vi "RT_SynthFoc.vi"(0 "mode":T4=enum."Full 25 Ch", 2 "Pause?":bool, 3 "Motion Board ID":T6=1 min=1 max=32 step=1, 5 "Scan Axis":u16=3, 8 "Filter":T1, 9 "Qs and Notis":T3, 10 "BKPT Shift":i32, 11 "Raw Name":string="raw", 14 "Trans Geometry (mm)":T2={"Geo Focus"=12.0, "a (radius)"=3.0, "# of rings"=5, "kerf space "=0.1} {"kerf space" format="%.4f"; "a (radius)" format="%.2f"; "Geo Focus" format="%.2f"}) -> (16 "Bd ID Out":T5, 19 "error out":errorcluster)   [LabVIEW 2022 SP3]
uses:
  ScanningControl/Motion Controllers/-MotionRoutines/MotionGlobals.vi
  <vilib>/Motion/FlexMotion/FunctionsVIs/Trajectory.llb/Load Acceleration/Deceleration.flx
  <vilib>/Motion/FlexMotion/CustomControls/CustomControls.llb/Axis To Control.flx
  <vilib>/Motion/FlexMotion/CustomControls/CustomControls.llb/Program.flx
  <instrlib>/niScope/Acquire/Fetch/niScope Multi Fetch Binary 8.vi
  <vilib>/Platform/TimedLoop/XDataNode/XDataNode.xnode
  <vilib>/Platform/TimedLoop/XDataNode/nitl_modes.ctl
  <vilib>/Platform/TimedLoop/XDataNode/XDNodeRunTimeDep.lvlib
  <vilib>/Platform/TimedLoop/XDataNode/wakeup.ctl
  <vilib>/Platform/TimedLoop/XDataNode/timing_clust.ctl
  <vilib>/Motion/FlexMotion/FunctionsVIs/Trajectory.llb/Wait for Move Complete (8 axes).flx
  <vilib>/DAQmx/write.llb/DAQmx Write (Digital 1D Bool NChan 1Samp 1Line).vi
  <vilib>/Motion/FlexMotion/FunctionsVIs/OnboardProgramming.llb/Pause/Resume Program.flx
  RealTimeMode.ctl
  <vilib>/ptbypt/NI_PtbyPt.lvlib
  Annular Array/-SynthApperture/TimeShiftDataI8.vi
  <vilib>/Analysis/NI_AALBase.lvlib
  Annular Array/-SynthApperture/TimeShiftData.vi
  <vilib>/Analysis/baseanly.llb/Mean (DBL).vi
  <instrlib>/niScope/Acquire/niScope Get Scaling Coefficients.vi
  <vilib>/picture/picture.llb/imagedata.ctl
panel:
  out "SF Loop":i32
  out "Read Loop":i32
  out "SF queue":i32
  out "Record queue":i32
  in  "Round to ROC?":bool
  in  "One Way Receive":bool
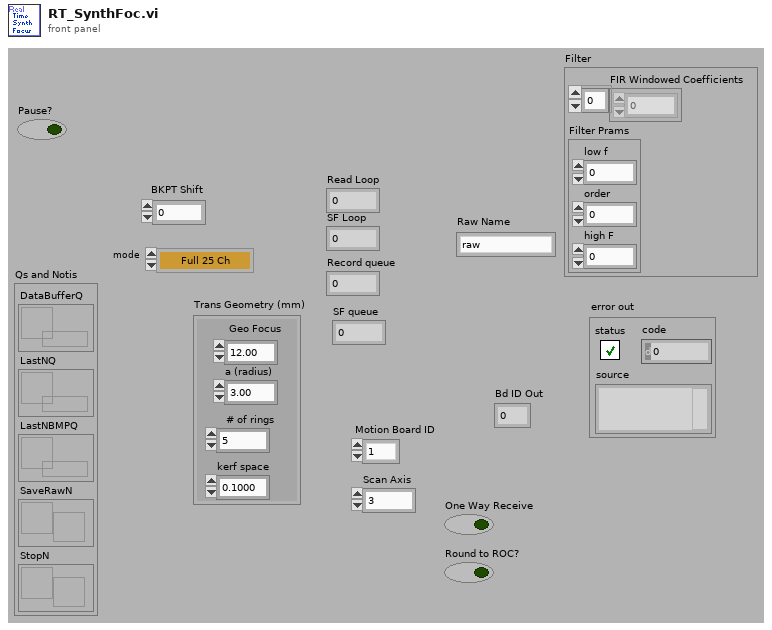
[diagram p1: front panel]
types:
  T1 = cluster{"FIR Windowed Coefficients":dbl[], "Filter Prams":cluster{"low f":i32, "order":i32, "high F":i32}}
  T2 = cluster{"Geo Focus":dbl, "a (radius)":dbl, "# of rings":i32, "kerf space ":dbl}
  T3 = cluster{"DataBufferQ":refnum<queue>, "LastNQ":refnum<queue>, "LastNBMPQ":refnum<queue>, "SaveRawN":refnum<notifier>, "StopN":refnum<notifier>}
  T4 = typedef "RealTimeMode.ctl" = enum16{"1T/5R", "1T/5R Deep Mem", "Full 25 Ch", "Drop Ch 5", "Drop Ch 5,4", "Drop Ch 5,4,3", "Drop Ch 5,4,3,2", "All 25 FIFO CH by CH", "Line by line 2 Ch", "Line by line All", "Deep Memory 2 CH", "Drop Ch 5 (3 Trig)", "test", "Drop Ch 5 XMIT", "Drop Ch 5,4 XMIT", "Drop Ch 5,4,3 XMIT"}
  T5 = typedef "Bd Id Out" = u8
  T6 = typedef "Board Id" = u8
  T7 = cluster{"offset":dbl, "gain":dbl, "reserved 1":dbl, "reserved 2":dbl}[]
  T8 = cluster{"offset":dbl, "gain":dbl, "reserved 1":dbl, "reserved 2":dbl}
  T9 = typedef "location.ctl" = enum16{"Automatic", "WCM Main", "Hawaii", "Columbia MM3000", "Columbia  NI System", "NYU", "RRI 2", "UHI Allen", "CUMC RT", "Chiba", "Stony Brook", "WCM Microscopy", "WCM Aeoretch", "WCM Optics Lab", "WCM Main 2Axis", "WCM Rotation", "WCM SAM SMAC", "SERI GP"}
  T10 = cluster{sgl, "Gain [dB]  ":sgl, "Atten (dB)":sgl}
  T11 = typedef "Program.flx" = u8
  T12 = cluster{"gain":dbl, "wfm":i8[][], bool, "max queue size (-1, unlimited)":i32}
  T13 = typedef "XDNodeRunTimeDep.lvlib/timing_clust.ctl" = cluster{"Expected End [f-1]":u64, "Actual End [f-1]":u64, "Finished Late? [f-1]":bool, "Expected End [i-1]":u64, "Actual End [i-1]":u64, "Finished Late? [i-1]":bool, "Expected Start [i]":u64, "Actual Start [i]":u64, "Expected Start [f]":u64, "Actual Start [f]":u64, "Source Name":string, "Structure Name":string, "Period":i64, "Deadline":i64, "Offset":i64, "Start":i64, "Priority":i32, "Timeout":i32, "Mode":T14, "Wakeup Reason":T15, "Error":errorcluster, "Source Type":string, "Secondary Source Type":string, "Global End Time":u64, "Global Start Time":u64, "Frame Duration":u64, "Iteration Duration":u64, "Assigned CPU":i32, "I/O Scan Engine Mode":u32}
  T14 = typedef "XDNodeRunTimeDep.lvlib/nitl_modes.ctl" = enum32{"No Change", "Process missed periods, maintain original phase", "Discard missed periods, maintain original phase", "Process missed periods, ignore original phase", "Discard missed periods, ignore original phase"}
  T15 = typedef "XDNodeRunTimeDep.lvlib/wakeup.ctl" = enum32{"Normal", "Aborted", "Asynchronous wakeup", "Timing source error", "Timed loop error", "Timeout"}
  T16 = typedef "Axis To Control.flx" = u16
  T17 = cluster{"ZoneStart":sgl[], "ZoneShift":sgl[], "ZoneLength":sgl[]}
  T18 = cluster{"[0]":string, "[1]":string, "[2]":string, "[3]":string, "[4]":string}
  T19 = cluster{"ZoneStart":sgl[], "ZoneShift":sgl[], "ZoneLength":sgl[]}[][]
  T20 = cluster{"ZoneStart":sgl[], "ZoneShift":sgl[], "ZoneLength":sgl[]}[]
  T21 = cluster{"gain":dbl, bool, i16[][], "Sat Pts":i32}
  T22 = cluster{"actualSamples":i32, "absoluteInitialX":dbl, "relativeInitialX":dbl, "xIncrement":dbl, "offset":dbl, "gain":dbl, "reserved1":dbl, "reserved2":dbl}[]
  T23 = cluster{"actualSamples":i32, "absoluteInitialX":dbl, "relativeInitialX":dbl, "xIncrement":dbl, "offset":dbl, "gain":dbl, "reserved1":dbl, "reserved2":dbl}
  T24 = cluster{"gain":dbl, "wfm":i8[][], "Reverse?":bool, i32}
  T25 = cluster{"dig gain":dbl, "Array":i8[][], "Reverse?":bool, i32}
  T26 = cluster{"dig gain":dbl, "Array":i8[][], "Reverse?":bool}
  T27 = typedef "Resource Out (Enum).flx" = u16
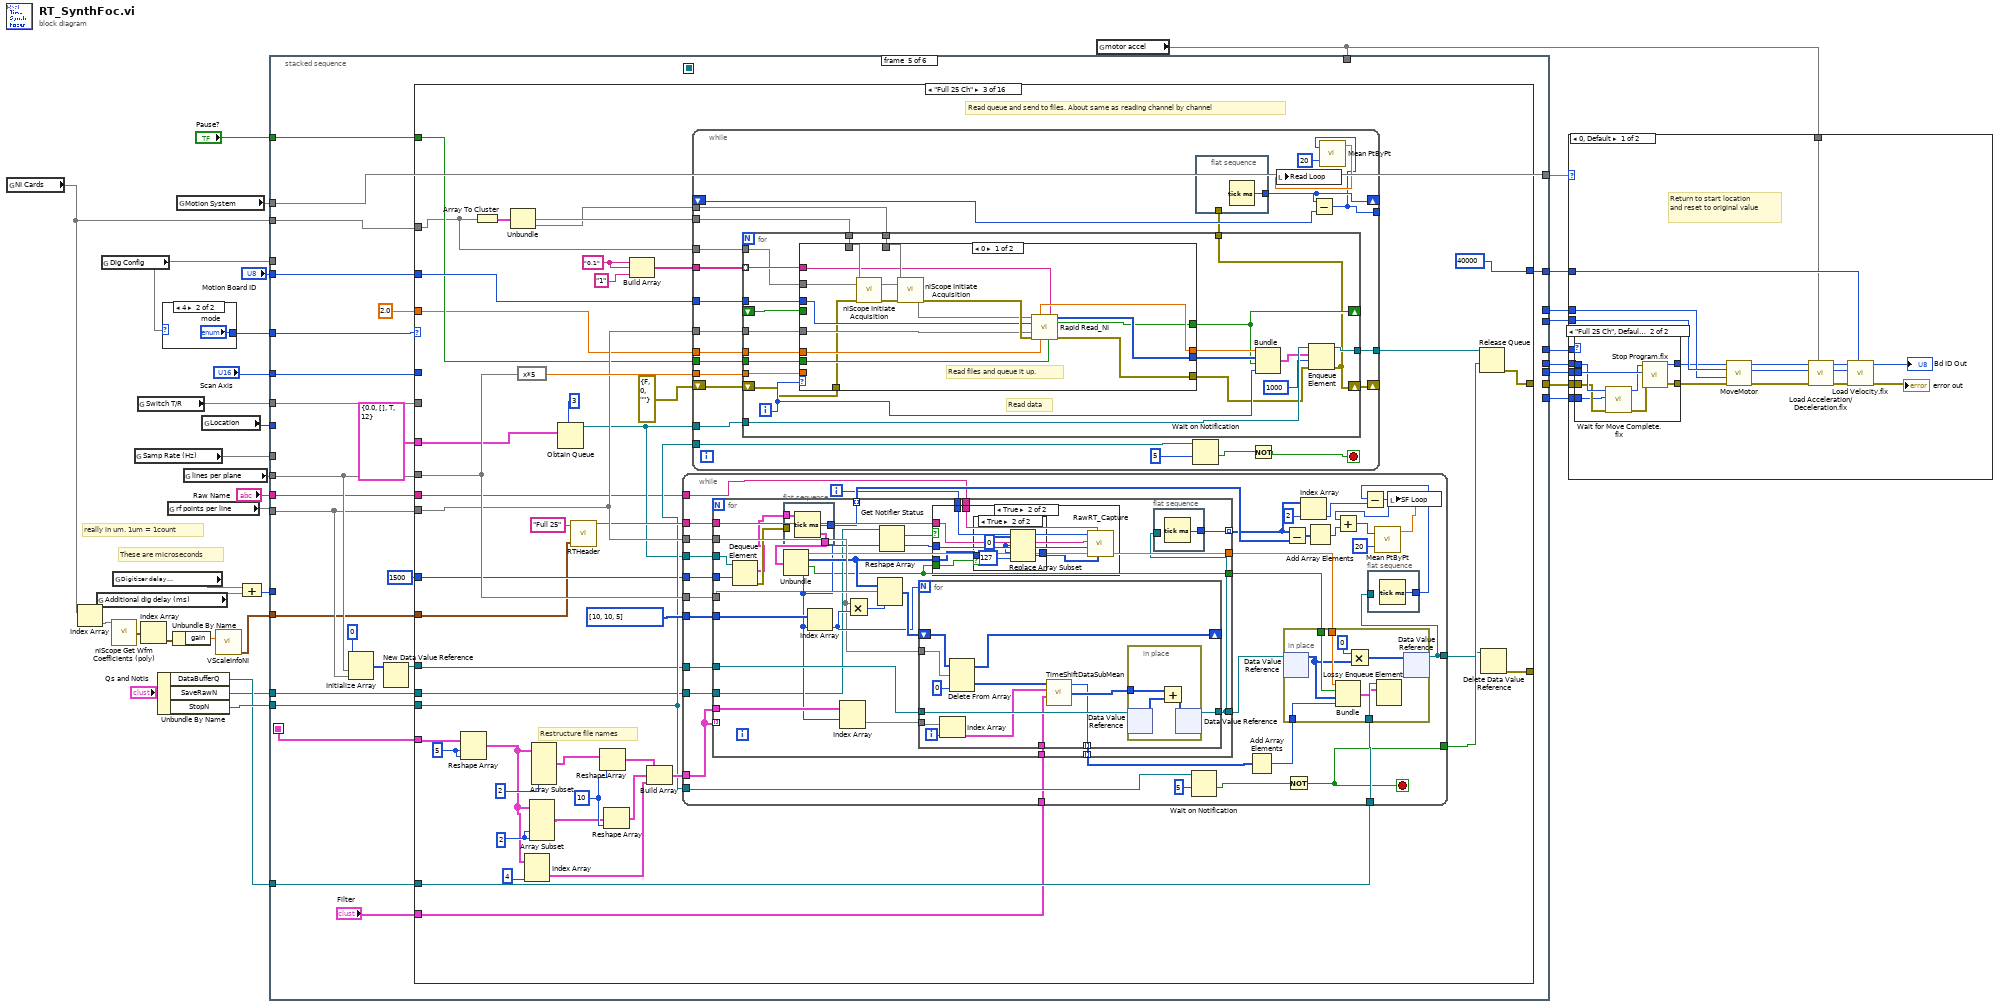
[diagram p0: block diagram]
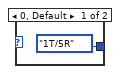
[diagram p4: hidden frame]
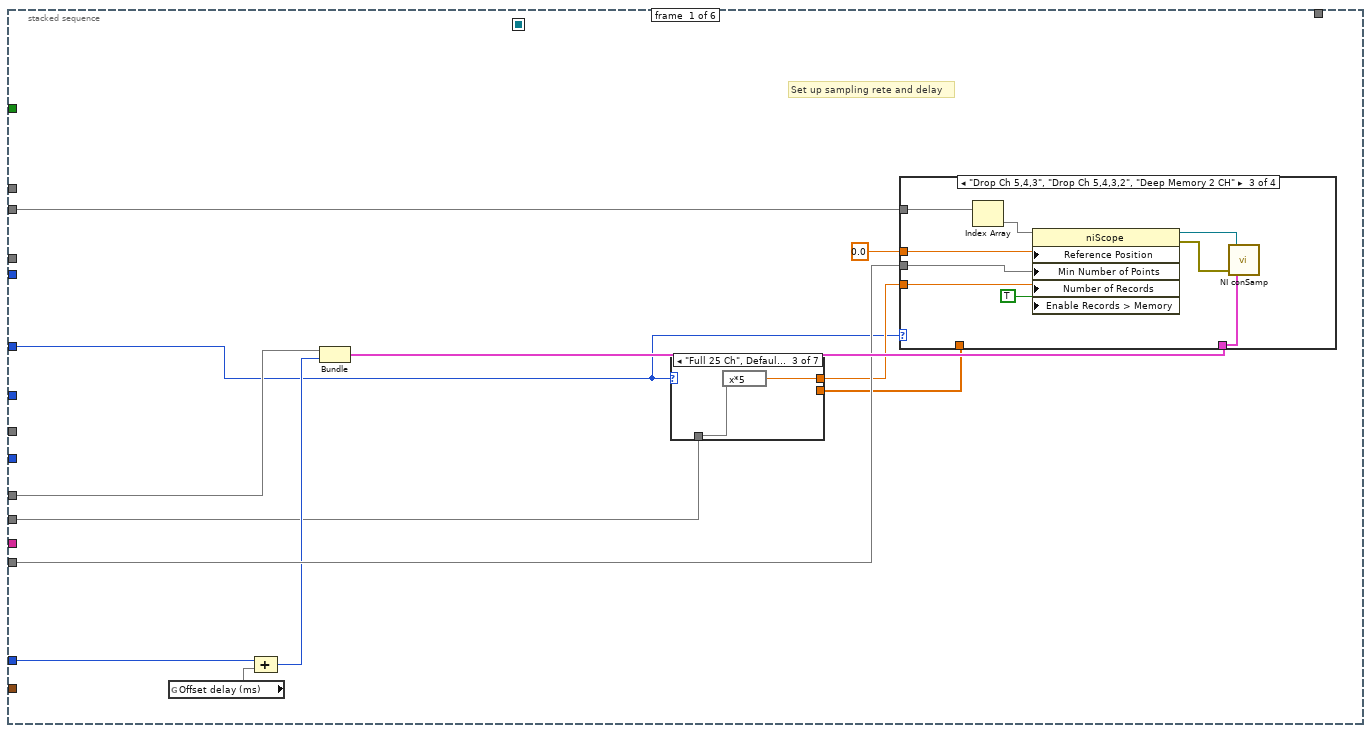
[diagram p5: hidden frame]
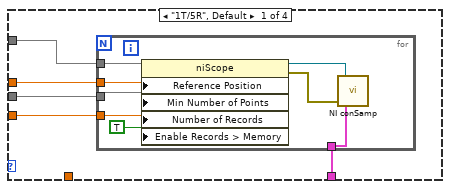
[diagram p6: hidden frame]
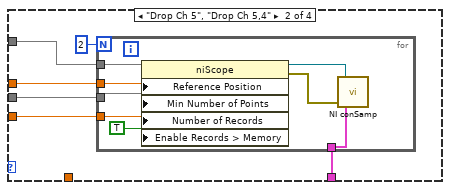
[diagram p7: hidden frame]
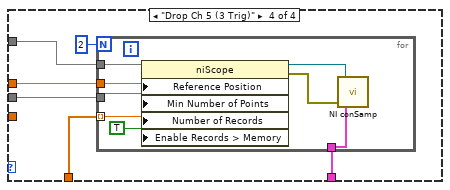
[diagram p8: hidden frame]
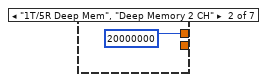
[diagram p10: hidden frame]
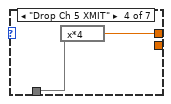
[diagram p11: hidden frame]
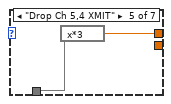
[diagram p12: hidden frame]
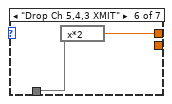
[diagram p13: hidden frame]
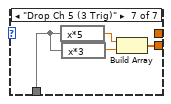
[diagram p14: hidden frame]
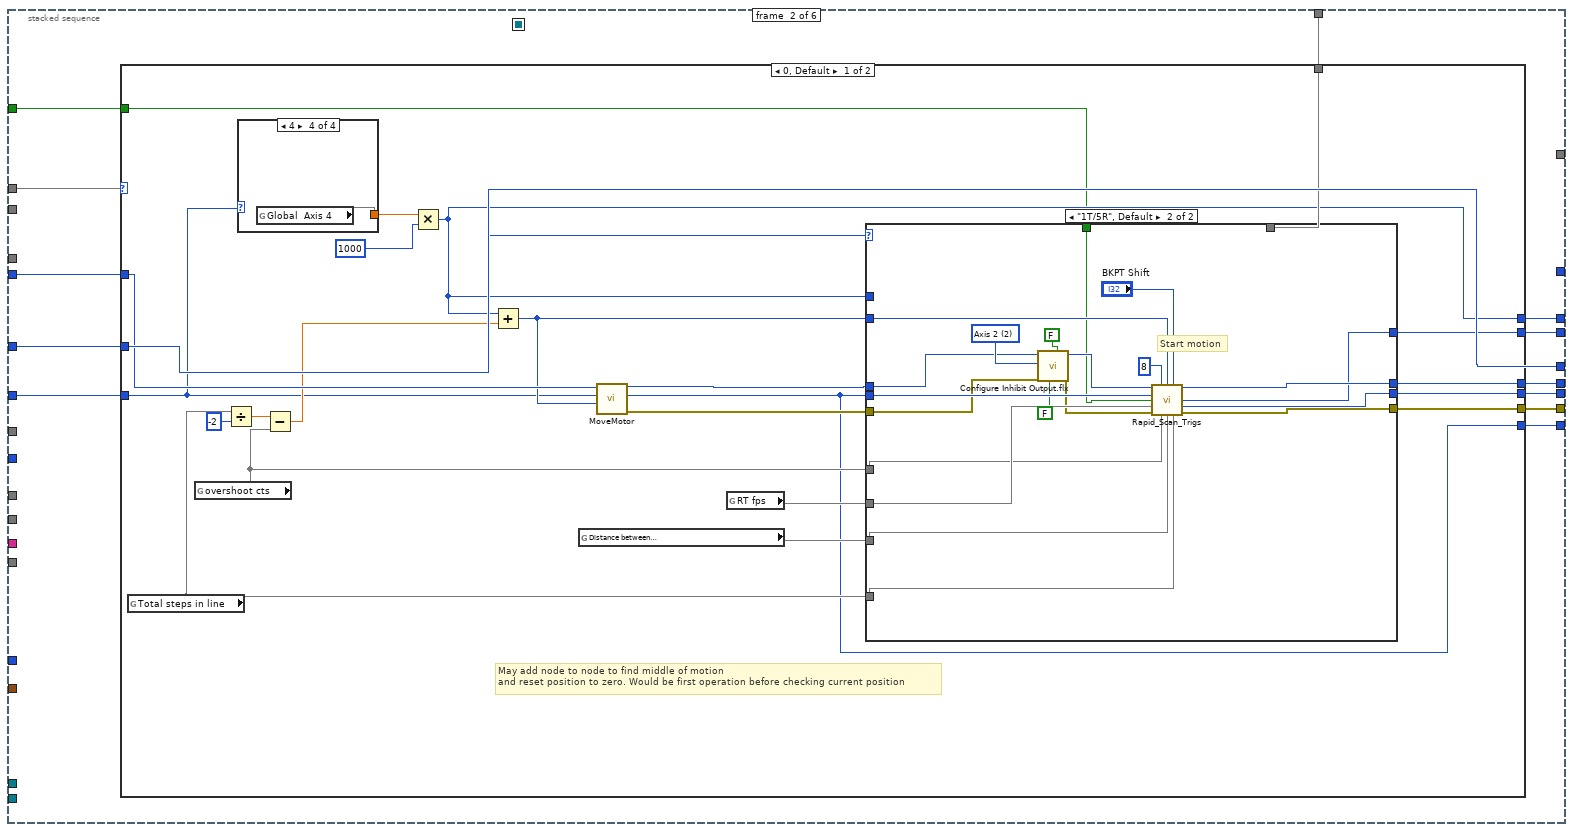
[diagram p15: hidden frame]
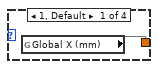
[diagram p16: hidden frame]
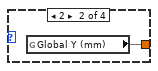
[diagram p17: hidden frame]
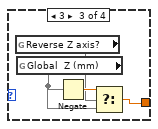
[diagram p18: hidden frame]
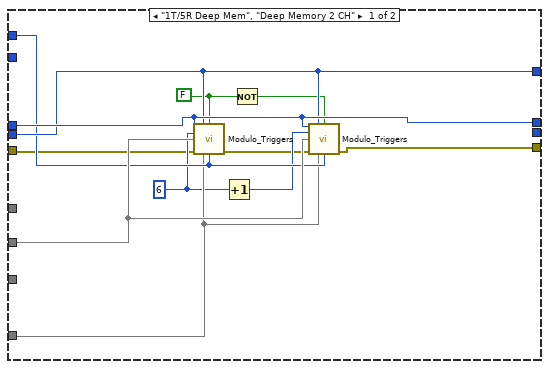
[diagram p19: hidden frame]
diagram:
  # "These are microseconds"
  # "really in um. 1um = 1count"
  n1 = global read "MotionGlobals.vi" "NI Cards"() -> (w1)
  n2 = Index Array(array=w1) -> (element=w4)  [unwired: 1 in]
  n3 = global read "MotionGlobals.vi" "Additional dig delay (ms)"() -> (w24)
  n4 = global read "MotionGlobals.vi" "Dig Config"() -> (w20)
  n5 = call-poly <instrlib>:"niScope Get Wfm Coefficients (poly).vi"("instrument handle"=w4) -> ("coefficient info"=w5:T7)  [unwired: 12 in, 2 out]
  n6 = global read "MotionGlobals.vi" "Digitizer delay\n (ms)"() -> (w25)
  n7 = global read "MotionGlobals.vi" "Samp Rate (Hz)"() -> (w22)
  n8 = global read "MotionGlobals.vi" "Switch T/R"() -> (w8)
  n9 = Index Array(array=w5) -> (element=w6:T8)  [unwired: 1 in]
  n10 = Unbundle By Name("Qs and Notis") -> ("DataBufferQ"=w13:refnum<queue>, "SaveRawN"=w12:refnum<notifier>, "StopN"=w14:refnum<notifier>)
  n11 = case shown="4" w20 {
    tunnel: [RealTimeMode."1T/5R" ("mode") "mode"] -> w21
    frame 0, Default {
    }
    frame 4 {
    }
  }
  n12 = global read "MotionGlobals.vi" "rf points per line"() -> (w34)
  n13 = Unbundle By Name(w6) -> ("gain"=w3:dbl)
  n14 = global read "MotionGlobals.vi" "Motion System"() -> (w19)
  n15 = global read "MotionGlobals.vi" "lines per plane"() -> (w35)
  n16 = global read "MotionGlobals.vi" "Location"() -> (w9:T9)
  n17 = call "VScaleInfoNI.vi"("gain"=w3) -> ("Voltage Scale"=w2:T10)  [unwired: 6 in, 3 out]
  n18 = Compound Arithmetic op=ADD(w25, w24) -> (w23:i32)
  n19 = global read "MotionGlobals.vi" "motor accel"() -> (w26)
  n20 = stacked-sequence {
    seq-local: [_ _ _ w214 _ _] -> [_ _ _ _ w298 _]
    seq-local: [_ _ _ w206 _ _] -> [_ _ _ _ _ w3133]
    tunnel: w35 -> [w41 _ _ _ w291 _]
    tunnel: [_ w125 _ _ _ _] -> w30
    tunnel: [_ w124 _ _ _ _] -> w32
    tunnel: w34 -> [w48 _ _ w219 w283 _]
    tunnel: [_ w123 _ _ _ _] -> w31
    tunnel: [_ w117 _ _ _ _] -> w29
    tunnel: [_ w122 _ _ _ _] -> w33
    tunnel: "Motion Board ID" -> [_ w121 w190 w205 w301 _]
    tunnel: [_ w119 _ _ _ _] -> w28
    tunnel: w21 -> [w40 w119 _ w208 w287 _]
    tunnel: "Scan Axis" -> [_ w118 _ w210 w296 _]
    tunnel: [_ _ _ _ w300 _] -> w27
    tunnel: w26 -> [_ w120 _ _ _ _]
    tunnel: w19 -> [_ w114 w189 w202 w299 _]
    tunnel: [_ _ _ _ w299 _] -> w7
    tunnel: w23 -> [w44 _ _ w217 _ _]
    tunnel: w22 -> [w47 _ _ w218 _ _]
    tunnel: w1 -> [w43 _ _ _ w297 _]
    tunnel: w20 -> [_ _ _ w203 _ w3130]
    tunnel: w14 -> [_ _ _ _ w295 w3131]
    tunnel: w13 -> [_ _ _ _ w294 _]
    tunnel: w9 -> [_ _ w191 _ _ w3132]
    tunnel: "Pause?" -> [_ w116 w188 w209 w289 _]
    tunnel: [_ w115 _ _ _ _] -> w15
    tunnel: w12 -> [_ _ _ _ w285 _]
    tunnel: "Raw Name" -> [_ _ _ _ w284 _]
    tunnel: w8 -> [_ _ _ w204 w282 _]
    tunnel: w2 -> [_ _ _ _ w280 _]
    frame #0 {
      # "Set up sampling rete and delay"
      n21 = global read "MotionGlobals.vi" "Offset delay (ms)"() -> (w46)
      n22 = Compound Arithmetic op=ADD(w44, w46) -> (w45:i32)
      n23 = Bundle("Samp Rate (Hz)"=w47, w45) -> (w49:cluster{"Samp Rate (Hz)":void, i32})  [unwired: 1 out]
      n24 = case shown="\"Full 25 Ch\", Default" w40 {
        tunnel: [w100 20000000 w102 w104 w106 w108 _] -> w42
        tunnel: w41 -> [w100 _ w103 w105 w107 w109 w113]
        tunnel: [_ _ _ _ _ _ w110] -> w39
        frame "1T/5R" {
        }
        frame "1T/5R Deep Mem", "Deep Memory 2 CH" {
        }
        frame "Full 25 Ch", Default {
          n25 = expression code="x*5"(w103) -> (w102:dbl)
        }
        frame "Drop Ch 5 XMIT" {
          n26 = expression code="x*4"(w105) -> (w104:dbl)
        }
        frame "Drop Ch 5,4 XMIT" {
          n27 = expression code="x*3"(w107) -> (w106:dbl)
        }
        frame "Drop Ch 5,4,3 XMIT" {
          n28 = expression code="x*2"(w109) -> (w108:dbl)
        }
        frame "Drop Ch 5 (3 Trig)" {
          n29 = expression code="x*5"(w113) -> (w112:dbl)
          n30 = expression code="x*3"(w113) -> (w111:dbl)
          n31 = Build Array(w112, w111) -> (w110:dbl[])
        }
      }
      n32 = case shown="\"Drop Ch 5,4,3\", \"Drop Ch 5,4,3,2\", \"Deep Memory 2 CH\"" w40 {
        tunnel: w42 -> [w54 w68 w85 _]
        tunnel: w48 -> [w53 w67 w84 w91]
        tunnel: w49 -> [w52 w66 w83 w90]
        tunnel: w43 -> [w51 w65 w81 w89]
        tunnel: 0.0 -> [w50 w64 w82 w88]
        tunnel: w39 -> [_ _ _ w86]
        frame "1T/5R", Default {
          n33 = for {
            tunnel: w54 -> [w57]
            tunnel: w53 -> [w62]
            tunnel: w51 -> [w59]
            tunnel: w52 -> [w58]
            tunnel: w50 -> [w56]
            n34 = property class="niScope"(reference=w59, "Reference Position"=w56, "Min Number of Points"=w62, "Number of Records"=w57, "Enable Records > Memory"=TRUE) -> (reference out=w61:refnum<k15>, error out=w60:errorcluster)  [unwired: 1 in]
            n35 = call "NI conSamp.vi"("error in"=w60, "Sampling"=w58, "InstrumentID"=w61) -> ()  [unwired: 2 out]
          }
        }
        frame "Drop Ch 5", "Drop Ch 5,4" {
          n36 = for {
            N: 2 -> [_]
            tunnel: w68 -> [w71]
            tunnel: w67 -> [w76]
            tunnel: w65 -> [w73]
            tunnel: w66 -> [w72]
            tunnel: w64 -> [w70]
            n37 = property class="niScope"(reference=w73, "Reference Position"=w70, "Min Number of Points"=w76, "Number of Records"=w71, "Enable Records > Memory"=TRUE) -> (reference out=w75:refnum<k15>, error out=w74:errorcluster)  [unwired: 1 in]
            n38 = call "NI conSamp.vi"("error in"=w74, "Sampling"=w72, "InstrumentID"=w75) -> ()  [unwired: 2 out]
          }
        }
        frame "Drop Ch 5,4,3", "Drop Ch 5,4,3,2", "Deep Memory 2 CH" {
          n39 = Index Array(array=w81) -> (element=w77)  [unwired: 1 in]
          n40 = property class="niScope"(reference=w77, "Reference Position"=w82, "Min Number of Points"=w84, "Number of Records"=w85, "Enable Records > Memory"=TRUE) -> (reference out=w80:refnum<k15>, error out=w79:errorcluster)  [unwired: 1 in]
          n41 = call "NI conSamp.vi"("error in"=w79, "Sampling"=w83, "InstrumentID"=w80) -> ()  [unwired: 2 out]
        }
        frame "Drop Ch 5 (3 Trig)" {
          n42 = for {
            N: 2 -> [_]
            tunnel: w86 -> [w94] mode=indexing
            tunnel: w91 -> [w99]
            tunnel: w89 -> [w96]
            tunnel: w90 -> [w95]
            tunnel: w88 -> [w93]
            n43 = property class="niScope"(reference=w96, "Reference Position"=w93, "Min Number of Points"=w99, "Number of Records"=w94, "Enable Records > Memory"=TRUE) -> (reference out=w98:refnum<k15>, error out=w97:errorcluster)  [unwired: 1 in]
            n44 = call "NI conSamp.vi"("error in"=w97, "Sampling"=w95, "InstrumentID"=w98) -> ()  [unwired: 2 out]
          }
        }
      }
    }
    frame #1 {
      n45 = case shown="0, Default" w114 {
        tunnel: [w148 _] -> w125
        tunnel: [w147 _] -> w124
        tunnel: [w145 _] -> w123
        tunnel: [w144 _] -> w122
        tunnel: w121 -> [w141 _]
        tunnel: w120 -> [w139 _]
        tunnel: w119 -> [w137 _]
        tunnel: w118 -> [w136 _]
        tunnel: [w134 _] -> w117
        tunnel: w116 -> [w127 _]
        tunnel: [w126 _] -> w115
        frame 0, Default {
          # "May add node to node to find middle of motion\nand reset position to zero. Would be first operation before checking current position"
          n46 = global read "MotionGlobals.vi" "Total steps in line"() -> (w143)
          n47 = global read "MotionGlobals.vi" "overshoot cts"() -> (w131)
          n48 = Divide(x=w143, y=-2) -> (x/y=w142:dbl)
          n49 = case shown="4" w136 {
            tunnel: [w149 w150 w151 w155] -> w135
            frame 1, Default {
              n50 = global read "MotionGlobals.vi" "Global X (mm)"() -> (w149)
            }
            frame 2 {
              n51 = global read "MotionGlobals.vi" "Global Y (mm)"() -> (w150)
            }
            frame 3 {
              n52 = global read "MotionGlobals.vi" "Reverse Z axis?"() -> (w152)
              n53 = global read "MotionGlobals.vi" "Global  Z (mm)"() -> (w153)
              n54 = Negate(x=w153) -> (-x=w154:dbl)
              n55 = Select(t=w154, s=w152, f=w153) -> (s? t:f=w151:dbl)
            }
            frame 4 {
              n56 = global read "MotionGlobals.vi" "Global  Axis 4"() -> (w155)
            }
          }
          n57 = Subtract(x=w142, y=w131) -> (x-y=w140:dbl)
          n58 = Multiply(x=w135, y=1000) -> (x*y=w134:i32)
          n59 = Add(x=w134, y=w140) -> (x+y=w138:i32)
          n60 = global read "MotionGlobals.vi" "Distance between\nscan lines (mm)"() -> (w129)
          n61 = call "MoveMotor.vi"("Target Position (0)"=w138, "Axis or Vector Space"=w136, "Motion Bd ID"=w141) -> ("error out"=w133:errorcluster, "Resource Output"=w126:u16, "Bd ID Out"=w132:u8)  [unwired: 2 in, 4 out]
          n62 = global read "MotionGlobals.vi" "RT fps"() -> (w128)
          n63 = case shown="\"1T/5R\", Default" w137 {
            tunnel: w128 -> [w165 w187]
            tunnel: [w156 w186] -> w148
            tunnel: [w167 w185] -> w147
            tunnel: [_ w184] -> w145
            tunnel: [w166 w183] -> w144
            tunnel: w143 -> [w163 w182]
            tunnel: w129 -> [_ w169]
            tunnel: w131 -> [_ w181]
            tunnel: w132 -> [w167 w172]
            tunnel: w126 -> [w166 w180]
            tunnel: w133 -> [w157 w171]
            tunnel: w138 -> [_ w179]
            tunnel: w134 -> [w164 _]
            tunnel: w139 -> [_ _]
            tunnel: w127 -> [_ w170]
            frame "1T/5R Deep Mem", "Deep Memory 2 CH" {
              w159 = T11 6 ("Program (1)")
              w162 = FALSE
              n64 = call "Modulo_Triggers.vi"("Motion Settings In"=w167, "Axis"=w166, "Reverse ?"=w162, "Program (1)"=w159, 7:w165, "error in (no error)"=w157, 12:w163, "Offset"=w164) -> ("error out"=w158:errorcluster)  [unwired: 1 in, 6 out]
              n65 = Increment(x=w159) -> (x+1=w160:T11)
              n66 = Not(x=w162) -> (.not. x?=w161:bool)
              n67 = call "Modulo_Triggers.vi"("Motion Settings In"=w167, "Axis"=w166, "Reverse ?"=w161, "Program (1)"=w160, 7:w165, "error in (no error)"=w158, 12:w163, "Offset"=w164) -> ("error out"=w156:errorcluster)  [unwired: 1 in, 6 out]
            }
            frame "1T/5R", Default {
              w174 = T16 2 items=["Axis 1"=1, "Axis 2"=2, "Axis 3"=3, "Axis 4"=4, "Axis 5"=5, "Axis 6"=6, "Axis 7"=7, "Axis 8"=8] ("Axis")
              # "Start motion"
              n68 = call <vilib>:"Configure Inhibit Output.flx"("Enable"=FALSE, "Polarity (Active Low)"=FALSE, "error in (no error)"=w171, "Axis"=w174, "Board ID"=w172) -> ("error out"=w177:errorcluster, "Bd ID Out"=w178:T5)  [unwired: 1 in, 4 out]
              n69 = call "Rapid_Scan_Trigs.vi"("Board ID"=w178, "Program (1)"=T11 8, "Start Position"=w179, "BKPT Shift"="BKPT Shift", "Scan Axis"=w180, "Pause?"=w170, "# frames/ s"=w187, "error in (no error)"=w177, "overshoot"=w181, "step interval"=w169, "Total Steps (one way)"=w182) -> ("Bd ID Out"=w185:u8, "Axis Resource out"=w183:u16, "Program ID"=w184:u8, "error out"=w186:errorcluster)  [unwired: 1 out]
            }
          }
        }
        frame 8 {
        }
      }
    }
    frame #2 {
      n70 = case shown="0, Default" w189 {
        tunnel: w190 -> [w197 _]
        frame 0, Default {
          n71 = call "CheckLimStat.vi"("Motion Board ID"=w197) -> ()
        }
        frame 1, 7, 8 {
        }
      }
      n72 = case shown="\"Hawaii\", Default" w191 {
        tunnel: w188 -> [_ w192]
        frame "UHI Allen", "CUMC RT" {
        }
        frame "Hawaii", Default {
          n73 = case shown="False" w192 {
            tunnel: [bool[] [FALSE, TRUE] ("data") bool[] [TRUE, FALSE] ("data")] -> w193
            frame False {
              # "turn on gated RT trig"
            }
            frame True {
              # "turn on motion trig"
            }
          }
          n74 = call-poly <vilib>:"DAQmx Write.vi"("task/channels in"=refnum<k21> "DIO-L2 L3", "data"=w193) -> ()  [unwired: 11 in, 3 out]
        }
      }
    }
    frame #3 {
      n75 = case shown="True" w209 {
        tunnel: w205 -> [_ w251]
        frame False {
        }
        frame True {
          w252 = T11 11 ("Program (1)")
          n76 = call <vilib>:"Begin Program Storage.flx"("Program (1)"=w252, "Board ID"=w251) -> ("error out"=w256:errorcluster, "Bd ID Out"=w257:T5)  [unwired: 4 in, 1 out]
          n77 = call "Pause/Resume Program.flx"("error in (no error)"=w256, "Program (1)"=T11 8, "Board ID"=w257) -> ("error out"=w254:errorcluster, "Bd ID Out"=w255:T5)  [unwired: 3 in, 1 out]
          n78 = call <vilib>:"End Program Storage.flx"("error in (no error)"=w254, "Program (1)"=w252, "Board ID"=w255) -> ()  [unwired: 3 in, 3 out]
        }
      }
      n79 = Decrement(x=w204) -> (x-1=w207:dbl)
      n80 = case shown="4" w203 {
        tunnel: w210 -> [_ w228]
        tunnel: w208 -> [_ w227]
        tunnel: w207 -> [_ w226]
        tunnel: [_ w225] -> w206
        tunnel: w205 -> [_ w221]
        tunnel: w202 -> [_ w220]
        frame 0, Default {
        }
        frame 4 {
          # "Arm all counters"
          n81 = call "5ChPulserTrigsNew.vi"("Motion Settings"=w221, 4:w226, "Digitizer Settings"=w227, "Axis"=w228) -> ("5CH Pulser Tasks"=w225:refnum<k21>[])  [unwired: 5 in, 1 out]
          n82 = for {
            tunnel: w225 -> [w235] mode=indexing
            tunnel: [w234] -> w223
            n83 = call <vilib>:"DAQmx Start Task.vi"("task/channels in"=w235) -> ("error out"=w234:errorcluster)  [unwired: 1 in, 13 out]
          }
          n84 = for {
            tunnel: bool[][] [[TRUE], [FALSE]] ("data") -> [w237] mode=indexing
            tunnel: w223 -> [_]
            tunnel: [w236] -> w222
            n85 = flat-sequence {
              tunnel: w237 -> [w240]
              tunnel: [w240] -> w238
              tunnel: w238 -> [w242]
              tunnel: [w241] -> w236
              frame #0 {
                n86 = Wait (ms)(milliseconds to wait=u32 25) -> ()  [unwired: 1 out]
              }
              frame #1 {
                n87 = call "DAQ Assistant"("data"=w242) -> ("error out"=w241:errorcluster)  [unwired: 17 in, 1 out]
              }
            }
          }
          n88 = case shown="0, Default" w220 {
            tunnel: w222 -> [w230 _]
            tunnel: w221 -> [w229 _]
            frame 0, Default {
              # "Prep Counters"
              n89 = for {
                N: 4 -> [_]
                tunnel: w229 -> [w233]
                tunnel: w230 -> [w232]
                n90 = call "ForceBreakPt.vi"("error in"=w232, "Bd ID in"=w233) -> ()  [unwired: 2 out]
              }
            }
            frame 8 {
            }
          }
        }
      }
      n91 = case shown="\"Full 25 Ch\", Default" w208 {
        tunnel: [w245 25] -> w213
        tunnel: [w244 u32 0] -> w212
        tunnel: w207 -> [w243 _]
        frame "1T/5R", "1T/5R Deep Mem" {
          w245 = 5
          n92 = In Range and Coerce(upper limit=u32 0, x=w243, lower limit=u32 4) -> (coerced(x)=w248:u32)  [unwired: 1 out]
          n93 = Multiply(x=w248, y=w245) -> (x*y=w244:i32)
        }
        frame "Full 25 Ch", Default {
        }
      }
      n94 = global read "MotionGlobals.vi" "c mm/mics"() -> (w211:sgl)
      n95 = global read "MotionGlobals.vi" "Tansducer"() -> (w199)
      n96 = call "F-Zones.vi"(7:"Trans Geometry (mm)", 11:w199) -> ("ROC (m)"=w200:dbl, "annuli rad (m)"=w201:dbl[])  [unwired: 6 in, 2 out]
      n97 = for {
        N: w213 -> [_]
        tunnel: w219 -> [w274]
        tunnel: w211 -> [w267]
        tunnel: w218 -> [w262]
        tunnel: w217 -> [w273]
        tunnel: "One Way Receive" -> [w272]
        tunnel: "Round to ROC?" -> [w271]
        tunnel: [w269] -> w214 mode=indexing
        tunnel: w212 -> [w264]
        tunnel: w201 -> [w259]
        tunnel: w200 -> [w258]
        i -> [w263]
        # "Added delay when Ch1 triggered from different hardware card."
        n98 = Multiply(x=w267, y=1000) -> (x*y=w268:sgl)
        n99 = Add(x=w263, y=w264) -> (x+y=w265:u32)
        n100 = Divide(x=w267, y=2) -> (x/y=w277:sgl)
        n101 = Multiply(x=w273, y=w277) -> (x*y=w266:sgl)
        n102 = global read "MotionGlobals.vi" "F Zones"() -> (w276)
        n103 = call "CalcFZones.vi"("F- zones"=w276, "delay (mm)"=w266, "Round to ROC?"=w271, "One Way Receive"=w272, "# rf points per line"=w274, "Radii (m)"=w259, "ROC (m)"=w258, "Sampling Rate"=w262, "c (m/s)"=w268, "File index number"=w265) -> ("ZoneStart"=w261:sgl[], "ZoneShift"=w260:sgl[], "ZoneLength"=w270:sgl[])  [unwired: 3 out]
        n104 = Bundle("ZoneStart"=w261, "ZoneShift"=w260, "ZoneLength"=w270) -> (w269:T17)  [unwired: 1 in]
      }
    }
    frame #4 {
      n105 = Initialize Array(i16 0, w291, w283) -> (w292:i16[][])
      n106 = New Data Value Reference(data value=w292) -> (data value reference=w290:refnum<data-value>)  [unwired: 1 in, 1 out]
      n107 = case shown="\"Full 25 Ch\"" w287 {
        tunnel: [40000 40000 40000 40000 40000 40000 40000 40000 40000 40000 40000 40000 40000 40000 40000 40000] -> w300
        tunnel: w301 -> [w346 w537 w691 w918 w1139 w1359 w1575 w1789 w2004 w2211 w2352 w2477 w2644 w2720 w2814 w2990]
        tunnel: w291 -> [w320 w533 w716 w942 w1163 w1383 w1599 w1774 w1989 w2209 w2350 w2478 w2645 w2721 w2793 w2971]
        tunnel: w283 -> [w345 w534 w701 w929 w1150 w1370 w1586 w1776 w1991 w2200 w2342 w2475 w2633 w2713 w2795 w2977]
        tunnel: w298 -> [w340 w528 w721 w947 w1168 w1388 w1604 w1792 w2008 w2214 w2355 w2482 w2636 w2722 w2799 w2994]
        tunnel: w297 -> [w333 w503 w680 w919 w1140 w1360 w1576 w1765 w1979 w2194 w2336 w2466 w2626 w2711 w2779 w2965]
        tunnel: w296 -> [_ w515 _ _ _ _ _ _ _ w2190 w2332 _ _ _ w2808 _]
        tunnel: w295 -> [w328 w505 w697 w925 w1146 w1366 w1582 w1769 w1982 w2192 w2335 w2471 w2630 w2715 w2785 w2968]
        tunnel: w294 -> [w329 w507 w696 w924 w1145 w1365 w1581 w1770 w1983 w2198 w2340 w2472 w2631 w2716 w2786 w2969]
        tunnel: w290 -> [_ _ w695 w923 w1144 w1364 w1580 w1767 w1981 w2196 w2338 w2468 w2628 w2712 w2781 w2967]
        tunnel: w289 -> [w319 _ w686 w913 w1134 w1354 w1570 w1761 w1975 w2188 w2333 w2460 w2624 w2710 _ w2960]
        tunnel: [_ _ w689 w916 w1137 w1357 w1573 _ _ _ _ _ _ _ _ _] -> _
        tunnel: [_ _ w688 w915 w1136 w1356 w1572 _ _ _ _ _ _ _ _ _] -> _
        tunnel: 1500 -> [w304 w504 w687 w914 w1135 w1355 w1571 w1760 w1976 w2189 w2331 w2461 _ _ w2777 w2961]
        tunnel: 2.0 ("timeout") -> [w318 w501 w685 w912 w1133 w1353 w1568 w1759 w1967 w2187 w2323 w2459 _ _ _ _]
        tunnel: w285 -> [w317 _ w684 w911 w1132 w1352 w1566 w1758 w1966 w2185 w2322 _ _ _ _ _]
        tunnel: w284 -> [w314 _ w683 w910 w1131 w1351 w1567 w1757 w1965 w2183 w2321 _ _ _ _ _]
        tunnel: w282 -> [w313 _ _ _ _ _ _ _ _ _ _ _ _ _ _ _]
        tunnel: T12 {"gain"=0.0, "wfm"=[], TRUE, "max queue size (-1, unlimited)"=12} -> [_ _ w682 w904 w1125 w1345 w1565 w1754 w1962 _ _ _ _ _ _ w2959]
        tunnel: w280 -> [w303 _ w679 w903 w1124 w1344 w1564 w1753 w1961 w2182 w2318 _ _ _ _ _]
        tunnel: "Filter" -> [w302 _ w678 w902 w1123 w1343 w1563 w1752 w1960 w2181 w2317 w2458 w2623 _ _ w2958]
        frame "1T/5R", Default {
          # "1T/5R flip flop version"
          n108 = Array To Cluster(array=w333) -> (cluster=w332:cluster{"[0]":void, "[1]":void, "[2]":void})
          n109 = Unbundle(w332) -> ("[0]"=w330, "[1]"=w326, "[2]"=w323)
          n110 = for {
            N: 5 -> [_]
            tunnel: w313 -> [w359]
            tunnel: [w356] -> w311 mode=indexing
            i -> [w358]
            n111 = Increment(x=w358) -> (x+1=w357:i32)
            n112 = Format Into String(initial string="_%d to %d", w359, w357) -> (resulting string=w356:string)  [unwired: 2 in, 1 out]
          }
          n113 = Obtain Queue(max queue size (-1, unlimited)=2, element data type=cluster{"gain":dbl, bool} {"gain"=0.0, TRUE}) -> (queue out=w353:refnum<queue>)  [unwired: 2 in, 3 out]
          n114 = Index Array(array=w340) -> (element=w337:T17)  [unwired: 1 in]
          n115 = Index Array(array=w340, index=1) -> (element=w336:T17)
          n116 = Index Array(array=w340, index=2) -> (element=w335:T17)
          n117 = Index Array(array=w340, index=3) -> (element=w338:T17)
          n118 = Index Array(array=w340, index=4) -> (element=w339:T17)
          n119 = Obtain Queue(max queue size (-1, unlimited)=5, element data type=i8[][] [] ("Array")) -> (queue out=w347:refnum<queue>)  [unwired: 2 in, 3 out]
          n120 = Array To Cluster(array=w311) -> (cluster=w310:T18)
          n121 = property class="niScope"(reference=w326, "Fetch Record Number"=0, "Fetch Number of Records"=w320) -> (reference out=w325:refnum<k15>)  [unwired: 1 in, 1 out]
          n122 = call "RTHeader.vi"("Comment"="1T, 5RCV", "Votage scaling"=w303) -> ("Header String Out"=w315:string)  [unwired: 4 in, 1 out]
          n123 = Unbundle(w310) -> ("[0]"=w309:string, "[1]"=w308:string, "[2]"=w307:string, "[3]"=w306:string, "[4]"=w305:string)
          n124 = while {
            tunnel: w353 -> [w411]
            tunnel: [w401] -> w352
            tunnel: [w417] -> w351
            tunnel: w347 -> [w412]
            tunnel: w339 -> [w424]
            tunnel: w338 -> [w423]
            tunnel: w337 -> [w422]
            tunnel: w336 -> [w421]
            tunnel: w335 -> [w420]
            tunnel: [w408] -> w334
            tunnel: w329 -> [w419]
            tunnel: w328 -> [w400]
            tunnel: w304 -> [w398]
            tunnel: w317 -> [w382]
            tunnel: w315 -> [w374]
            tunnel: w314 -> [w373]
            tunnel: w309 -> [w366]
            tunnel: w308 -> [w365]
            tunnel: w307 -> [w364]
            tunnel: w306 -> [w363]
            tunnel: w305 -> [w362]
            tunnel: w302 -> [w361]
            i -> [w375]
            stop <- w401 stop-if-true
            # "Dequeue data and synth focus"
            n125 = Get Notifier Status(notifier=w382) -> (current notification=w381:bool)  [unwired: 1 in, 4 out]
            n126 = Dequeue Element(queue=w411, timeout in ms (-1)=w398) -> (queue out=w417:refnum<queue>, element=w428:cluster{"gain":dbl, bool}, error out=w385:errorcluster)  [unwired: 1 in, 1 out]
            n127 = Dequeue Element(queue=w412, timeout in ms (-1)=w398, error in (no error)=w384) -> (queue out=w390:refnum<queue>, element=w380:i8[][], error out=w416:errorcluster)  [unwired: 1 out]
            n128 = flat-sequence {
              tunnel: [w443] -> w389
              tunnel: w385 -> [w442]
              tunnel: [w442] -> w384
              frame #0 {
                n129 = Tick Count (ms)() -> (millisecond timer value=w443:u32)
              }
            }
            n130 = call "TimeShiftDataSubMean.vi"("Filter"=w361, "output cluster"=w422, "Array In"=w380) -> ("Array Out"=w406:i16[][], "Sat Pts"=w372:i32)  [unwired: 2 in]
            n131 = Dequeue Element(queue=w390, timeout in ms (-1)=w398, error in (no error)=w416) -> (queue out=w427:refnum<queue>, element=w379:i8[][], error out=w415:errorcluster)  [unwired: 1 out]
            n132 = call "TimeShiftDataSubMean.vi"("Filter"=w361, "output cluster"=w421, "Array In"=w379) -> ("Array Out"=w383:i16[][], "Sat Pts"=w371:i32)  [unwired: 2 in]
            n133 = Dequeue Element(queue=w427, timeout in ms (-1)=w398, error in (no error)=w415) -> (queue out=w426:refnum<queue>, element=w378:i8[][], error out=w414:errorcluster)  [unwired: 1 out]
            n134 = call "TimeShiftDataSubMean.vi"("Filter"=w361, "output cluster"=w420, "Array In"=w378) -> ("Array Out"=w394:i16[][], "Sat Pts"=w370:i32)  [unwired: 2 in]
            n135 = Dequeue Element(queue=w426, timeout in ms (-1)=w398, error in (no error)=w414) -> (queue out=w425:refnum<queue>, element=w377:i8[][], error out=w413:errorcluster)  [unwired: 1 out]
            n136 = call "TimeShiftDataSubMean.vi"("Filter"=w361, "output cluster"=w423, "Array In"=w377) -> ("Array Out"=w393:i16[][], "Sat Pts"=w369:i32)  [unwired: 2 in]
            n137 = Dequeue Element(queue=w425, timeout in ms (-1)=w398, error in (no error)=w413) -> (queue out=w409:refnum<queue>, element=w376:i8[][], error out=w410:errorcluster)  [unwired: 1 out]
            n138 = case shown="True" w381 {
              tunnel: w380 -> [_ w441]
              tunnel: w379 -> [_ w440]
              tunnel: w378 -> [_ w439]
              tunnel: w377 -> [_ w438]
              tunnel: w376 -> [_ w437]
              tunnel: w375 -> [_ w435]
              tunnel: w374 -> [_ w436]
              tunnel: w373 -> [_ w434]
              tunnel: w366 -> [_ w433]
              tunnel: w365 -> [_ w432]
              tunnel: w364 -> [_ w431]
              tunnel: w363 -> [_ w430]
              tunnel: w362 -> [_ w429]
              frame False {
              }
              frame True {
                n139 = call "RawRT_Capture.vi"("Raw data"=w441, "File Name In"=w434, "Add Text"=w433, "header"=w436, "Iter"=w435) -> ()  [unwired: 7 in]
                n140 = call "RawRT_Capture.vi"("Raw data"=w440, "File Name In"=w434, "Add Text"=w432, "header"=w436, "Iter"=w435) -> ()  [unwired: 7 in]
                n141 = call "RawRT_Capture.vi"("Raw data"=w439, "File Name In"=w434, "Add Text"=w431, "header"=w436, "Iter"=w435) -> ()  [unwired: 7 in]
                n142 = call "RawRT_Capture.vi"("Raw data"=w438, "File Name In"=w434, "Add Text"=w430, "header"=w436, "Iter"=w435) -> ()  [unwired: 7 in]
                n143 = call "RawRT_Capture.vi"("Raw data"=w437, "File Name In"=w434, "Add Text"=w429, "header"=w436, "Iter"=w435) -> ()  [unwired: 7 in]
              }
            }
            n144 = Unbundle(w428) -> ("gain"=w404:dbl, w418:bool)
            n145 = call "TimeShiftDataSubMean.vi"("Filter"=w361, "output cluster"=w424, "Array In"=w376) -> ("Array Out"=w392:i16[][], "Sat Pts"=w368:i32)  [unwired: 2 in]
            n146 = Compound Arithmetic op=ADD(w383, w394, w393, w392) -> (w391:i16[][])
            n147 = Get Queue Status(queue=w409, error in (no error)=w410) -> (queue out=w408:refnum<queue>, # elements in queue=w407:i32)  [unwired: 1 in, 6 out]
            n148 = local write "SF queue"(w407) -> ()
            n149 = expression code="x*2"(w391) -> (w405:i16[][])
            n150 = Compound Arithmetic op=ADD(w368, w372, w371, w370, w369) -> (w367:i32)
            n151 = Add(x=w406, y=w405) -> (x+y=w395:i16[][])
            n152 = Wait on Notification(notifier=w400, timeout in ms (-1)=5) -> (timed out?=w399:bool)  [unwired: 2 in, 3 out]
            n153 = Not(x=w399) -> (.not. x?=w401:bool)
            n154 = Bundle("gain"=w404, w418, w395, w367) -> (w403:cluster{"gain":dbl, bool, i16[][], i32})  [unwired: 1 in]
            n155 = Lossy Enqueue Element(queue=w419, element=w403) -> (error out=w397:errorcluster)  [unwired: 1 in, 3 out]
            n156 = stacked-sequence {
              tunnel: [w444] -> w396
              tunnel: w397 -> [_]
              frame #0 {
                n157 = Tick Count (ms)() -> (millisecond timer value=w444:u32)
              }
            }
            n158 = Subtract(x=w396, y=w389) -> (x-y=w387:u32)
            n159 = call <vilib>:"Mean PtByPt.vi"("x"=w387, "sample length"=20) -> ("mean"=w386:dbl)  [unwired: 2 in, 1 out]
            n160 = local write "SF Loop"(w386) -> ()
          }
          n161 = property class="niScope"(reference=w323, "Fetch Record Number"=0, "Fetch Number of Records"=w320) -> (reference out=w322:refnum<k15>)  [unwired: 1 in, 1 out]
          n162 = while {
            tunnel: w345 -> [w482]
            tunnel: w346 -> [w455]
            tunnel: w353 -> [w488]
            tunnel: w330 -> [w461]
            tunnel: w347 -> [w470]
            tunnel: w328 -> [w459]
            tunnel: w325 -> [w457]
            tunnel: w322 -> [w456]
            tunnel: [w454] -> w321
            tunnel: w319 -> [w453]
            shift-right: [w450] -> _
            shift-left: _ -> [w451]
            tunnel: w318 -> [w446]
            tunnel: w304 -> [w445]
            stop <- w454 stop-if-true
            # "Get next available frame and queue data"
            n163 = call <instrlib>:"niScope Initiate Acquisition.vi"("instrument handle"=w457) -> ("instrument handle out"=w473:refnum<k15>, "error out"=w474:errorcluster)  [unwired: 2 in, 11 out]
            n164 = call <instrlib>:"niScope Initiate Acquisition.vi"("instrument handle"=w456, "error in"=w474) -> ("instrument handle out"=w472:refnum<k15>, "error out"=w483:errorcluster)  [unwired: 1 in, 11 out]
            n165 = call "Rapid Read_NI.vi"("NI Card"=w461, "Channel"="0", "Motion Board ID"=w455, "rf points per line"=w482, "error in"=w483, "timeout"=w446, "Pause?"=w453) -> ("dig gain"=w485:dbl, "Array"=w468:i8[][], "Reverse?"=w487:bool, "error out"=w463:errorcluster)  [unwired: 5 in]
            n166 = Bundle("dig gain"=w485, "Reverse?"=w487) -> (w486:cluster{"dig gain":dbl, "Reverse?":bool})  [unwired: 1 out]
            n167 = Enqueue Element(queue=w470, element=w468, timeout in ms (-1)=w445) -> (queue out=w469:refnum<queue>, error out=w467:errorcluster)  [unwired: 1 in, 1 out]
            n168 = Lossy Enqueue Element(queue=w488, element=w486, error in (no error)=w463) -> (error out=w462:errorcluster)  [unwired: 3 out]
            n169 = flat-sequence {
              tunnel: w482 -> [w500]
              tunnel: [w499] -> w478
              tunnel: [w498] -> w477
              tunnel: [w497] -> w476
              tunnel: [w496] -> w475
              tunnel: w473 -> [w491]
              tunnel: w472 -> [w495]
              tunnel: 0.1 -> [w494]
              tunnel: w462 -> [_]
              tunnel: w461 -> [w493]
              frame #0 {
                w490 = "1" ("Channel")
                n170 = call-poly <instrlib>:"niScope Fetch (poly).vi"("timeout"=w494, "numSamples"=w500, "channels"="1" ("Channel"), "instrument handle"=w493) -> ("wfm"=w499:i8[][])  [unwired: 1 in, 6 out]
                n171 = call-poly <instrlib>:"niScope Fetch (poly).vi"("timeout"=w494, "numSamples"=w500, "instrument handle"=w491) -> ("wfm"=w498:i8[][])  [unwired: 2 in, 6 out]
                n172 = call-poly <instrlib>:"niScope Fetch (poly).vi"("timeout"=w494, "numSamples"=w500, "channels"=w490, "instrument handle"=w491) -> ("wfm"=w497:i8[][])  [unwired: 1 in, 6 out]
                n173 = call-poly <instrlib>:"niScope Fetch (poly).vi"("timeout"=w494, "numSamples"=w500, "channels"=w490, "instrument handle"=w495) -> ("wfm"=w496:i8[][])  [unwired: 1 in, 6 out]
              }
            }
            n174 = Enqueue Element(queue=w469, element=w478, timeout in ms (-1)=w445, error in (no error)=w467) -> (queue out=w481:refnum<queue>, error out=w466:errorcluster)  [unwired: 1 out]
            n175 = Wait on Notification(notifier=w459, timeout in ms (-1)=5) -> (timed out?=w458:bool)  [unwired: 2 in, 3 out]
            n176 = Enqueue Element(queue=w481, element=w477, timeout in ms (-1)=w445, error in (no error)=w466) -> (queue out=w480:refnum<queue>, error out=w465:errorcluster)  [unwired: 1 out]
            n177 = Not(x=w458) -> (.not. x?=w454:bool)
            n178 = Enqueue Element(queue=w480, element=w476, timeout in ms (-1)=w445, error in (no error)=w465) -> (queue out=w479:refnum<queue>, error out=w464:errorcluster)  [unwired: 1 out]
            n179 = Enqueue Element(queue=w479, element=w475, timeout in ms (-1)=w445, error in (no error)=w464) -> (error out=w452:errorcluster)  [unwired: 2 out]
            n180 = stacked-sequence {
              tunnel: w452 -> [_]
              tunnel: [w489] -> w450
              frame #0 {
                n181 = Tick Count (ms)() -> (millisecond timer value=w489:u32)
              }
            }
            n182 = Subtract(x=w450, y=w451) -> (x-y=w448:u32)
            n183 = call <vilib>:"Mean PtByPt.vi"("x"=w448, "sample length"=20) -> ("mean"=w447:dbl)  [unwired: 2 in, 1 out]
            n184 = local write "Read Loop"(w447) -> ()
          }
          n185 = And(x=w321, y=w352) -> (x .and. y?=w331:bool)
          n186 = Release Queue(queue=w351, force destroy? (F)=w331) -> ()  [unwired: 1 in, 3 out]
          n187 = Release Queue(queue=w334, force destroy? (F)=w331) -> ()  [unwired: 1 in, 3 out]
        }
        frame "1T/5R Deep Mem" {
          # "1T/5R test case/ This works but was a bit slower than case using flip flop gate. Also cam suffer memory overflow if Byte depth too small"
          # "Arm digitizer"
          n188 = Reverse 1D Array(array=w503) -> (reversed array=w513:void[])
          n189 = for {
            tunnel: [w580] -> w514
            tunnel: w513 -> [w579] mode=indexing
            n190 = call <instrlib>:"niScope Initiate Acquisition.vi"("instrument handle"=w579) -> ("error out"=w580:errorcluster)  [unwired: 2 in, 12 out]
          }
          n191 = Index Array(array=w503) -> (element=w502)  [unwired: 1 in]
          n192 = Index Array(array=w528) -> (element=w527:T17)  [unwired: 1 in]
          n193 = Obtain Queue(max queue size (-1, unlimited)=5, element data type=i8[][] [] ("Array")) -> (queue out=w522:refnum<queue>)  [unwired: 2 in, 3 out]
          n194 = Index Array(array=w528, index=1) -> (element=w523:T17)
          n195 = Index Array(array=w528, index=2) -> (element=w524:T17)
          n196 = Index Array(array=w528, index=3) -> (element=w525:T17)
          n197 = Index Array(array=w528, index=4) -> (element=w526:T17)
          n198 = Obtain Queue(max queue size (-1, unlimited)=2, element data type=cluster{"Fetch:Records Done":i32, bool} {"Fetch:Records Done"=0, TRUE}) -> (queue out=w520:refnum<queue>)  [unwired: 2 in, 3 out]
          n199 = node-c288() -> (w511:T13)  [unwired: 4 in]
          n200 = while {
            tunnel: w522 -> [w621]
            tunnel: [w603] -> w521
            tunnel: w526 -> [w585]
            tunnel: w525 -> [w588]
            tunnel: w527 -> [w596]
            tunnel: w523 -> [w594]
            tunnel: w524 -> [w592]
            shift-right: [w609] -> _
            shift-left: TRUE -> [w607]
            tunnel: w507 -> [w605]
            tunnel: w505 -> [w602]
            stop <- w603 stop-if-true
            w598 = 1000 ("timeout in ms (-1)")
            # "This loop does beam forming after data is read."
            n201 = Dequeue Element(queue=w621, timeout in ms (-1)=w598) -> (queue out=w616:refnum<queue>, element=w597:i8[][], error out=w617:errorcluster)  [unwired: 1 in, 1 out]
            n202 = call-poly "TimeShiftDataPoly.vi"("output cluster"=w596, "Array In"=w597) -> ("Array Out"=w583:i8[][])  [unwired: 1 in, 1 out]
            n203 = Dequeue Element(queue=w616, timeout in ms (-1)=w598, error in (no error)=w617) -> (queue out=w620:refnum<queue>, element=w595:i8[][], error out=w615:errorcluster)  [unwired: 1 out]
            n204 = call-poly "TimeShiftDataPoly.vi"("output cluster"=w594, "Array In"=w595) -> ("Array Out"=w591:i8[][])  [unwired: 1 in, 1 out]
            n205 = Dequeue Element(queue=w620, timeout in ms (-1)=w598, error in (no error)=w615) -> (queue out=w619:refnum<queue>, element=w593:i8[][], error out=w614:errorcluster)  [unwired: 1 out]
            n206 = To Word Integer(number=w591) -> (16bit integer=w582:i16[][])
            n207 = call-poly "TimeShiftDataPoly.vi"("output cluster"=w592, "Array In"=w593) -> ("Array Out"=w590:i8[][])  [unwired: 1 in, 1 out]
            n208 = Dequeue Element(queue=w619, timeout in ms (-1)=w598, error in (no error)=w614) -> (queue out=w618:refnum<queue>, element=w589:i8[][], error out=w613:errorcluster)  [unwired: 1 out]
            n209 = call-poly "TimeShiftDataPoly.vi"("output cluster"=w588, "Array In"=w589) -> ("Array Out"=w587:i8[][])  [unwired: 1 in, 1 out]
            n210 = Dequeue Element(queue=w618, timeout in ms (-1)=w598, error in (no error)=w613) -> (queue out=w612:refnum<queue>, element=w586:i8[][], error out=w611:errorcluster)  [unwired: 1 out]
            n211 = call-poly "TimeShiftDataPoly.vi"("output cluster"=w585, "Array In"=w586) -> ("Array Out"=w584:i8[][])  [unwired: 1 in, 1 out]
            n212 = Get Queue Status(queue=w612, error in (no error)=w611) -> (# elements in queue=→"SF queue":i32)  [unwired: 1 in, 7 out]
            n213 = Compound Arithmetic op=ADD(w582, w590, w587, w584) -> (w600:i16[][])
            n214 = expression code="x*2"(w600) -> ()  [unwired: 1 out]
            n215 = Wait on Notification(notifier=w602, timeout in ms (-1)=5) -> (timed out?=w601:bool)  [unwired: 2 in, 3 out]
            n216 = Compound Arithmetic op=ADD(w583, w600) -> (w599:i16[][])
            n217 = Not(x=w601) -> (.not. x?=w603:bool)
            n218 = Not(x=w607) -> (.not. x?=w609:bool)
            n219 = Bundle(0.0, w607, w599, 0) -> (w608:cluster{dbl, bool, i16[][], i32})  [unwired: 1 in]
            n220 = Lossy Enqueue Element(queue=w605, element=w608) -> ()  [unwired: 1 in, 4 out]
          }
          n221 = while {
            tunnel: w520 -> [w655]
            tunnel: [w633] -> w519
            tunnel: w522 -> [w653]
            tunnel: w534 -> [w636]
            tunnel: w533 -> [w652]
            tunnel: [w638] -> w517
            tunnel: [w644] -> w508
            tunnel: w505 -> [w634]
            tunnel: w504 -> [w631]
            tunnel: w503 -> [w629]
            tunnel: w501 -> [w622]
            stop <- w633 stop-if-true
            w630 = 483 items=["Start"=482, "Trigger"=483, "Pretrigger"=477, "Now"=481, "Read Pointer"=388] ("Fetch:Fetch Relative To")
            # "This loop reads the data once it is in the queue"
            # "Get and display data"
            n222 = Dequeue Element(queue=w655, timeout in ms (-1)=w631) -> (element=w654:cluster{"Fetch:Records Done":i32, bool}, error out=w646:errorcluster)  [unwired: 1 in, 2 out]
            n223 = Unbundle(w654) -> ("Fetch:Records Done"=w648:i32)  [unwired: 1 out]
            n224 = for {
              tunnel: w652 -> [w661]
              tunnel: w648 -> [w667]
              tunnel: [w666] -> w647
              tunnel: w646 -> [w665]
              tunnel: [w664] -> w626 mode=indexing
              tunnel: w630 -> [w663]
              tunnel: w629 -> [w662]
              n225 = property class="niScope"(reference=w662, error in=w665, "Fetch Relative To"=w663, "Fetch Record Number"=w667, "Fetch Number of Records"=w661) -> (reference out=w664:refnum<k15>, error out=w666:errorcluster)
            }
            n226 = Index Array(array=w626) -> (element=w623:refnum<k15>)  [unwired: 1 in]
            n227 = call-poly <instrlib>:"niScope Fetch (poly).vi"("timeout"=w622, "error in"=w647, "numSamples"=w636, "instrument handle"=w623) -> ("error out"=w645:errorcluster, "wfm"=w649:i8[][])  [unwired: 1 in, 5 out]
            n228 = Enqueue Element(queue=w653, element=w649, error in (no error)=w645) -> (queue out=w642:refnum<queue>, error out=w643:errorcluster)  [unwired: 1 in, 1 out]
            n229 = call-poly <instrlib>:"niScope Fetch (poly).vi"("timeout"=w622, "numSamples"=w636, "channels"="1", "instrument handle"=w623) -> ("wfm"=w639:i8[][])  [unwired: 1 in, 6 out]
            n230 = Index Array(array=w626, index=2) -> (element=w625:refnum<k15>)
            n231 = Index Array(array=w626, index=1) -> (element=w624:refnum<k15>)
            n232 = Enqueue Element(queue=w642, element=w639, error in (no error)=w643) -> (queue out=w640:refnum<queue>, error out=w641:errorcluster)  [unwired: 1 in, 1 out]
            n233 = stacked-sequence {
              tunnel: [w677] -> w658
              tunnel: [w676] -> w657
              tunnel: [w675] -> w656
              tunnel: w636 -> [w674]
              tunnel: w622 -> [w673]
              tunnel: w625 -> [w672]
              tunnel: w624 -> [w671]
              tunnel: [w668] -> w644
              frame #0 {
                n234 = call-poly <instrlib>:"niScope Fetch (poly).vi"("timeout"=w673, "numSamples"=w674, "instrument handle"=w671) -> ("wfm"=w677:i8[][])  [unwired: 2 in, 6 out]
                n235 = call-poly <instrlib>:"niScope Fetch (poly).vi"("timeout"=w673, "numSamples"=w674, "channels"="1" ("Channel"), "instrument handle"=w671) -> ("wfm"=w676:i8[][])  [unwired: 1 in, 6 out]
                n236 = call-poly <instrlib>:"niScope Fetch (poly).vi"("timeout"=w673, "numSamples"=w674, "channels"="1" ("Channel"), "instrument handle"=w672) -> ("error out"=w668:errorcluster, "wfm"=w675:i8[][])  [unwired: 1 in, 5 out]
              }
            }
            n237 = Enqueue Element(queue=w640, element=w658, error in (no error)=w641) -> (queue out=w660:refnum<queue>, error out=w651:errorcluster)  [unwired: 1 in, 1 out]
            n238 = Wait on Notification(notifier=w634, timeout in ms (-1)=5) -> (timed out?=w632:bool)  [unwired: 2 in, 3 out]
            n239 = Enqueue Element(queue=w660, element=w657, error in (no error)=w651) -> (queue out=w659:refnum<queue>, error out=w650:errorcluster)  [unwired: 1 in, 1 out]
            n240 = Not(x=w632) -> (.not. x?=w633:bool)
            n241 = Enqueue Element(queue=w659, element=w656, error in (no error)=w650) -> (queue out=w638:refnum<queue>)  [unwired: 1 in, 2 out]
          }
          n242 = timed-loop {
            shift-right: [w554] -> _
            shift-left: 0 -> [w561]
            shift-right: [w568] -> _
            shift-left: TRUE -> [w562]
            tunnel: w537 -> [w566]
            tunnel: w520 -> [w558]
            tunnel: [w548] -> w518
            tunnel: w502 -> [w560]
            tunnel: w515 -> [w555]
            tunnel: w514 -> [w564]
            timing: w511 -> [_]
            timing-out: [_] -> w510
            tunnel: [w544] -> w506
            tunnel: w505 -> [w543]
            stop <- w544 stop-if-true
            # "This loop performs back and forth scan and records record # at end of run"
            n243 = Bundle(w561, w562) -> (w559:cluster{i32, bool})  [unwired: 1 in]
            n244 = Select(t=T11 6 ("Program (1)"), s=w562, f=T11 7 ("Program (1)")) -> (s? t:f=w565:T11)
            n245 = call <vilib>:"Run Program.flx"("error in (no error)"=w564, "Program (1)"=w565, "Board ID"=w566) -> ("error out"=w557:errorcluster, "Bd ID Out"=w552:T5)  [unwired: 4 out]
            n246 = stacked-sequence {
              tunnel: w557 -> [w572]
              tunnel: [w572] -> w556
              tunnel: [w570] -> w553
              tunnel: w552 -> [w570]
              frame #0 {
                n247 = Wait (ms)(milliseconds to wait=35) -> ()  [unwired: 1 out]
              }
            }
            n248 = call-poly <vilib>:"Wait for Move Complete.flx"("Poll Interval (20 ms)"=5, "error in (no error)"=w556, "Axis or Vector Space"=w555, "Board ID"=w553) -> ("error out"=w563:errorcluster)  [unwired: 4 in, 3 out]
            n249 = property class="niScope"(reference=w560, error in=w563) -> (error out=w551:errorcluster, "Records Done"=w554:i32)  [unwired: 1 out]
            n250 = Wait on Notification(notifier=w543, timeout in ms (-1)=5) -> (timed out?=w542:bool)  [unwired: 2 in, 3 out]
            n251 = Lossy Enqueue Element(queue=w558, element=w559, error in (no error)=w551) -> (queue out=w549:refnum<queue>, error out=w547:errorcluster)  [unwired: 2 out]
            n252 = Not(x=w542) -> (.not. x?=w544:bool)
            n253 = Not(x=w562) -> (.not. x?=w568:bool)
            n254 = Get Queue Status(queue=w549, error in (no error)=w547) -> (queue out=w548:refnum<queue>, # elements in queue=→"Record queue":i32)  [unwired: 1 in, 6 out]
          }
          n255 = node-c288(w510) -> ()
          n256 = Compound Arithmetic op=AND(w506, w519, w521) -> (w512:bool)
          n257 = Release Queue(queue=w518, force destroy? (F)=w512) -> ()  [unwired: 1 in, 3 out]
          n258 = for {
            tunnel: w503 -> [w578]
            tunnel: w508 -> [w577]
            n259 = call <instrlib>:"niScope Abort.vi"("instrument handle"=w578, "error in"=w577) -> ()  [unwired: 12 in, 2 out]
          }
          n260 = Release Queue(queue=w517, force destroy? (F)=w512) -> ()  [unwired: 1 in, 3 out]
        }
        frame "Full 25 Ch" {
          w709 = 10
          w704 = 2 ("index")
          w720 = 5
          w711 = "0,1"
          # "Restructure file names"
          # "Read queue and send to files. About same as reading channel by channel"
          n261 = Reshape Array(w721, w720, w720) -> (w702:T19)
          n262 = Array To Cluster(array=w680) -> (cluster=w694:cluster{"[0]":void, "[1]":void, "[2]":void})
          n263 = Unbundle(w694) -> ("[1]"=w693, "[2]"=w692)  [unwired: 1 out]
          n264 = expression code="x*5"(w716) -> (w722:dbl)
          n265 = Index Array(array=w702, index (col)=4 ("index")) -> (element=w708:T20)  [unwired: 1 in]
          n266 = Array Subset(array=w702, index (col)=w704, length (col)=w704) -> (w707:T19)  [unwired: 2 in]
          n267 = Array Subset(array=w702, length (col)=2 ("index")) -> (w706:T19)  [unwired: 3 in]
          n268 = Obtain Queue(max queue size (-1, unlimited)=3, element data type=w682) -> (queue out=w690:refnum<queue>)  [unwired: 3 in, 2 out]
          n269 = call "RTHeader.vi"("Comment"="Full 25", "Votage scaling"=w679) -> ("Header String Out"=w698:string)  [unwired: 4 in, 1 out]
          n270 = Reshape Array(w706, w709) -> (w710:T20)
          n271 = Reshape Array(w707, w709) -> (w715:T20)
          n272 = Build Array(w711, w711, "1") -> (w724:string[])
          n273 = Build Array(w710, w715, w708) -> (w714:T19)
          n274 = while {
            tunnel: w690 -> [w758]
            tunnel: w701 -> [w757]
            tunnel: [w746] -> w717
            tunnel: w716 -> [w756]
            tunnel: w695 -> [w753]
            tunnel: w696 -> [w755]
            tunnel: w714 -> [w751]
            tunnel: i32[] [10, 10, 5] -> [w752]
            tunnel: w687 -> [w749]
            tunnel: [w743] -> w700
            tunnel: w698 -> [w748]
            tunnel: w697 -> [w744]
            tunnel: w684 -> [w731]
            tunnel: w683 -> [w730]
            tunnel: w678 -> [w725]
            i -> [w729]
            stop <- w746 stop-if-true
            n275 = for {
              tunnel: w757 -> [w785]
              tunnel: w756 -> [w793]
              tunnel: w758 -> [w795]
              tunnel: [w769] -> w726
              tunnel: [w784] -> w754
              tunnel: [w779] -> w750
              tunnel: w753 -> [w792]
              tunnel: w751 -> [_] mode=indexing
              tunnel: w752 -> [w788]
              tunnel: w751 -> [w790]
              tunnel: w749 -> [w787]
              tunnel: w748 -> [w782]
              tunnel: [w780] -> w741 mode=indexing
              tunnel: [w778] -> w739 mode=indexing
              tunnel: w731 -> [w773]
              tunnel: w730 -> [w772]
              tunnel: w729 -> [w771]
              tunnel: [w770] -> w728 mode=indexing
              tunnel: w725 -> [w768]
              n276 = Dequeue Element(queue=w795, timeout in ms (-1)=w787) -> (element=w776:T12, error out=w777:errorcluster)  [unwired: 1 in, 2 out]
              n277 = flat-sequence {
                tunnel: [w798] -> w780
                tunnel: w777 -> [_]
                tunnel: w776 -> [w797]
                tunnel: [w797] -> w775
                frame #0 {
                  n278 = Tick Count (ms)() -> (millisecond timer value=w798:u32)
                }
              }
              n279 = Unbundle(w775) -> ("gain"=w784:dbl, "wfm"=w783:i8[][], w769:bool, "max queue size (-1, unlimited)"=w781:i32)
              n280 = Index Array(array=w788, index=w781) -> (element=w786:i32)
              n281 = Index Array(array=w790, index (row)=w781) -> (element=w789:T20)  [unwired: 1 in]
              n282 = Multiply(x=w785, y=w786) -> (x*y=w791:i32)
              n283 = Reshape Array(w783, w793, w791) -> (w794:i8[][])
              n284 = Get Notifier Status(notifier=w773) -> (current notification=w774:bool)  [unwired: 1 in, 4 out]
              n285 = for {
                N: w786 -> [_]
                tunnel: w789 -> [w819]
                tunnel: [w822] -> w779
                tunnel: w792 -> [w821]
                shift-right: [w814] -> _
                shift-left: w794 -> [w823]
                tunnel: w785 -> [w817]
                tunnel: [w812] -> w770 mode=indexing
                tunnel: w768 -> [w811]
                i -> [w820]
                n286 = Index Array(array=w819, index=w820) -> (element=w815:T17)
                n287 = Delete From Array(array=w823, length=w817, index (col)=0 ("disabled index (col)")) -> (deleted portion=w816:i8[], array with subset deleted=w814:i8[][])  [unwired: 1 in]
                n288 = call "TimeShiftDataSubMean.vi"("Filter"=w811, "output cluster"=w815, "Array In"=w816) -> ("Array Out"=w813:i16[][], "Sat Pts"=w812:i32)  [unwired: 2 in]
                n289 = in-place {
                  in-place-border: w813 -> [w826]
                  n290 = in-place-dvr #1(w821) -> (w824:i16[][])  [unwired: 1 out]
                  n291 = Add(x=w826, y=w824) -> (x+y=w825:i16[][])
                  n292 = in-place-dvr #1(w825) -> (w822:refnum<data-value>)  [unwired: 1 out]
                }
              }
              n293 = case shown="True" w774 {
                tunnel: w781 -> [_ w804]
                tunnel: w783 -> [_ w801]
                tunnel: w782 -> [_ w805]
                tunnel: w772 -> [_ w803]
                tunnel: w771 -> [_ w802]
                tunnel: w769 -> [_ w799]
                frame False {
                }
                frame True {
                  n294 = case shown="True" w799 {
                    tunnel: w801 -> [w806 w810]
                    tunnel: [w806 w809] -> w800
                    frame False {
                    }
                    frame True {
                      w808 = 0 ("index (row)")
                      n295 = Replace Array Subset(array=w810, new element=127 ("index (row)"), index (row)=w808, index (col)=w808) -> (w809:i8[][])
                    }
                  }
                  n296 = call "RawRT_Capture.vi"("Raw data"=w800, "File Name In"=w803, "DigCard"=w804, "header"=w805, "Iter"=w802) -> ()  [unwired: 7 in]
                }
              }
              n297 = flat-sequence {
                tunnel: [w796] -> w778
                tunnel: w779 -> [_]
                frame #0 {
                  n298 = Tick Count (ms)() -> (millisecond timer value=w796:u32)
                }
              }
            }
            n299 = Wait on Notification(notifier=w744, timeout in ms (-1)=5) -> (timed out?=w747:bool)  [unwired: 2 in, 3 out]
            n300 = Add Array Elements(numeric array=w728) -> (sum=w727:i32)
            n301 = in-place {
              in-place-border: w755 -> [w767]
              in-place-border: w726 -> [w766]
              in-place-border: w754 -> [w765]
              in-place-border: w727 -> [w760]
              n302 = in-place-dvr #2(w750) -> (w761:i16[][])  [unwired: 1 out]
              n303 = Bundle("gain"=w765, w766, w761, "Sat Pts"=w760) -> (w764:T21)  [unwired: 1 in]
              n304 = Multiply(x=i16 0, y=w761) -> (x*y=w763:i16[][])
              n305 = Lossy Enqueue Element(queue=w767, element=w764) -> ()  [unwired: 1 in, 4 out]
              n306 = in-place-dvr #2(w763) -> (w743:refnum<data-value>)  [unwired: 1 out]
            }
            n307 = Subtract(x=w739, y=w741) -> (x-y=w740:u32[])
            n308 = Not(x=w747) -> (.not. x?=w746:bool)
            n309 = Index Array(array=w739, index=2) -> (element=w737:u32)
            n310 = Add Array Elements(numeric array=w740) -> (sum=w736:u32)
            n311 = Subtract(x=w742, y=w737) -> (x-y=w735:u32)
            n312 = Add(x=w735, y=w736) -> (x+y=w734:u32)
            n313 = flat-sequence {
              tunnel: [w759] -> w742
              tunnel: w743 -> [_]
              frame #0 {
                n314 = Tick Count (ms)() -> (millisecond timer value=w759:u32)
              }
            }
            n315 = call <vilib>:"Mean PtByPt.vi"("x"=w734, "sample length"=20) -> ("mean"=w732:dbl)  [unwired: 2 in, 1 out]
            n316 = local write "SF Loop"(w732) -> ()
          }
          n317 = while {
            tunnel: w724 -> [w849]
            tunnel: w690 -> [w848]
            tunnel: w693 -> [w847]
            tunnel: w692 -> [w846]
            tunnel: w722 -> [w845]
            tunnel: w701 -> [w844]
            tunnel: [w843] -> w718
            tunnel: w691 -> [w836]
            shift-right: [w832] -> _
            shift-left: _ -> [w842]
            tunnel: [w830] -> _
            tunnel: w697 -> [w838]
            tunnel: w680 -> [w837]
            tunnel: w686 -> [w835]
            tunnel: w685 -> [w829]
            shift-right: [w827] -> _
            shift-left: errorcluster {"status"=FALSE, "code"=0, "source"=""} ("error out") -> [w828]
            stop <- w839 stop-if-true
            n318 = for {
              tunnel: w844 -> [w869]
              tunnel: w845 -> [w871]
              tunnel: w849 -> [w870] mode=indexing
              tunnel: w848 -> [w861]
              tunnel: w847 -> [w866]
              tunnel: w846 -> [w865]
              tunnel: [w864] -> w843
              tunnel: w836 -> [w862]
              tunnel: w837 -> [w863]
              tunnel: w835 -> [w860]
              tunnel: [w852] -> w834
              tunnel: w829 -> [w857]
              shift-right: [w855] -> _
              shift-left: _ -> [w854]
              shift-right: [w852] -> w827
              shift-left: w828 -> [w851]
              i -> [w859]
              # "Read data"
              n319 = case shown="0" w859 {
                tunnel: w871 -> [_ w898]
                tunnel: w863 -> [w879 w897]
                tunnel: w870 -> [w877 w895]
                tunnel: w869 -> [w880 w894]
                tunnel: [w881 w893] -> w868
                tunnel: [w882 w892] -> w867
                tunnel: w866 -> [w886 _]
                tunnel: w865 -> [w885 _]
                tunnel: [w878 w889] -> w855
                tunnel: w862 -> [w876 _]
                tunnel: w860 -> [w875 _]
                tunnel: w857 -> [w874 w890]
                tunnel: w854 -> [_ w889]
                tunnel: [w873 w888] -> w853
                tunnel: w851 -> [w872 w887]
                frame 0 {
                  # "Read files and queue it up."
                  n320 = call <instrlib>:"niScope Initiate Acquisition.vi"("instrument handle"=w886, "error in"=w872) -> ("error out"=w884:errorcluster)  [unwired: 1 in, 12 out]
                  n321 = call <instrlib>:"niScope Initiate Acquisition.vi"("instrument handle"=w885, "error in"=w884) -> ("error out"=w883:errorcluster)  [unwired: 1 in, 12 out]
                  n322 = call "Rapid Read_NI.vi"("NI Card"=w879, "Channel"=w877, "Motion Board ID"=w876, "rf points per line"=w880, "error in"=w883, "timeout"=w874, "Pause?"=w875) -> ("dig gain"=w881:dbl, "Array"=w882:i8[][], "Reverse?"=w878:bool, "error out"=w873:errorcluster)  [unwired: 5 in]
                }
                frame 1, Default {
                  n323 = property class="niScope"(reference=w897, error in=w887, "Fetch Record Number"=0, "Fetch Number of Records"=w898) -> (reference out=w896:refnum<k15>, error out=w891:errorcluster)
                  n324 = call-poly <instrlib>:"niScope Fetch (poly).vi"("timeout"=w890, "error in"=w891, "numSamples"=w894, "channels"=w895, "instrument handle"=w896) -> ("error out"=w888:errorcluster, "wfm"=w892:i8[][], "wfm info"=w901:T22)  [unwired: 4 out]
                  n325 = Index Array(array=w901) -> (element=w900:T23)  [unwired: 1 in]
                  n326 = Unbundle By Name(w900) -> ("gain"=w893:dbl)
                }
              }
              n327 = Bundle("gain"=w868, "wfm"=w867, "Reverse?"=w855, w859) -> (w858:T24)  [unwired: 1 in]
              n328 = Enqueue Element(queue=w861, element=w858, timeout in ms (-1)=1000, error in (no error)=w853) -> (queue out=w864:refnum<queue>, error out=w852:errorcluster)  [unwired: 1 out]
            }
            n329 = Wait on Notification(notifier=w838, timeout in ms (-1)=5) -> (timed out?=w841:bool)  [unwired: 2 in, 3 out]
            n330 = flat-sequence {
              tunnel: [w850] -> w832
              tunnel: w834 -> [_]
              frame #0 {
                n331 = Tick Count (ms)() -> (millisecond timer value=w850:u32)
              }
            }
            n332 = Not(x=w841) -> (.not. x?=w839:bool)
            n333 = Subtract(x=w832, y=w842) -> (x-y=w830:u32)
            n334 = call <vilib>:"Mean PtByPt.vi"("x"=w830, "sample length"=20) -> ("mean"=w831:dbl)  [unwired: 2 in, 1 out]
            n335 = local write "Read Loop"(w831) -> ()
          }
          n336 = Release Queue(queue=w718, force destroy? (F)=w717) -> (error out=w688:errorcluster)  [unwired: 1 in, 2 out]
          n337 = Delete Data Value Reference(data value reference=w700) -> (error out=w689:errorcluster)  [unwired: 1 in, 1 out]
        }
        frame "Drop Ch 5 XMIT" {
          w905 = 4 ("index")
          w935 = 8
          w931 = 2 ("index")
          w946 = 5
          w937 = "0,1"
          # "Restructure file names"
          # "Read queue and send to files. About same as reading channel by channel"
          n338 = Reshape Array(w947, w946, w946) -> (w930:T19)
          n339 = Array To Cluster(array=w919) -> (cluster=w922:cluster{"[0]":void, "[1]":void, "[2]":void})
          n340 = Unbundle(w922) -> ("[1]"=w921, "[2]"=w920)  [unwired: 1 out]
          n341 = expression code="x*4"(w942) -> (w948:dbl)
          n342 = Index Array(array=w930, index (col)=4 ("index")) -> (element=w909:T20)  [unwired: 1 in]
          n343 = Array Subset(array=w930, length (row)=w905, index (col)=w931, length (col)=w931) -> (w934:T19)  [unwired: 1 in]
          n344 = Array Subset(array=w930, length (row)=w905, length (col)=2 ("index")) -> (w933:T19)  [unwired: 2 in]
          n345 = call "RTHeader.vi"("Comment"="Drop 5 Xmit", "Votage scaling"=w903) -> ("Header String Out"=w926:string)  [unwired: 4 in, 1 out]
          n346 = Obtain Queue(max queue size (-1, unlimited)=3, element data type=w904) -> (queue out=w917:refnum<queue>)  [unwired: 3 in, 2 out]
          n347 = Array Subset(array=w909, length=w905) -> (w908:T20)  [unwired: 1 in]
          n348 = Reshape Array(w933, w935) -> (w936:T20)
          n349 = Reshape Array(w934, w935) -> (w941:T20)
          n350 = Build Array(w937, w937, "1") -> (w950:string[])
          n351 = Build Array(w936, w941, w908) -> (w940:T19)
          n352 = while {
            tunnel: w917 -> [w985]
            tunnel: w929 -> [w984]
            tunnel: [w973] -> w943
            tunnel: w942 -> [w983]
            tunnel: w923 -> [w980]
            tunnel: w924 -> [w982]
            tunnel: w940 -> [w978]
            tunnel: i32[] [8, 8, 4] -> [w979]
            tunnel: w914 -> [w976]
            tunnel: [w970] -> w928
            tunnel: w926 -> [w975]
            tunnel: w925 -> [w971]
            tunnel: w911 -> [w958]
            tunnel: w910 -> [w957]
            tunnel: i16[] [1, 1, 2] -> [w953]
            tunnel: w902 -> [w951]
            i -> [w956]
            stop <- w973 stop-if-true
            n353 = for {
              tunnel: w984 -> [w1013]
              tunnel: w983 -> [w1022]
              tunnel: w985 -> [w1024]
              tunnel: [w1021] -> w952
              tunnel: [w1012] -> w981
              tunnel: [w1008] -> w977
              tunnel: w980 -> [w1020]
              tunnel: w978 -> [_] mode=indexing
              tunnel: w979 -> [w1016]
              tunnel: w978 -> [w1018]
              tunnel: w976 -> [w1015]
              tunnel: w975 -> [w1010]
              tunnel: [w1009] -> w968 mode=indexing
              tunnel: [w1007] -> w966 mode=indexing
              tunnel: w958 -> [w1002]
              tunnel: w957 -> [w1001]
              tunnel: w956 -> [w1000]
              tunnel: [w999] -> w955 mode=indexing
              tunnel: w953 -> [w997]
              tunnel: w951 -> [w995]
              n354 = Dequeue Element(queue=w1024, timeout in ms (-1)=w1015) -> (element=w1005:T12, error out=w1006:errorcluster)  [unwired: 1 in, 2 out]
              n355 = flat-sequence {
                tunnel: [w1027] -> w1009
                tunnel: w1006 -> [_]
                tunnel: w1005 -> [w1026]
                tunnel: [w1026] -> w1004
                frame #0 {
                  n356 = Tick Count (ms)() -> (millisecond timer value=w1027:u32)
                }
              }
              n357 = Unbundle(w1004) -> ("gain"=w1012:dbl, "wfm"=w1011:i8[][], w1021:bool, "max queue size (-1, unlimited)"=w998:i32)
              n358 = Index Array(array=w1016, index=w998) -> (element=w1014:i32)
              n359 = Index Array(array=w997, index=w998) -> (element=w996:i16)
              n360 = Index Array(array=w1018, index (row)=w998) -> (element=w1017:T20)  [unwired: 1 in]
              n361 = Multiply(x=w1013, y=w1014) -> (x*y=w1019:i32)
              n362 = Reshape Array(w1011, w1022, w1019) -> (w1023:i8[][])
              n363 = Get Notifier Status(notifier=w1002) -> (current notification=w1003:bool)  [unwired: 1 in, 4 out]
              n364 = for {
                N: w1014 -> [_]
                tunnel: w1017 -> [w1042]
                tunnel: [w1045] -> w1008
                tunnel: w1020 -> [w1044]
                shift-right: [w1037] -> _
                shift-left: w1023 -> [w1046]
                tunnel: w1013 -> [w1040]
                tunnel: [w1035] -> w999 mode=indexing
                tunnel: w996 -> [w1034]
                tunnel: w995 -> [w1033]
                i -> [w1043]
                n365 = Index Array(array=w1042, index=w1043) -> (element=w1038:T17)
                n366 = Delete From Array(array=w1046, length=w1040, index (col)=0 ("disabled index (col)")) -> (deleted portion=w1039:i8[], array with subset deleted=w1037:i8[][])  [unwired: 1 in]
                n367 = call "TimeShiftDataSubMean.vi"("Filter"=w1033, "output cluster"=w1038, "Array In"=w1039) -> ("Array Out"=w1036:i16[][], "Sat Pts"=w1035:i32)  [unwired: 2 in]
                n368 = in-place {
                  in-place-border: w1036 -> [w1049]
                  in-place-border: w1034 -> [w1047]
                  n369 = in-place-dvr #3(w1044) -> (w1050:i16[][])  [unwired: 1 out]
                  n370 = case shown="2" w1047 {
                    selector: w1047 -> [_ w1053]
                    tunnel: w1049 -> [w1052 w1055]
                    tunnel: [w1052 w1054] -> w1048
                    frame 0, Default {
                    }
                    frame 2 {
                      n371 = Multiply(x=w1053, y=w1055) -> (x*y=w1054:i16[][])
                    }
                  }
                  n372 = Add(x=w1048, y=w1050) -> (x+y=w1051:i16[][])
                  n373 = in-place-dvr #3(w1051) -> (w1045:refnum<data-value>)  [unwired: 1 out]
                }
              }
              n374 = case shown="True" w1003 {
                tunnel: w998 -> [_ w1031]
                tunnel: w1011 -> [_ w1030]
                tunnel: w1010 -> [_ w1032]
                tunnel: w1001 -> [_ w1029]
                tunnel: w1000 -> [_ w1028]
                frame False {
                }
                frame True {
                  n375 = call "RawRT_Capture.vi"("Raw data"=w1030, "File Name In"=w1029, "DigCard"=w1031, "header"=w1032, "Iter"=w1028) -> ()  [unwired: 7 in]
                }
              }
              n376 = flat-sequence {
                tunnel: [w1025] -> w1007
                tunnel: w1008 -> [_]
                frame #0 {
                  n377 = Tick Count (ms)() -> (millisecond timer value=w1025:u32)
                }
              }
            }
            n378 = Wait on Notification(notifier=w971, timeout in ms (-1)=5) -> (timed out?=w974:bool)  [unwired: 2 in, 3 out]
            n379 = Add Array Elements(numeric array=w955) -> (sum=w954:i32)
            n380 = in-place {
              in-place-border: w982 -> [w994]
              in-place-border: w952 -> [w993]
              in-place-border: w981 -> [w992]
              in-place-border: w954 -> [w987]
              n381 = in-place-dvr #4(w977) -> (w988:i16[][])  [unwired: 1 out]
              n382 = Bundle("gain"=w992, w993, w988, "Sat Pts"=w987) -> (w991:T21)  [unwired: 1 in]
              n383 = Multiply(x=i16 0, y=w988) -> (x*y=w990:i16[][])
              n384 = Lossy Enqueue Element(queue=w994, element=w991) -> ()  [unwired: 1 in, 4 out]
              n385 = in-place-dvr #4(w990) -> (w970:refnum<data-value>)  [unwired: 1 out]
            }
            n386 = Subtract(x=w966, y=w968) -> (x-y=w967:u32[])
            n387 = Not(x=w974) -> (.not. x?=w973:bool)
            n388 = Index Array(array=w966, index=2) -> (element=w964:u32)
            n389 = Add Array Elements(numeric array=w967) -> (sum=w963:u32)
            n390 = Subtract(x=w969, y=w964) -> (x-y=w962:u32)
            n391 = Add(x=w962, y=w963) -> (x+y=w961:u32)
            n392 = flat-sequence {
              tunnel: [w986] -> w969
              tunnel: w970 -> [_]
              frame #0 {
                n393 = Tick Count (ms)() -> (millisecond timer value=w986:u32)
              }
            }
            n394 = call <vilib>:"Mean PtByPt.vi"("x"=w961, "sample length"=20) -> ("mean"=w959:dbl)  [unwired: 2 in, 1 out]
            n395 = local write "SF Loop"(w959) -> ()
          }
          n396 = while {
            tunnel: w950 -> [w1076]
            tunnel: w917 -> [w1075]
            tunnel: w921 -> [w1074]
            tunnel: w920 -> [w1073]
            tunnel: w948 -> [w1072]
            tunnel: w929 -> [w1071]
            tunnel: [w1070] -> w944
            tunnel: w918 -> [w1063]
            shift-right: [w1059] -> _
            shift-left: _ -> [w1069]
            tunnel: [w1057] -> _
            tunnel: w925 -> [w1065]
            tunnel: w919 -> [w1064]
            tunnel: w913 -> [w1062]
            tunnel: w912 -> [w1056]
            stop <- w1066 stop-if-true
            n397 = for {
              tunnel: w1071 -> [w1094]
              tunnel: w1072 -> [w1096]
              tunnel: w1076 -> [w1095] mode=indexing
              tunnel: w1075 -> [w1086]
              tunnel: w1074 -> [w1091]
              tunnel: w1073 -> [w1090]
              tunnel: [w1089] -> w1070
              tunnel: w1063 -> [w1087]
              tunnel: w1064 -> [w1088]
              tunnel: w1062 -> [w1085]
              tunnel: [w1082] -> w1061
              tunnel: w1056 -> [w1081]
              shift-right: [w1079] -> _
              shift-left: _ -> [w1078]
              i -> [w1084]
              # "Read data"
              n398 = case shown="0" w1084 {
                tunnel: w1096 -> [_ w1119]
                tunnel: w1088 -> [w1102 w1118]
                tunnel: w1095 -> [w1100 w1116]
                tunnel: w1094 -> [w1103 w1115]
                tunnel: [w1104 w1114] -> w1093
                tunnel: [w1105 w1113] -> w1092
                tunnel: w1091 -> [w1109 _]
                tunnel: w1090 -> [w1108 _]
                tunnel: [w1101 w1110] -> w1079
                tunnel: w1087 -> [w1099 _]
                tunnel: w1085 -> [w1098 _]
                tunnel: w1081 -> [w1097 w1111]
                tunnel: w1078 -> [_ w1110]
                frame 0 {
                  # "Read files and queue it up."
                  n399 = call <instrlib>:"niScope Initiate Acquisition.vi"("instrument handle"=w1109) -> ("error out"=w1107:errorcluster)  [unwired: 2 in, 12 out]
                  n400 = call <instrlib>:"niScope Initiate Acquisition.vi"("instrument handle"=w1108, "error in"=w1107) -> ("error out"=w1106:errorcluster)  [unwired: 1 in, 12 out]
                  n401 = call "Rapid Read_NI.vi"("NI Card"=w1102, "Channel"=w1100, "Motion Board ID"=w1099, "rf points per line"=w1103, "error in"=w1106, "timeout"=w1097, "Pause?"=w1098) -> ("dig gain"=w1104:dbl, "Array"=w1105:i8[][], "Reverse?"=w1101:bool)  [unwired: 5 in, 1 out]
                }
                frame 1, Default {
                  n402 = property class="niScope"(reference=w1118, "Fetch Record Number"=0, "Fetch Number of Records"=w1119) -> (reference out=w1117:refnum<k15>, error out=w1112:errorcluster)  [unwired: 1 in]
                  n403 = call-poly <instrlib>:"niScope Fetch (poly).vi"("timeout"=w1111, "error in"=w1112, "numSamples"=w1115, "channels"=w1116, "instrument handle"=w1117) -> ("wfm"=w1113:i8[][], "wfm info"=w1122:T22)  [unwired: 5 out]
                  n404 = Index Array(array=w1122) -> (element=w1121:T23)  [unwired: 1 in]
                  n405 = Unbundle By Name(w1121) -> ("gain"=w1114:dbl)
                }
              }
              n406 = Bundle("gain"=w1093, "wfm"=w1092, "Reverse?"=w1079, w1084) -> (w1083:T24)  [unwired: 1 in]
              n407 = Enqueue Element(queue=w1086, element=w1083, timeout in ms (-1)=100) -> (queue out=w1089:refnum<queue>, error out=w1082:errorcluster)  [unwired: 1 in, 1 out]
            }
            n408 = Wait on Notification(notifier=w1065, timeout in ms (-1)=5) -> (timed out?=w1068:bool)  [unwired: 2 in, 3 out]
            n409 = flat-sequence {
              tunnel: [w1077] -> w1059
              tunnel: w1061 -> [_]
              frame #0 {
                n410 = Tick Count (ms)() -> (millisecond timer value=w1077:u32)
              }
            }
            n411 = Not(x=w1068) -> (.not. x?=w1066:bool)
            n412 = Subtract(x=w1059, y=w1069) -> (x-y=w1057:u32)
            n413 = call <vilib>:"Mean PtByPt.vi"("x"=w1057, "sample length"=20) -> ("mean"=w1058:dbl)  [unwired: 2 in, 1 out]
            n414 = local write "Read Loop"(w1058) -> ()
          }
          n415 = Release Queue(queue=w944, force destroy? (F)=w943) -> (error out=w915:errorcluster)  [unwired: 1 in, 2 out]
          n416 = Delete Data Value Reference(data value reference=w928) -> (error out=w916:errorcluster)  [unwired: 1 in, 1 out]
        }
        frame "Drop Ch 5,4 XMIT" {
          w1127 = 3 ("index")
          w1156 = 6
          w1152 = 2 ("index")
          w1167 = 5
          w1158 = "0,1"
          # "Restructure file names"
          # "Read queue and send to files. About same as reading channel by channel"
          n417 = Reshape Array(w1168, w1167, w1167) -> (w1151:T19)
          n418 = Array To Cluster(array=w1140) -> (cluster=w1143:cluster{"[0]":void, "[1]":void, "[2]":void})
          n419 = Unbundle(w1143) -> ("[1]"=w1142, "[2]"=w1141)  [unwired: 1 out]
          n420 = expression code="x*3"(w1163) -> (w1169:dbl)
          n421 = Index Array(array=w1151, index (col)=4 ("index")) -> (element=w1130:T20)  [unwired: 1 in]
          n422 = Array Subset(array=w1151, length (row)=w1127, index (col)=w1152, length (col)=w1152) -> (w1155:T19)  [unwired: 1 in]
          n423 = Array Subset(array=w1151, length (row)=w1127, length (col)=2 ("index")) -> (w1154:T19)  [unwired: 2 in]
          n424 = call "RTHeader.vi"("Comment"="Drop 5,4 Xmit", "Votage scaling"=w1124) -> ("Header String Out"=w1147:string)  [unwired: 4 in, 1 out]
          n425 = Obtain Queue(max queue size (-1, unlimited)=3, element data type=w1125) -> (queue out=w1138:refnum<queue>)  [unwired: 3 in, 2 out]
          n426 = Array Subset(array=w1130, length=w1127) -> (w1129:T20)  [unwired: 1 in]
          n427 = Reshape Array(w1154, w1156) -> (w1157:T20)
          n428 = Reshape Array(w1155, w1156) -> (w1162:T20)
          n429 = Build Array(w1158, w1158, "1") -> (w1171:string[])
          n430 = Build Array(w1157, w1162, w1129) -> (w1161:T19)
          n431 = while {
            tunnel: w1138 -> [w1207]
            tunnel: w1150 -> [w1206]
            tunnel: [w1193] -> w1164
            tunnel: w1163 -> [w1205]
            tunnel: w1144 -> [w1202]
            tunnel: w1145 -> [w1204]
            tunnel: w1161 -> [w1200]
            tunnel: i32[] [6, 6, 3] -> [w1201]
            tunnel: w1135 -> [w1196]
            tunnel: [w1190] -> w1149
            tunnel: w1147 -> [w1195]
            tunnel: w1146 -> [w1191]
            tunnel: w1132 -> [w1178]
            tunnel: w1131 -> [w1177]
            tunnel: i16[][] [[1, 1, 1, 1, 1, 1], [1, 2, 1, 2, 1, 2], [2, 2, 2, 0, 0, 0]] -> [w1173]
            tunnel: w1123 -> [w1172]
            i -> [w1176]
            stop <- w1193 stop-if-true
            n432 = for {
              tunnel: w1206 -> [w1235]
              tunnel: w1205 -> [w1244]
              tunnel: w1207 -> [w1246]
              tunnel: [w1243] -> w1199 mode=indexing
              tunnel: [w1234] -> w1203
              tunnel: [w1230] -> w1197
              tunnel: w1202 -> [w1242]
              tunnel: w1200 -> [_] mode=indexing
              tunnel: w1201 -> [w1238]
              tunnel: w1200 -> [w1240]
              tunnel: w1196 -> [w1237]
              tunnel: w1195 -> [w1232]
              tunnel: [w1231] -> w1188 mode=indexing
              tunnel: [w1229] -> w1186 mode=indexing
              tunnel: w1178 -> [w1224]
              tunnel: w1177 -> [w1223]
              tunnel: w1176 -> [w1222]
              tunnel: [w1221] -> w1175 mode=indexing
              tunnel: w1173 -> [w1219]
              tunnel: w1172 -> [w1217]
              n433 = Dequeue Element(queue=w1246, timeout in ms (-1)=w1237) -> (element=w1227:T12, error out=w1228:errorcluster)  [unwired: 1 in, 2 out]
              n434 = flat-sequence {
                tunnel: [w1249] -> w1231
                tunnel: w1228 -> [_]
                tunnel: w1227 -> [w1248]
                tunnel: [w1248] -> w1226
                frame #0 {
                  n435 = Tick Count (ms)() -> (millisecond timer value=w1249:u32)
                }
              }
              n436 = Unbundle(w1226) -> ("gain"=w1234:dbl, "wfm"=w1233:i8[][], w1243:bool, "max queue size (-1, unlimited)"=w1220:i32)
              n437 = Index Array(array=w1238, index=w1220) -> (element=w1236:i32)
              n438 = Index Array(array=w1219, index (row)=w1220) -> (element=w1218:i16[])  [unwired: 1 in]
              n439 = Index Array(array=w1240, index (row)=w1220) -> (element=w1239:T20)  [unwired: 1 in]
              n440 = Multiply(x=w1235, y=w1236) -> (x*y=w1241:i32)
              n441 = Reshape Array(w1233, w1244, w1241) -> (w1245:i8[][])
              n442 = Get Notifier Status(notifier=w1224) -> (current notification=w1225:bool)  [unwired: 1 in, 4 out]
              n443 = for {
                N: w1236 -> [_]
                tunnel: w1239 -> [w1264]
                tunnel: [w1267] -> w1230
                tunnel: w1242 -> [w1266]
                shift-right: [w1259] -> _
                shift-left: w1245 -> [w1268]
                tunnel: w1235 -> [w1262]
                tunnel: [w1257] -> w1221 mode=indexing
                tunnel: w1218 -> [w1256] mode=indexing
                tunnel: w1217 -> [w1255]
                i -> [w1265]
                n444 = Index Array(array=w1264, index=w1265) -> (element=w1260:T17)
                n445 = Delete From Array(array=w1268, length=w1262, index (col)=0 ("disabled index (col)")) -> (deleted portion=w1261:i8[], array with subset deleted=w1259:i8[][])  [unwired: 1 in]
                n446 = call "TimeShiftDataSubMean.vi"("Filter"=w1255, "output cluster"=w1260, "Array In"=w1261) -> ("Array Out"=w1258:i16[][], "Sat Pts"=w1257:i32)  [unwired: 2 in]
                n447 = in-place {
                  in-place-border: w1258 -> [w1271]
                  in-place-border: w1256 -> [w1269]
                  n448 = in-place-dvr #5(w1266) -> (w1272:i16[][])  [unwired: 1 out]
                  n449 = case shown="2" w1269 {
                    selector: w1269 -> [_ w1275]
                    tunnel: w1271 -> [w1274 w1277]
                    tunnel: [w1274 w1276] -> w1270
                    frame 0, Default {
                    }
                    frame 2 {
                      n450 = Multiply(x=w1275, y=w1277) -> (x*y=w1276:i16[][])
                    }
                  }
                  n451 = Add(x=w1270, y=w1272) -> (x+y=w1273:i16[][])
                  n452 = in-place-dvr #5(w1273) -> (w1267:refnum<data-value>)  [unwired: 1 out]
                }
              }
              n453 = case shown="True" w1225 {
                tunnel: w1220 -> [_ w1253]
                tunnel: w1233 -> [_ w1252]
                tunnel: w1232 -> [_ w1254]
                tunnel: w1223 -> [_ w1251]
                tunnel: w1222 -> [_ w1250]
                frame False {
                }
                frame True {
                  n454 = call "RawRT_Capture.vi"("Raw data"=w1252, "File Name In"=w1251, "DigCard"=w1253, "header"=w1254, "Iter"=w1250) -> ()  [unwired: 7 in]
                }
              }
              n455 = flat-sequence {
                tunnel: [w1247] -> w1229
                tunnel: w1230 -> [_]
                frame #0 {
                  n456 = Tick Count (ms)() -> (millisecond timer value=w1247:u32)
                }
              }
            }
            n457 = Wait on Notification(notifier=w1191, timeout in ms (-1)=5) -> (timed out?=w1194:bool)  [unwired: 2 in, 3 out]
            n458 = Add Array Elements(numeric array=w1175) -> (sum=w1174:i32)
            n459 = Subtract(x=w1186, y=w1188) -> (x-y=w1187:u32[])
            n460 = Not(x=w1194) -> (.not. x?=w1193:bool)
            n461 = Or Array Elements(Boolean array=w1199) -> (logical OR=w1198:bool)
            n462 = in-place {
              in-place-border: w1204 -> [w1216]
              in-place-border: w1198 -> [w1215]
              in-place-border: w1203 -> [w1214]
              in-place-border: w1174 -> [w1209]
              n463 = in-place-dvr #6(w1197) -> (w1210:i16[][])  [unwired: 1 out]
              n464 = Bundle("gain"=w1214, w1215, w1210, "Sat Pts"=w1209) -> (w1213:T21)  [unwired: 1 in]
              n465 = Multiply(x=i16 0, y=w1210) -> (x*y=w1212:i16[][])
              n466 = Lossy Enqueue Element(queue=w1216, element=w1213) -> ()  [unwired: 1 in, 4 out]
              n467 = in-place-dvr #6(w1212) -> (w1190:refnum<data-value>)  [unwired: 1 out]
            }
            n468 = Index Array(array=w1186, index=2) -> (element=w1184:u32)
            n469 = Add Array Elements(numeric array=w1187) -> (sum=w1183:u32)
            n470 = Subtract(x=w1189, y=w1184) -> (x-y=w1182:u32)
            n471 = Add(x=w1182, y=w1183) -> (x+y=w1181:u32)
            n472 = flat-sequence {
              tunnel: [w1208] -> w1189
              tunnel: w1190 -> [_]
              frame #0 {
                n473 = Tick Count (ms)() -> (millisecond timer value=w1208:u32)
              }
            }
            n474 = call <vilib>:"Mean PtByPt.vi"("x"=w1181, "sample length"=20) -> ("mean"=w1179:dbl)  [unwired: 2 in, 1 out]
            n475 = local write "SF Loop"(w1179) -> ()
          }
          n476 = while {
            tunnel: w1171 -> [w1298]
            tunnel: w1138 -> [w1297]
            tunnel: w1142 -> [w1296]
            tunnel: w1141 -> [w1295]
            tunnel: w1169 -> [w1294]
            tunnel: w1150 -> [w1293]
            tunnel: [w1292] -> w1165
            tunnel: w1139 -> [w1285]
            shift-right: [w1281] -> _
            shift-left: _ -> [w1291]
            tunnel: [w1279] -> _
            tunnel: w1146 -> [w1287]
            tunnel: w1140 -> [w1286]
            tunnel: w1134 -> [w1284]
            tunnel: w1133 -> [w1278]
            stop <- w1288 stop-if-true
            n477 = for {
              tunnel: w1293 -> [w1315]
              tunnel: w1294 -> [w1317]
              tunnel: w1298 -> [w1316] mode=indexing
              tunnel: w1297 -> [w1306]
              tunnel: w1296 -> [w1312]
              tunnel: w1295 -> [w1311]
              tunnel: [w1309] -> w1292
              tunnel: w1285 -> [w1307]
              tunnel: w1286 -> [w1308]
              tunnel: w1284 -> [w1305]
              tunnel: [w1302] -> w1283
              tunnel: w1278 -> [w1301]
              i -> [w1304]
              # "Read data"
              n478 = case shown="0" w1304 {
                tunnel: w1317 -> [_ w1339]
                tunnel: w1308 -> [w1323 w1338]
                tunnel: w1316 -> [w1321 w1336]
                tunnel: w1315 -> [w1324 w1335]
                tunnel: [w1325 w1334] -> w1314
                tunnel: [w1326 w1333] -> w1313
                tunnel: w1312 -> [w1330 _]
                tunnel: w1311 -> [w1329 _]
                tunnel: [w1322 _] -> w1310
                tunnel: w1307 -> [w1320 _]
                tunnel: w1305 -> [w1319 _]
                tunnel: w1301 -> [w1318 w1331]
                frame 0 {
                  # "Read files and queue it up."
                  n479 = call <instrlib>:"niScope Initiate Acquisition.vi"("instrument handle"=w1330) -> ("error out"=w1328:errorcluster)  [unwired: 2 in, 12 out]
                  n480 = call <instrlib>:"niScope Initiate Acquisition.vi"("instrument handle"=w1329, "error in"=w1328) -> ("error out"=w1327:errorcluster)  [unwired: 1 in, 12 out]
                  n481 = call "Rapid Read_NI.vi"("NI Card"=w1323, "Channel"=w1321, "Motion Board ID"=w1320, "rf points per line"=w1324, "error in"=w1327, "timeout"=w1318, "Pause?"=w1319) -> ("dig gain"=w1325:dbl, "Array"=w1326:i8[][], "Reverse?"=w1322:bool)  [unwired: 5 in, 1 out]
                }
                frame 1, Default {
                  n482 = property class="niScope"(reference=w1338, "Fetch Record Number"=0, "Fetch Number of Records"=w1339) -> (reference out=w1337:refnum<k15>, error out=w1332:errorcluster)  [unwired: 1 in]
                  n483 = call-poly <instrlib>:"niScope Fetch (poly).vi"("timeout"=w1331, "error in"=w1332, "numSamples"=w1335, "channels"=w1336, "instrument handle"=w1337) -> ("wfm"=w1333:i8[][], "wfm info"=w1342:T22)  [unwired: 5 out]
                  n484 = Index Array(array=w1342) -> (element=w1341:T23)  [unwired: 1 in]
                  n485 = Unbundle By Name(w1341) -> ("gain"=w1334:dbl)
                }
              }
              n486 = Bundle("gain"=w1314, "wfm"=w1313, "Reverse?"=w1310, w1304) -> (w1303:T24)  [unwired: 1 in]
              n487 = Enqueue Element(queue=w1306, element=w1303, timeout in ms (-1)=100) -> (queue out=w1309:refnum<queue>, error out=w1302:errorcluster)  [unwired: 1 in, 1 out]
            }
            n488 = Wait on Notification(notifier=w1287, timeout in ms (-1)=5) -> (timed out?=w1290:bool)  [unwired: 2 in, 3 out]
            n489 = flat-sequence {
              tunnel: [w1299] -> w1281
              tunnel: w1283 -> [_]
              frame #0 {
                n490 = Tick Count (ms)() -> (millisecond timer value=w1299:u32)
              }
            }
            n491 = Not(x=w1290) -> (.not. x?=w1288:bool)
            n492 = Subtract(x=w1281, y=w1291) -> (x-y=w1279:u32)
            n493 = call <vilib>:"Mean PtByPt.vi"("x"=w1279, "sample length"=20) -> ("mean"=w1280:dbl)  [unwired: 2 in, 1 out]
            n494 = local write "Read Loop"(w1280) -> ()
          }
          n495 = Release Queue(queue=w1165, force destroy? (F)=w1164) -> (error out=w1136:errorcluster)  [unwired: 1 in, 2 out]
          n496 = Delete Data Value Reference(data value reference=w1149) -> (error out=w1137:errorcluster)  [unwired: 1 in, 1 out]
        }
        frame "Drop Ch 5,4,3 XMIT" {
          w1347 = 2 ("index")
          w1376 = 4
          w1372 = 2 ("index")
          w1387 = 5
          w1378 = "0,1"
          # "Restructure file names"
          # "Read queue and send to files. About same as reading channel by channel"
          n497 = Reshape Array(w1388, w1387, w1387) -> (w1371:T19)
          n498 = Array To Cluster(array=w1360) -> (cluster=w1363:cluster{"[0]":void, "[1]":void, "[2]":void})
          n499 = Unbundle(w1363) -> ("[1]"=w1362, "[2]"=w1361)  [unwired: 1 out]
          n500 = expression code="x*2"(w1383) -> (w1389:dbl)
          n501 = Index Array(array=w1371, index (col)=4 ("index")) -> (element=w1350:T20)  [unwired: 1 in]
          n502 = Array Subset(array=w1371, length (row)=w1347, index (col)=w1372, length (col)=w1372) -> (w1375:T19)  [unwired: 1 in]
          n503 = Array Subset(array=w1371, length (row)=w1347, length (col)=2 ("index")) -> (w1374:T19)  [unwired: 2 in]
          n504 = call "RTHeader.vi"("Comment"="Drop 5,4,3 Xmit", "Votage scaling"=w1344) -> ("Header String Out"=w1367:string)  [unwired: 4 in, 1 out]
          n505 = Obtain Queue(max queue size (-1, unlimited)=3, element data type=w1345) -> (queue out=w1358:refnum<queue>)  [unwired: 3 in, 2 out]
          n506 = Array Subset(array=w1350, length=w1347) -> (w1349:T20)  [unwired: 1 in]
          n507 = Reshape Array(w1374, w1376) -> (w1377:T20)
          n508 = Reshape Array(w1375, w1376) -> (w1382:T20)
          n509 = Build Array(w1378, w1378, "1") -> (w1391:string[])
          n510 = Build Array(w1377, w1382, w1349) -> (w1381:T19)
          n511 = while {
            tunnel: w1358 -> [w1427]
            tunnel: w1370 -> [w1426]
            tunnel: [w1413] -> w1384
            tunnel: w1383 -> [w1425]
            tunnel: w1364 -> [w1422]
            tunnel: w1365 -> [w1424]
            tunnel: w1381 -> [w1420]
            tunnel: i32[] [4, 4, 2] -> [w1421]
            tunnel: w1355 -> [w1416]
            tunnel: [w1410] -> w1369
            tunnel: w1367 -> [w1415]
            tunnel: w1366 -> [w1411]
            tunnel: w1352 -> [w1398]
            tunnel: w1351 -> [w1397]
            tunnel: i16[] [1, 2, 2] -> [w1393]
            tunnel: w1343 -> [w1392]
            i -> [w1396]
            stop <- w1413 stop-if-true
            n512 = for {
              tunnel: w1426 -> [w1455]
              tunnel: w1425 -> [w1464]
              tunnel: w1427 -> [w1466]
              tunnel: [w1463] -> w1419 mode=indexing
              tunnel: [w1454] -> w1423
              tunnel: [w1450] -> w1417
              tunnel: w1422 -> [w1462]
              tunnel: w1420 -> [_] mode=indexing
              tunnel: w1421 -> [w1458]
              tunnel: w1420 -> [w1460]
              tunnel: w1416 -> [w1457]
              tunnel: w1415 -> [w1452]
              tunnel: [w1451] -> w1408 mode=indexing
              tunnel: [w1449] -> w1406 mode=indexing
              tunnel: w1398 -> [w1444]
              tunnel: w1397 -> [w1443]
              tunnel: w1396 -> [w1442]
              tunnel: [w1441] -> w1395 mode=indexing
              tunnel: w1393 -> [w1439]
              tunnel: w1392 -> [w1437]
              n513 = Dequeue Element(queue=w1466, timeout in ms (-1)=w1457) -> (element=w1447:T12, error out=w1448:errorcluster)  [unwired: 1 in, 2 out]
              n514 = flat-sequence {
                tunnel: [w1469] -> w1451
                tunnel: w1448 -> [_]
                tunnel: w1447 -> [w1468]
                tunnel: [w1468] -> w1446
                frame #0 {
                  n515 = Tick Count (ms)() -> (millisecond timer value=w1469:u32)
                }
              }
              n516 = Unbundle(w1446) -> ("gain"=w1454:dbl, "wfm"=w1453:i8[][], w1463:bool, "max queue size (-1, unlimited)"=w1440:i32)
              n517 = Index Array(array=w1458, index=w1440) -> (element=w1456:i32)
              n518 = Index Array(array=w1439, index=w1440) -> (element=w1438:i16)
              n519 = Index Array(array=w1460, index (row)=w1440) -> (element=w1459:T20)  [unwired: 1 in]
              n520 = Multiply(x=w1455, y=w1456) -> (x*y=w1461:i32)
              n521 = Reshape Array(w1453, w1464, w1461) -> (w1465:i8[][])
              n522 = Get Notifier Status(notifier=w1444) -> (current notification=w1445:bool)  [unwired: 1 in, 4 out]
              n523 = for {
                N: w1456 -> [_]
                tunnel: w1459 -> [w1484]
                tunnel: [w1487] -> w1450
                tunnel: w1462 -> [w1486]
                shift-right: [w1479] -> _
                shift-left: w1465 -> [w1488]
                tunnel: w1455 -> [w1482]
                tunnel: [w1477] -> w1441 mode=indexing
                tunnel: w1438 -> [w1476]
                tunnel: w1437 -> [w1475]
                i -> [w1485]
                n524 = Index Array(array=w1484, index=w1485) -> (element=w1480:T17)
                n525 = Delete From Array(array=w1488, length=w1482, index (col)=0 ("disabled index (col)")) -> (deleted portion=w1481:i8[], array with subset deleted=w1479:i8[][])  [unwired: 1 in]
                n526 = call "TimeShiftDataSubMean.vi"("Filter"=w1475, "output cluster"=w1480, "Array In"=w1481) -> ("Array Out"=w1478:i16[][], "Sat Pts"=w1477:i32)  [unwired: 2 in]
                n527 = in-place {
                  in-place-border: w1478 -> [w1491]
                  in-place-border: w1476 -> [w1489]
                  n528 = in-place-dvr #7(w1486) -> (w1492:i16[][])  [unwired: 1 out]
                  n529 = case shown="2" w1489 {
                    selector: w1489 -> [_ w1495]
                    tunnel: w1491 -> [w1494 w1497]
                    tunnel: [w1494 w1496] -> w1490
                    frame 0, Default {
                    }
                    frame 2 {
                      n530 = Multiply(x=w1495, y=w1497) -> (x*y=w1496:i16[][])
                    }
                  }
                  n531 = Add(x=w1490, y=w1492) -> (x+y=w1493:i16[][])
                  n532 = in-place-dvr #7(w1493) -> (w1487:refnum<data-value>)  [unwired: 1 out]
                }
              }
              n533 = case shown="True" w1445 {
                tunnel: w1440 -> [_ w1473]
                tunnel: w1453 -> [_ w1472]
                tunnel: w1452 -> [_ w1474]
                tunnel: w1443 -> [_ w1471]
                tunnel: w1442 -> [_ w1470]
                frame False {
                }
                frame True {
                  n534 = call "RawRT_Capture.vi"("Raw data"=w1472, "File Name In"=w1471, "DigCard"=w1473, "header"=w1474, "Iter"=w1470) -> ()  [unwired: 7 in]
                }
              }
              n535 = flat-sequence {
                tunnel: [w1467] -> w1449
                tunnel: w1450 -> [_]
                frame #0 {
                  n536 = Tick Count (ms)() -> (millisecond timer value=w1467:u32)
                }
              }
            }
            n537 = Wait on Notification(notifier=w1411, timeout in ms (-1)=5) -> (timed out?=w1414:bool)  [unwired: 2 in, 3 out]
            n538 = Add Array Elements(numeric array=w1395) -> (sum=w1394:i32)
            n539 = Subtract(x=w1406, y=w1408) -> (x-y=w1407:u32[])
            n540 = Not(x=w1414) -> (.not. x?=w1413:bool)
            n541 = Or Array Elements(Boolean array=w1419) -> (logical OR=w1418:bool)
            n542 = in-place {
              in-place-border: w1424 -> [w1436]
              in-place-border: w1418 -> [w1435]
              in-place-border: w1423 -> [w1434]
              in-place-border: w1394 -> [w1429]
              n543 = in-place-dvr #8(w1417) -> (w1430:i16[][])  [unwired: 1 out]
              n544 = Bundle("gain"=w1434, w1435, w1430, "Sat Pts"=w1429) -> (w1433:T21)  [unwired: 1 in]
              n545 = Multiply(x=i16 0, y=w1430) -> (x*y=w1432:i16[][])
              n546 = Lossy Enqueue Element(queue=w1436, element=w1433) -> ()  [unwired: 1 in, 4 out]
              n547 = in-place-dvr #8(w1432) -> (w1410:refnum<data-value>)  [unwired: 1 out]
            }
            n548 = Index Array(array=w1406, index=2) -> (element=w1404:u32)
            n549 = Add Array Elements(numeric array=w1407) -> (sum=w1403:u32)
            n550 = Subtract(x=w1409, y=w1404) -> (x-y=w1402:u32)
            n551 = Add(x=w1402, y=w1403) -> (x+y=w1401:u32)
            n552 = flat-sequence {
              tunnel: [w1428] -> w1409
              tunnel: w1410 -> [_]
              frame #0 {
                n553 = Tick Count (ms)() -> (millisecond timer value=w1428:u32)
              }
            }
            n554 = call <vilib>:"Mean PtByPt.vi"("x"=w1401, "sample length"=20) -> ("mean"=w1399:dbl)  [unwired: 2 in, 1 out]
            n555 = local write "SF Loop"(w1399) -> ()
          }
          n556 = while {
            tunnel: w1391 -> [w1518]
            tunnel: w1358 -> [w1517]
            tunnel: w1362 -> [w1516]
            tunnel: w1361 -> [w1515]
            tunnel: w1389 -> [w1514]
            tunnel: w1370 -> [w1513]
            tunnel: [w1512] -> w1385
            tunnel: w1359 -> [w1505]
            shift-right: [w1501] -> _
            shift-left: _ -> [w1511]
            tunnel: [w1499] -> _
            tunnel: w1366 -> [w1507]
            tunnel: w1360 -> [w1506]
            tunnel: w1354 -> [w1504]
            tunnel: w1353 -> [w1498]
            stop <- w1508 stop-if-true
            n557 = for {
              tunnel: w1513 -> [w1535]
              tunnel: w1514 -> [w1537]
              tunnel: w1518 -> [w1536] mode=indexing
              tunnel: w1517 -> [w1526]
              tunnel: w1516 -> [w1532]
              tunnel: w1515 -> [w1531]
              tunnel: [w1529] -> w1512
              tunnel: w1505 -> [w1527]
              tunnel: w1506 -> [w1528]
              tunnel: w1504 -> [w1525]
              tunnel: [w1522] -> w1503
              tunnel: w1498 -> [w1521]
              i -> [w1524]
              # "Read data"
              n558 = case shown="1, Default" w1524 {
                tunnel: w1537 -> [_ w1559]
                tunnel: w1528 -> [w1543 w1558]
                tunnel: w1536 -> [w1541 w1556]
                tunnel: w1535 -> [w1544 w1555]
                tunnel: [w1545 w1554] -> w1534
                tunnel: [w1546 w1553] -> w1533
                tunnel: w1532 -> [w1550 _]
                tunnel: w1531 -> [w1549 _]
                tunnel: [w1542 _] -> w1530
                tunnel: w1527 -> [w1540 _]
                tunnel: w1525 -> [w1539 _]
                tunnel: w1521 -> [w1538 w1551]
                frame 0 {
                  # "Read files and queue it up."
                  n559 = call <instrlib>:"niScope Initiate Acquisition.vi"("instrument handle"=w1550) -> ("error out"=w1548:errorcluster)  [unwired: 2 in, 12 out]
                  n560 = call <instrlib>:"niScope Initiate Acquisition.vi"("instrument handle"=w1549, "error in"=w1548) -> ("error out"=w1547:errorcluster)  [unwired: 1 in, 12 out]
                  n561 = call "Rapid Read_NI.vi"("NI Card"=w1543, "Channel"=w1541, "Motion Board ID"=w1540, "rf points per line"=w1544, "error in"=w1547, "timeout"=w1538, "Pause?"=w1539) -> ("dig gain"=w1545:dbl, "Array"=w1546:i8[][], "Reverse?"=w1542:bool)  [unwired: 5 in, 1 out]
                }
                frame 1, Default {
                  n562 = property class="niScope"(reference=w1558, "Fetch Record Number"=0, "Fetch Number of Records"=w1559) -> (reference out=w1557:refnum<k15>, error out=w1552:errorcluster)  [unwired: 1 in]
                  n563 = call-poly <instrlib>:"niScope Fetch (poly).vi"("timeout"=w1551, "error in"=w1552, "numSamples"=w1555, "channels"=w1556, "instrument handle"=w1557) -> ("wfm"=w1553:i8[][], "wfm info"=w1562:T22)  [unwired: 5 out]
                  n564 = Index Array(array=w1562) -> (element=w1561:T23)  [unwired: 1 in]
                  n565 = Unbundle By Name(w1561) -> ("gain"=w1554:dbl)
                }
              }
              n566 = Bundle("gain"=w1534, "wfm"=w1533, "Reverse?"=w1530, w1524) -> (w1523:T24)  [unwired: 1 in]
              n567 = Enqueue Element(queue=w1526, element=w1523, timeout in ms (-1)=100) -> (queue out=w1529:refnum<queue>, error out=w1522:errorcluster)  [unwired: 1 in, 1 out]
            }
            n568 = Wait on Notification(notifier=w1507, timeout in ms (-1)=5) -> (timed out?=w1510:bool)  [unwired: 2 in, 3 out]
            n569 = flat-sequence {
              tunnel: [w1519] -> w1501
              tunnel: w1503 -> [_]
              frame #0 {
                n570 = Tick Count (ms)() -> (millisecond timer value=w1519:u32)
              }
            }
            n571 = Not(x=w1510) -> (.not. x?=w1508:bool)
            n572 = Subtract(x=w1501, y=w1511) -> (x-y=w1499:u32)
            n573 = call <vilib>:"Mean PtByPt.vi"("x"=w1499, "sample length"=20) -> ("mean"=w1500:dbl)  [unwired: 2 in, 1 out]
            n574 = local write "Read Loop"(w1500) -> ()
          }
          n575 = Release Queue(queue=w1385, force destroy? (F)=w1384) -> (error out=w1356:errorcluster)  [unwired: 1 in, 2 out]
          n576 = Delete Data Value Reference(data value reference=w1369) -> (error out=w1357:errorcluster)  [unwired: 1 in, 1 out]
        }
        frame "test" {
          w1594 = 10
          w1589 = 2 ("index")
          w1603 = 5
          # "Restructure file names"
          # "Read queue and send to files. About same as reading channel by channel"
          n577 = Reshape Array(w1604, w1603, w1603) -> (w1587:T19)
          n578 = Array To Cluster(array=w1576) -> (cluster=w1579:cluster{"[0]":void, "[1]":void, "[2]":void})
          n579 = Unbundle(w1579) -> ("[0]"=w1569, "[1]"=w1578, "[2]"=w1577)
          n580 = Index Array(array=w1587, index (col)=4 ("index")) -> (element=w1593:T20)  [unwired: 1 in]
          n581 = Array Subset(array=w1587, index (col)=w1589, length (col)=w1589) -> (w1592:T19)  [unwired: 2 in]
          n582 = Array Subset(array=w1587, length (col)=2 ("index")) -> (w1591:T19)  [unwired: 3 in]
          n583 = call "RTHeader.vi"("Comment"="Full 25", "Votage scaling"=w1564) -> ("Header String Out"=w1583:string)  [unwired: 4 in, 1 out]
          n584 = Obtain Queue(max queue size (-1, unlimited)=3, element data type=w1565) -> (queue out=w1574:refnum<queue>)  [unwired: 3 in, 2 out]
          n585 = Reshape Array(w1591, w1594) -> (w1595:T20)
          n586 = Reshape Array(w1592, w1594) -> (w1598:T20)
          n587 = Build Array(w1595, w1598, w1593) -> (w1597:T19)
          n588 = while {
            tunnel: w1574 -> [w1640]
            tunnel: w1586 -> [w1639]
            tunnel: [w1626] -> w1600
            tunnel: w1599 -> [w1638]
            tunnel: w1580 -> [w1635]
            tunnel: w1581 -> [w1637]
            tunnel: w1597 -> [w1633]
            tunnel: i32[] [10, 10, 5] -> [w1634]
            tunnel: w1571 -> [w1629]
            tunnel: [w1623] -> w1585
            tunnel: w1583 -> [w1628]
            tunnel: w1582 -> [w1624]
            tunnel: w1567 -> [w1611]
            tunnel: w1566 -> [w1610]
            tunnel: w1563 -> [w1606]
            i -> [w1609]
            stop <- w1626 stop-if-true
            n589 = for {
              tunnel: w1639 -> [w1666]
              tunnel: w1638 -> [w1675]
              tunnel: w1640 -> [w1677]
              tunnel: [w1674] -> w1632 mode=indexing
              tunnel: [w1665] -> w1636
              tunnel: [w1660] -> w1630
              tunnel: w1635 -> [w1673]
              tunnel: w1633 -> [_] mode=indexing
              tunnel: w1634 -> [w1669]
              tunnel: w1633 -> [w1671]
              tunnel: w1629 -> [w1668]
              tunnel: w1628 -> [w1663]
              tunnel: [w1661] -> w1621 mode=indexing
              tunnel: [w1659] -> w1619 mode=indexing
              tunnel: w1611 -> [w1655]
              tunnel: w1610 -> [w1653]
              tunnel: w1609 -> [w1652]
              tunnel: [w1651] -> w1608 mode=indexing
              tunnel: w1606 -> [w1650]
              n590 = Dequeue Element(queue=w1677, timeout in ms (-1)=w1668) -> (element=w1657:T12, error out=w1658:errorcluster)  [unwired: 1 in, 2 out]
              n591 = flat-sequence {
                tunnel: [w1680] -> w1661
                tunnel: w1658 -> [_]
                tunnel: w1657 -> [w1679]
                tunnel: [w1679] -> w1656
                frame #0 {
                  n592 = Tick Count (ms)() -> (millisecond timer value=w1680:u32)
                }
              }
              n593 = Unbundle(w1656) -> ("gain"=w1665:dbl, "wfm"=w1664:i8[][], w1674:bool, "max queue size (-1, unlimited)"=w1662:i32)
              n594 = Index Array(array=w1669, index=w1662) -> (element=w1667:i32)
              n595 = Index Array(array=w1671, index (row)=w1662) -> (element=w1670:T20)  [unwired: 1 in]
              n596 = Multiply(x=w1666, y=w1667) -> (x*y=w1672:i32)
              n597 = Reshape Array(w1664, w1675, w1672) -> (w1676:i8[][])
              n598 = Get Notifier Status(notifier=w1653) -> (current notification=w1654:bool)  [unwired: 1 in, 4 out]
              n599 = for {
                N: w1667 -> [_]
                tunnel: w1670 -> [w1694]
                tunnel: [w1697] -> w1660
                tunnel: w1673 -> [w1696]
                shift-right: [w1692] -> _
                shift-left: w1676 -> [w1698]
                tunnel: w1666 -> [w1691]
                tunnel: [w1687] -> w1651 mode=indexing
                tunnel: w1650 -> [w1686]
                i -> [w1695]
                n600 = Index Array(array=w1694, index=w1695) -> (element=w1688:T17)
                n601 = Delete From Array(array=w1698, length=w1691, index (col)=0 ("disabled index (col)")) -> (deleted portion=w1690:i8[], array with subset deleted=w1692:i8[][])  [unwired: 1 in]
                n602 = call "TimeShiftDataSubMean.vi"("Filter"=w1686, "output cluster"=w1688, "Array In"=w1690) -> ("Array Out"=w1689:i16[][], "Sat Pts"=w1687:i32)  [unwired: 2 in]
                n603 = in-place {
                  in-place-border: w1689 -> [w1701]
                  n604 = in-place-dvr #9(w1696) -> (w1699:i16[][])  [unwired: 1 out]
                  n605 = Add(x=w1701, y=w1699) -> (x+y=w1700:i16[][])
                  n606 = in-place-dvr #9(w1700) -> (w1697:refnum<data-value>)  [unwired: 1 out]
                }
              }
              n607 = case shown="True" w1654 {
                tunnel: w1662 -> [_ w1685]
                tunnel: w1664 -> [_ w1684]
                tunnel: w1663 -> [_ w1682]
                tunnel: w1655 -> [_ w1683]
                tunnel: w1652 -> [_ w1681]
                frame False {
                }
                frame True {
                  n608 = call "RawRT_Capture.vi"("Raw data"=w1684, "File Name In"=w1683, "DigCard"=w1685, "header"=w1682, "Iter"=w1681) -> ()  [unwired: 7 in]
                }
              }
              n609 = flat-sequence {
                tunnel: [w1678] -> w1659
                tunnel: w1660 -> [_]
                frame #0 {
                  n610 = Tick Count (ms)() -> (millisecond timer value=w1678:u32)
                }
              }
            }
            n611 = Wait on Notification(notifier=w1624, timeout in ms (-1)=5) -> (timed out?=w1627:bool)  [unwired: 2 in, 3 out]
            n612 = Add Array Elements(numeric array=w1608) -> (sum=w1607:i32)
            n613 = Subtract(x=w1619, y=w1621) -> (x-y=w1620:u32[])
            n614 = Not(x=w1627) -> (.not. x?=w1626:bool)
            n615 = Or Array Elements(Boolean array=w1632) -> (logical OR=w1631:bool)
            n616 = in-place {
              in-place-border: w1637 -> [w1649]
              in-place-border: w1631 -> [w1648]
              in-place-border: w1636 -> [w1647]
              in-place-border: w1607 -> [w1642]
              n617 = in-place-dvr #10(w1630) -> (w1643:i16[][])  [unwired: 1 out]
              n618 = Bundle("gain"=w1647, w1648, w1643, "Sat Pts"=w1642) -> (w1646:T21)  [unwired: 1 in]
              n619 = Multiply(x=i16 0, y=w1643) -> (x*y=w1645:i16[][])
              n620 = Lossy Enqueue Element(queue=w1649, element=w1646) -> ()  [unwired: 1 in, 4 out]
              n621 = in-place-dvr #10(w1645) -> (w1623:refnum<data-value>)  [unwired: 1 out]
            }
            n622 = Index Array(array=w1619, index=2) -> (element=w1617:u32)
            n623 = Add Array Elements(numeric array=w1620) -> (sum=w1616:u32)
            n624 = Subtract(x=w1622, y=w1617) -> (x-y=w1615:u32)
            n625 = Add(x=w1615, y=w1616) -> (x+y=w1614:u32)
            n626 = flat-sequence {
              tunnel: [w1641] -> w1622
              tunnel: w1623 -> [_]
              frame #0 {
                n627 = Tick Count (ms)() -> (millisecond timer value=w1641:u32)
              }
            }
            n628 = call <vilib>:"Mean PtByPt.vi"("x"=w1614, "sample length"=20) -> ("mean"=w1612:dbl)  [unwired: 2 in, 1 out]
            n629 = local write "SF Loop"(w1612) -> ()
          }
          n630 = while {
            tunnel: w1574 -> [w1709]
            tunnel: w1578 -> [w1718]
            tunnel: w1577 -> [w1717]
            tunnel: w1586 -> [w1716]
            tunnel: [w1750] -> w1601
            tunnel: w1575 -> [w1732]
            shift-right: [w1742] -> _
            shift-left: _ -> [w1749]
            tunnel: [w1740] -> _
            tunnel: w1582 -> [w1745]
            tunnel: w1570 -> [w1744]
            tunnel: w1569 -> [w1734]
            tunnel: w1568 -> [w1702]
            stop <- w1746 stop-if-true
            w1719 = -1
            # "Read files and queue it up."
            # "Read data"
            n631 = call <instrlib>:"niScope Initiate Acquisition.vi"("instrument handle"=w1718) -> ("error out"=w1736:errorcluster)  [unwired: 2 in, 12 out]
            n632 = call <instrlib>:"niScope Initiate Acquisition.vi"("instrument handle"=w1717, "error in"=w1736) -> ("error out"=w1705:errorcluster)  [unwired: 1 in, 12 out]
            n633 = property class="niScope"(reference=w1718, error in=w1705, "Fetch Record Number"=0, "Fetch Number of Records"=w1719) -> (reference out=w1729:refnum<k15>, error out=w1728:errorcluster)
            n634 = property class="niScope"(reference=w1717, error in=w1705, "Fetch Record Number"=0, "Fetch Number of Records"=w1719) -> (reference out=w1724:refnum<k15>, error out=w1723:errorcluster)
            n635 = call-poly <instrlib>:"niScope Fetch (poly).vi"("timeout"=w1702, "error in"=w1728, "numSamples"=w1716, "channels"="0,1", "instrument handle"=w1729) -> ("wfm"=w1708:i8[][], "wfm info"=w1731:T22)  [unwired: 5 out]
            n636 = call "Rapid Read_NI.vi"("NI Card"=w1734, "Channel"="0,1", "Motion Board ID"=w1732, "rf points per line"=w1716, "error in"=w1705, "timeout"=w1702, "Pause?"=w1744) -> ("dig gain"=w1739:dbl, "Array"=w1738:i8[][], "Reverse?"=w1707:bool)  [unwired: 5 in, 1 out]
            n637 = call-poly <instrlib>:"niScope Fetch (poly).vi"("timeout"=w1702, "error in"=w1723, "numSamples"=w1716, "channels"="1", "instrument handle"=w1724) -> ("wfm"=w1713:i8[][], "wfm info"=w1726:T22)  [unwired: 5 out]
            n638 = Index Array(array=w1731) -> (element=w1730:T23)  [unwired: 1 in]
            n639 = Unbundle By Name(w1730) -> ("gain"=w1711:dbl)
            n640 = Index Array(array=w1726) -> (element=w1725:T23)  [unwired: 1 in]
            n641 = Unbundle By Name(w1725) -> ("gain"=w1712:dbl)
            n642 = Wait on Notification(notifier=w1745, timeout in ms (-1)=5) -> (timed out?=w1748:bool)  [unwired: 2 in, 3 out]
            n643 = flat-sequence {
              tunnel: [w1751] -> w1742
              tunnel: w1703 -> [_]
              frame #0 {
                n644 = Tick Count (ms)() -> (millisecond timer value=w1751:u32)
              }
            }
            n645 = Not(x=w1748) -> (.not. x?=w1746:bool)
            n646 = Bundle("gain"=w1712, "wfm"=w1713, "Reverse?"=w1707, 2) -> (w1710:T24)  [unwired: 1 in]
            n647 = Bundle("dig gain"=w1739, "Array"=w1738, "Reverse?"=w1707, 0) -> (w1737:T25)  [unwired: 1 in]
            n648 = Bundle("gain"=w1711, "wfm"=w1708, "Reverse?"=w1707, 1) -> (w1706:T24)  [unwired: 1 in]
            n649 = Subtract(x=w1742, y=w1749) -> (x-y=w1740:u32)
            n650 = Enqueue Element(queue=w1709, element=w1737) -> (queue out=w1750:refnum<queue>, error out=w1704:errorcluster)  [unwired: 2 in, 1 out]
            n651 = Enqueue Element(queue=w1709, element=w1706, error in (no error)=w1704) -> ()  [unwired: 1 in, 3 out]
            n652 = Enqueue Element(queue=w1709, element=w1710, error in (no error)=w1704) -> (error out=w1703:errorcluster)  [unwired: 1 in, 2 out]
            n653 = call <vilib>:"Mean PtByPt.vi"("x"=w1740, "sample length"=20) -> ("mean"=w1741:dbl)  [unwired: 2 in, 1 out]
            n654 = local write "Read Loop"(w1741) -> ()
          }
          n655 = Release Queue(queue=w1601, force destroy? (F)=w1600) -> (error out=w1572:errorcluster)  [unwired: 1 in, 2 out]
          n656 = Delete Data Value Reference(data value reference=w1585) -> (error out=w1573:errorcluster)  [unwired: 1 in, 1 out]
        }
        frame "Drop Ch 5" {
          w1779 = 2 ("index")
          w1791 = 5
          # "Reduced data case that drop ring 5 receive"
          # "Restructure file names"
          # "Read queue and send to files. About same as reading channel by channel"
          n657 = Array To Cluster(array=w1765) -> (cluster=w1766:cluster{"[0]":void, "[1]":void, "[2]":void})
          n658 = Reshape Array(w1792, w1791, w1791) -> (w1777:T19)
          n659 = Unbundle(w1766) -> ("[0]"=w1764, "[1]"=w1763)  [unwired: 1 out]
          n660 = Array Subset(array=w1777, index (col)=w1779, length (col)=w1779) -> (w1778:T19)  [unwired: 2 in]
          n661 = Array Subset(array=w1777, length (col)=2 ("index")) -> (w1781:T19)  [unwired: 3 in]
          n662 = expression code="x*5"(w1774) -> (w1771:dbl)
          n663 = Obtain Queue(max queue size (-1, unlimited)=2, element data type=w1754) -> (queue out=w1794:refnum<queue>)  [unwired: 3 in, 2 out]
          n664 = Build Array(w1764, w1763) -> (w1773:void[])
          n665 = call "RTHeader.vi"("Comment"="Drop 5", "Votage scaling"=w1753) -> ("Header String Out"=w1755:string)  [unwired: 4 in, 1 out]
          n666 = Reshape Array(w1781, 10) -> (w1780:T20)
          n667 = Reshape Array(w1778, 10) -> (w1788:T20)
          n668 = Build Array(w1780, w1788) -> (w1787:T19)
          n669 = while {
            tunnel: w1794 -> [w1831]
            tunnel: w1776 -> [w1830]
            tunnel: w1774 -> [w1829]
            tunnel: w1767 -> [w1826]
            tunnel: w1770 -> [w1828]
            tunnel: w1787 -> [w1796]
            tunnel: i32[] [10, 10] -> [w1825]
            tunnel: w1760 -> [w1822]
            tunnel: i16[] [1, 1, 1, 1, 1, 1, 1, 1, 2, 2] -> [w1821]
            tunnel: [w1814] -> w1775
            tunnel: w1769 -> [w1819]
            tunnel: [w1816] -> w1762
            tunnel: w1758 -> [w1804]
            tunnel: w1757 -> [w1803]
            tunnel: w1755 -> [w1802]
            tunnel: w1752 -> [w1795]
            i -> [w1801]
            stop <- w1818 stop-if-true
            n670 = for {
              tunnel: w1830 -> [w1860]
              tunnel: w1829 -> [w1868]
              tunnel: w1831 -> [w1870]
              tunnel: [w1867] -> w1824 mode=indexing
              tunnel: [w1866] -> w1827
              tunnel: [w1855] -> w1800
              tunnel: w1826 -> [w1843]
              tunnel: w1796 -> [_] mode=indexing
              tunnel: w1825 -> [w1863]
              tunnel: w1796 -> [w1865]
              tunnel: w1822 -> [w1862]
              tunnel: w1821 -> [w1859]
              tunnel: [w1857] -> w1816
              tunnel: [w1856] -> w1812 mode=indexing
              tunnel: [w1854] -> w1810 mode=indexing
              tunnel: w1804 -> [w1849]
              tunnel: w1803 -> [w1848]
              tunnel: w1802 -> [w1845]
              tunnel: w1801 -> [w1844]
              tunnel: [w1842] -> w1798 mode=indexing
              tunnel: w1795 -> [w1841]
              n671 = Dequeue Element(queue=w1870, timeout in ms (-1)=w1862) -> (queue out=w1857:refnum<queue>, element=w1852:T12, error out=w1853:errorcluster)  [unwired: 1 in, 1 out]
              n672 = Unbundle(w1851) -> ("gain"=w1866:dbl, "wfm"=w1869:i8[][], w1867:bool, "max queue size (-1, unlimited)"=w1846:i32)
              n673 = Index Array(array=w1863, index=w1846) -> (element=w1861:i32)
              n674 = Index Array(array=w1865, index (row)=w1846) -> (element=w1864:T20)  [unwired: 1 in]
              n675 = Multiply(x=w1860, y=w1861) -> (x*y=w1858:i32)
              n676 = flat-sequence {
                tunnel: [w1878] -> w1856
                tunnel: w1853 -> [_]
                tunnel: w1852 -> [w1877]
                tunnel: [w1877] -> w1851
                frame #0 {
                  n677 = Tick Count (ms)() -> (millisecond timer value=w1878:u32)
                }
              }
              n678 = Reshape Array(w1869, w1868, w1858) -> (w1847:i8[][])
              n679 = for {
                N: w1861 -> [_]
                tunnel: w1864 -> [w1888]
                tunnel: [w1891] -> w1855
                tunnel: w1843 -> [w1890]
                shift-right: [w1884] -> _
                shift-left: w1847 -> [w1892]
                tunnel: w1859 -> [w1886] mode=indexing
                tunnel: w1860 -> [w1885]
                tunnel: [w1880] -> w1842 mode=indexing
                tunnel: w1841 -> [w1879]
                i -> [w1889]
                n680 = Index Array(array=w1888, index=w1889) -> (element=w1882:T17)
                n681 = Delete From Array(array=w1892, length=w1885, index (col)=0 ("disabled index (col)")) -> (deleted portion=w1883:i8[], array with subset deleted=w1884:i8[][])  [unwired: 1 in]
                n682 = call "TimeShiftDataSubMean.vi"("Filter"=w1879, "output cluster"=w1882, "Array In"=w1883) -> ("Array Out"=w1881:i16[][], "Sat Pts"=w1880:i32)  [unwired: 2 in]
                n683 = in-place {
                  in-place-border: w1881 -> [w1894]
                  in-place-border: w1886 -> [w1895]
                  n684 = in-place-dvr #11(w1890) -> (w1896:i16[][])  [unwired: 1 out]
                  n685 = case shown="2" w1895 {
                    selector: w1895 -> [_ w1899]
                    tunnel: w1894 -> [w1898 w1901]
                    tunnel: [w1898 w1900] -> w1893
                    frame 0, Default {
                    }
                    frame 2 {
                      n686 = Multiply(x=w1899, y=w1901) -> (x*y=w1900:i16[][])
                    }
                  }
                  n687 = Add(x=w1893, y=w1896) -> (x+y=w1897:i16[][])
                  n688 = in-place-dvr #11(w1897) -> (w1891:refnum<data-value>)  [unwired: 1 out]
                }
              }
              n689 = Get Notifier Status(notifier=w1849) -> (current notification=w1850:bool)  [unwired: 1 in, 4 out]
              n690 = case shown="True" w1850 {
                tunnel: w1846 -> [_ w1875]
                tunnel: w1847 -> [_ w1874]
                tunnel: w1848 -> [_ w1873]
                tunnel: w1845 -> [_ w1872]
                tunnel: w1844 -> [_ w1871]
                frame False {
                }
                frame True {
                  n691 = call "RawRT_Capture.vi"("Raw data"=w1874, "File Name In"=w1873, "DigCard"=w1875, "header"=w1872, "Iter"=w1871) -> ()  [unwired: 7 in]
                }
              }
              n692 = flat-sequence {
                tunnel: [w1876] -> w1854
                tunnel: w1855 -> [_]
                frame #0 {
                  n693 = Tick Count (ms)() -> (millisecond timer value=w1876:u32)
                }
              }
            }
            n694 = Wait on Notification(notifier=w1819, timeout in ms (-1)=5) -> (timed out?=w1817:bool)  [unwired: 2 in, 3 out]
            n695 = Not(x=w1817) -> (.not. x?=w1818:bool)
            n696 = Add Array Elements(numeric array=w1798) -> (sum=w1797:i32)
            n697 = Or Array Elements(Boolean array=w1824) -> (logical OR=w1823:bool)
            n698 = in-place {
              in-place-border: w1828 -> [w1840]
              in-place-border: w1823 -> [w1839]
              in-place-border: w1827 -> [w1838]
              in-place-border: w1797 -> [w1833]
              n699 = in-place-dvr #12(w1800) -> (w1834:i16[][])  [unwired: 1 out]
              n700 = Bundle("gain"=w1838, w1839, w1834, "Sat Pts"=w1833) -> (w1837:T21)  [unwired: 1 in]
              n701 = Multiply(x=i16 0, y=w1834) -> (x*y=w1836:i16[][])
              n702 = Lossy Enqueue Element(queue=w1840, element=w1837) -> ()  [unwired: 1 in, 4 out]
              n703 = in-place-dvr #12(w1836) -> (w1814:refnum<data-value>)  [unwired: 1 out]
            }
            n704 = Index Array(array=w1810, index=1) -> (element=w1815:u32)
            n705 = Subtract(x=w1810, y=w1812) -> (x-y=w1811:u32[])
            n706 = Subtract(x=w1813, y=w1815) -> (x-y=w1807:u32)
            n707 = Add Array Elements(numeric array=w1811) -> (sum=w1808:u32)
            n708 = flat-sequence {
              tunnel: [w1832] -> w1813
              tunnel: w1814 -> [_]
              frame #0 {
                n709 = Tick Count (ms)() -> (millisecond timer value=w1832:u32)
              }
            }
            n710 = Add(x=w1807, y=w1808) -> (x+y=w1805:u32)
            n711 = call <vilib>:"Mean PtByPt.vi"("x"=w1805, "sample length"=20) -> ("mean"=→"SF Loop":dbl)  [unwired: 2 in, 1 out]
          }
          n712 = while {
            tunnel: w1773 -> [w1920]
            tunnel: w1794 -> [w1919]
            tunnel: w1763 -> [w1918]
            tunnel: w1776 -> [w1917]
            tunnel: w1789 -> [w1916]
            shift-right: [w1907] -> _
            shift-left: _ -> [w1915]
            tunnel: [w1904] -> _
            tunnel: "0,1" -> [w1914]
            tunnel: w1771 -> [w1913]
            tunnel: w1769 -> [w1911]
            tunnel: [w1910] -> w1768
            tunnel: w1761 -> [w1908]
            tunnel: w1759 -> [w1902]
            stop <- w1910 stop-if-true
            n713 = for {
              tunnel: w1917 -> [w1934]
              tunnel: w1920 -> [w1936] mode=indexing
              tunnel: w1914 -> [w1935]
              tunnel: w1919 -> [w1933]
              tunnel: w1918 -> [w1930]
              tunnel: w1916 -> [w1927]
              tunnel: w1913 -> [w1928]
              tunnel: w1908 -> [w1926]
              tunnel: [w1923] -> w1906
              tunnel: w1902 -> [w1922]
              i -> [w1925]
              # "Read data"
              n714 = case shown="0" w1925 {
                tunnel: w1936 -> [w1944 w1953]
                tunnel: w1935 -> [w1942 w1952]
                tunnel: w1934 -> [w1945 w1956]
                tunnel: [w1946 w1955] -> w1932
                tunnel: [w1939 w1951] -> w1931
                tunnel: w1930 -> [w1947 _]
                tunnel: [w1943 _] -> w1929
                tunnel: w1927 -> [w1941 _]
                tunnel: w1928 -> [_ w1949]
                tunnel: w1926 -> [w1938 _]
                tunnel: w1922 -> [w1937 w1948]
                frame 0 {
                  # "Read files and queue it up."
                  n715 = call <instrlib>:"niScope Initiate Acquisition.vi"("instrument handle"=w1947) -> ("error out"=w1940:errorcluster)  [unwired: 2 in, 12 out]
                  n716 = call "Rapid Read_NI.vi"("NI Card"=w1944, "Channel"=w1942, "Motion Board ID"=w1941, "rf points per line"=w1945, "error in"=w1940, "timeout"=w1937, "Pause?"=w1938) -> ("dig gain"=w1946:dbl, "Array"=w1939:i8[][], "Reverse?"=w1943:bool)  [unwired: 5 in, 1 out]
                }
                frame 1, Default {
                  n717 = property class="niScope"(reference=w1953, "Fetch Record Number"=0, "Fetch Number of Records"=w1949) -> (reference out=w1957:refnum<k15>, error out=w1954:errorcluster)  [unwired: 1 in]
                  n718 = call-poly <instrlib>:"niScope Fetch (poly).vi"("timeout"=w1948, "error in"=w1954, "numSamples"=w1956, "channels"=w1952, "instrument handle"=w1957) -> ("wfm"=w1951:i8[][], "wfm info"=w1959:T22)  [unwired: 5 out]
                  n719 = Index Array(array=w1959) -> (element=w1958:T23)  [unwired: 1 in]
                  n720 = Unbundle By Name(w1958) -> ("gain"=w1955:dbl)
                }
              }
              n721 = Bundle("gain"=w1932, "wfm"=w1931, "Reverse?"=w1929, w1925) -> (w1924:T24)  [unwired: 1 in]
              n722 = Enqueue Element(queue=w1933, element=w1924) -> (error out=w1923:errorcluster)  [unwired: 2 in, 2 out]
            }
            n723 = Wait on Notification(notifier=w1911, timeout in ms (-1)=5) -> (timed out?=w1909:bool)  [unwired: 2 in, 3 out]
            n724 = flat-sequence {
              tunnel: [w1921] -> w1907
              tunnel: w1906 -> [_]
              frame #0 {
                n725 = Tick Count (ms)() -> (millisecond timer value=w1921:u32)
              }
            }
            n726 = Not(x=w1909) -> (.not. x?=w1910:bool)
            n727 = Subtract(x=w1907, y=w1915) -> (x-y=w1904:u32)
            n728 = call <vilib>:"Mean PtByPt.vi"("x"=w1904, "sample length"=20) -> ("mean"=→"Read Loop":dbl)  [unwired: 2 in, 1 out]
          }
          n729 = Release Queue(queue=w1762, force destroy? (F)=w1768) -> ()  [unwired: 1 in, 3 out]
          n730 = Delete Data Value Reference(data value reference=w1775) -> ()  [unwired: 1 in, 2 out]
        }
        frame "Drop Ch 5,4" {
          w2007 = 5
          # "Reduced data case that drop ring 4,5 receive"
          # "Restructure file names"
          # "Read queue and send to files. About same as reading channel by channel"
          n731 = Array To Cluster(array=w1979) -> (cluster=w1980:cluster{"[0]":void, "[1]":void, "[2]":void})
          n732 = Reshape Array(w2008, w2007, w2007) -> (w1992:T19)
          n733 = Unbundle(w1980) -> ("[0]"=w1978, "[1]"=w1972)  [unwired: 1 out]
          n734 = Array Subset(array=w1992, index (col)=2 ("index"), length (col)=1 ("index")) -> (w1993:T19)  [unwired: 2 in]
          n735 = Array Subset(array=w1992, length (col)=2 ("index")) -> (w1996:T19)  [unwired: 3 in]
          n736 = call "RTHeader.vi"("Comment"="Drop 4,5", "Votage scaling"=w1961) -> ("Header String Out"=w1963:string)  [unwired: 4 in, 1 out]
          n737 = Obtain Queue(max queue size (-1, unlimited)=2, element data type=w1962) -> (queue out=w2010:refnum<queue>)  [unwired: 3 in, 2 out]
          n738 = property class="niScope"(reference=w1972, "Active Channel"="1", "Channel Enabled"=FALSE ("Vertical:Channel Enabled")) -> (reference out=w1971:refnum<k15>)  [unwired: 1 in, 1 out]
          n739 = Build Array(w1978, w1972) -> (w1988:void[])
          n740 = Reshape Array(w1996, 10) -> (w1995:T20)
          n741 = Reshape Array(w1993, 5) -> (w2003:T20)
          n742 = expression code="x*5"(w1989) -> (w1987:dbl)
          n743 = Build Array(w1995, w2003) -> (w2002:T19)
          n744 = while {
            tunnel: w2010 -> [w2047]
            tunnel: w1991 -> [w2046]
            tunnel: w1989 -> [w2045]
            tunnel: w1981 -> [w2042]
            tunnel: w1983 -> [w2044]
            tunnel: w2002 -> [w2018]
            tunnel: i32[] [10, 5] -> [w2041]
            tunnel: w1976 -> [w2037]
            tunnel: i16[] [1, 1, 1, 1, 1, 1, 2, 2, 2, 2] -> [w2036]
            tunnel: [w2029] -> w1990
            tunnel: i16[] [1, 1, 1, 2, 2] -> [w2035]
            tunnel: w1982 -> [w2033]
            tunnel: [w2031] -> w1977
            tunnel: w1966 -> [w2017]
            tunnel: w1965 -> [w2016]
            tunnel: w1963 -> [w2014]
            tunnel: w1960 -> [w2011]
            i -> [w2015]
            stop <- w2031 stop-if-true
            n745 = for {
              tunnel: w2046 -> [w2076]
              tunnel: w2045 -> [w2085]
              tunnel: w2047 -> [w2087]
              tunnel: [w2084] -> w2040 mode=indexing
              tunnel: [w2083] -> w2043
              tunnel: [w2070] -> w2038
              tunnel: w2042 -> [w2082]
              tunnel: w2018 -> [_] mode=indexing
              tunnel: w2041 -> [w2079]
              tunnel: w2018 -> [w2081]
              tunnel: w2037 -> [w2078]
              tunnel: w2036 -> [w2073]
              tunnel: w2035 -> [w2072]
              tunnel: [w2071] -> w2027 mode=indexing
              tunnel: [w2069] -> w2026 mode=indexing
              tunnel: w2017 -> [w2065]
              tunnel: w2016 -> [w2063]
              tunnel: w2015 -> [w2062]
              tunnel: w2014 -> [w2061]
              tunnel: [w2058] -> w2013 mode=indexing
              tunnel: w2011 -> [w2057]
              n746 = Dequeue Element(queue=w2087, timeout in ms (-1)=w2078) -> (element=w2067:T12, error out=w2068:errorcluster)  [unwired: 1 in, 2 out]
              n747 = Unbundle(w2066) -> ("gain"=w2083:dbl, "wfm"=w2086:i8[][], w2084:bool, "max queue size (-1, unlimited)"=w2060:i32)
              n748 = Index Array(array=w2079, index=w2060) -> (element=w2077:i32)
              n749 = Index Array(array=w2081, index (row)=w2060) -> (element=w2080:T20)  [unwired: 1 in]
              n750 = case shown="1" w2060 {
                tunnel: [w2096 w2097] -> w2074
                tunnel: w2073 -> [w2096 _]
                tunnel: w2072 -> [_ w2097]
                frame 0, Default {
                }
                frame 1 {
                }
              }
              n751 = Multiply(x=w2076, y=w2077) -> (x*y=w2075:i32)
              n752 = Reshape Array(w2086, w2085, w2075) -> (w2059:i8[][])
              n753 = for {
                N: w2077 -> [_]
                tunnel: w2080 -> [w2107]
                tunnel: [w2110] -> w2070
                tunnel: w2082 -> [w2109]
                shift-right: [w2103] -> _
                shift-left: w2059 -> [w2111]
                tunnel: w2074 -> [w2105] mode=indexing
                tunnel: w2076 -> [w2104]
                tunnel: [w2099] -> w2058 mode=indexing
                tunnel: w2057 -> [w2098]
                i -> [w2108]
                n754 = Index Array(array=w2107, index=w2108) -> (element=w2100:T17)
                n755 = Delete From Array(array=w2111, length=w2104, index (col)=0 ("disabled index (col)")) -> (deleted portion=w2102:i8[], array with subset deleted=w2103:i8[][])  [unwired: 1 in]
                n756 = call "TimeShiftDataSubMean.vi"("Filter"=w2098, "output cluster"=w2100, "Array In"=w2102) -> ("Array Out"=w2101:i16[][], "Sat Pts"=w2099:i32)  [unwired: 2 in]
                n757 = in-place {
                  in-place-border: w2101 -> [w2113]
                  in-place-border: w2105 -> [w2114]
                  n758 = in-place-dvr #13(w2109) -> (w2115:i16[][])  [unwired: 1 out]
                  n759 = case shown="0, Default" w2114 {
                    selector: w2114 -> [_ w2118]
                    tunnel: w2113 -> [w2117 w2120]
                    tunnel: [w2117 w2119] -> w2112
                    frame 0, Default {
                    }
                    frame 2 {
                      n760 = Multiply(x=w2118, y=w2120) -> (x*y=w2119:i16[][])
                    }
                  }
                  n761 = Add(x=w2112, y=w2115) -> (x+y=w2116:i16[][])
                  n762 = in-place-dvr #13(w2116) -> (w2110:refnum<data-value>)  [unwired: 1 out]
                }
              }
              n763 = Get Notifier Status(notifier=w2065) -> (current notification=w2064:bool)  [unwired: 1 in, 4 out]
              n764 = flat-sequence {
                tunnel: [w2095] -> w2071
                tunnel: w2068 -> [_]
                tunnel: w2067 -> [w2094]
                tunnel: [w2094] -> w2066
                frame #0 {
                  n765 = Tick Count (ms)() -> (millisecond timer value=w2095:u32)
                }
              }
              n766 = case shown="True" w2064 {
                tunnel: w2060 -> [_ w2092]
                tunnel: w2059 -> [_ w2091]
                tunnel: w2063 -> [_ w2090]
                tunnel: w2061 -> [_ w2089]
                tunnel: w2062 -> [_ w2088]
                frame False {
                }
                frame True {
                  n767 = call "RawRT_Capture.vi"("Raw data"=w2091, "File Name In"=w2090, "DigCard"=w2092, "header"=w2089, "Iter"=w2088) -> ()  [unwired: 7 in]
                }
              }
              n768 = flat-sequence {
                tunnel: [w2093] -> w2069
                tunnel: w2070 -> [_]
                frame #0 {
                  n769 = Tick Count (ms)() -> (millisecond timer value=w2093:u32)
                }
              }
            }
            n770 = Wait on Notification(notifier=w2033, timeout in ms (-1)=5) -> (timed out?=w2032:bool)  [unwired: 2 in, 3 out]
            n771 = Add Array Elements(numeric array=w2013) -> (sum=w2012:i32)
            n772 = Or Array Elements(Boolean array=w2040) -> (logical OR=w2039:bool)
            n773 = in-place {
              in-place-border: w2044 -> [w2056]
              in-place-border: w2039 -> [w2055]
              in-place-border: w2043 -> [w2054]
              in-place-border: w2012 -> [w2049]
              n774 = in-place-dvr #14(w2038) -> (w2050:i16[][])  [unwired: 1 out]
              n775 = Bundle("gain"=w2054, w2055, w2050, "Sat Pts"=w2049) -> (w2053:T21)  [unwired: 1 in]
              n776 = Multiply(x=i16 0, y=w2050) -> (x*y=w2052:i16[][])
              n777 = Lossy Enqueue Element(queue=w2056, element=w2053) -> ()  [unwired: 1 in, 4 out]
              n778 = in-place-dvr #14(w2052) -> (w2029:refnum<data-value>)  [unwired: 1 out]
            }
            n779 = Subtract(x=w2026, y=w2027) -> (x-y=w2028:u32[])
            n780 = Index Array(array=w2026, index=1) -> (element=w2030:u32)
            n781 = Not(x=w2032) -> (.not. x?=w2031:bool)
            n782 = Add Array Elements(numeric array=w2028) -> (sum=w2024:u32)
            n783 = Subtract(x=w2022, y=w2030) -> (x-y=w2023:u32)
            n784 = flat-sequence {
              tunnel: [w2048] -> w2022
              tunnel: w2029 -> [_]
              frame #0 {
                n785 = Tick Count (ms)() -> (millisecond timer value=w2048:u32)
              }
            }
            n786 = Add(x=w2023, y=w2024) -> (x+y=w2019:u32)
            n787 = call <vilib>:"Mean PtByPt.vi"("x"=w2019, "sample length"=20) -> ("mean"=w2020:dbl)  [unwired: 2 in, 1 out]
            n788 = local write "SF Loop"(w2020) -> ()
          }
          n789 = while {
            tunnel: w1988 -> [w2140]
            tunnel: w2010 -> [w2139]
            tunnel: w1971 -> [w2126]
            tunnel: w1991 -> [w2138]
            tunnel: [w2137] -> w2005
            tunnel: w2004 -> [w2136]
            shift-right: [w2124] -> _
            shift-left: _ -> [w2135]
            tunnel: [w2122] -> _
            tunnel: "0,1" -> [w2134]
            tunnel: w1987 -> [w2133]
            tunnel: w1982 -> [w2131]
            tunnel: w1975 -> [w2128]
            tunnel: [w2126] -> w1968
            tunnel: w1967 -> [w2121]
            stop <- w2130 stop-if-true
            n790 = for {
              tunnel: w2138 -> [w2155]
              tunnel: w2140 -> [w2157] mode=indexing
              tunnel: w2134 -> [w2156]
              tunnel: w2139 -> [w2154]
              tunnel: w2126 -> [w2151]
              tunnel: [w2149] -> w2137
              tunnel: w2136 -> [w2147]
              tunnel: w2133 -> [w2148]
              tunnel: w2128 -> [w2146]
              tunnel: [w2143] -> w2127
              tunnel: w2121 -> [w2142]
              i -> [w2145]
              # "Read data"
              n791 = case shown="0" w2145 {
                tunnel: w2157 -> [w2165 w2174]
                tunnel: w2156 -> [w2163 _]
                tunnel: w2155 -> [w2166 w2177]
                tunnel: [w2167 w2176] -> w2153
                tunnel: [w2160 w2173] -> w2152
                tunnel: w2151 -> [w2168 _]
                tunnel: [w2164 _] -> w2150
                tunnel: w2147 -> [w2162 _]
                tunnel: w2148 -> [_ w2171]
                tunnel: w2146 -> [w2159 _]
                tunnel: w2142 -> [w2158 w2169]
                frame 0 {
                  # "Read files and queue it up."
                  n792 = call <instrlib>:"niScope Initiate Acquisition.vi"("instrument handle"=w2168) -> ("error out"=w2161:errorcluster)  [unwired: 2 in, 12 out]
                  n793 = call "Rapid Read_NI.vi"("NI Card"=w2165, "Channel"=w2163, "Motion Board ID"=w2162, "rf points per line"=w2166, "error in"=w2161, "timeout"=w2158, "Pause?"=w2159) -> ("dig gain"=w2167:dbl, "Array"=w2160:i8[][], "Reverse?"=w2164:bool)  [unwired: 5 in, 1 out]
                }
                frame 1, Default {
                  n794 = property class="niScope"(reference=w2174, "Fetch Record Number"=0, "Fetch Number of Records"=w2171) -> (reference out=w2178:refnum<k15>, error out=w2175:errorcluster)  [unwired: 1 in]
                  n795 = call-poly <instrlib>:"niScope Fetch (poly).vi"("timeout"=w2169, "error in"=w2175, "numSamples"=w2177, "channels"="0", "instrument handle"=w2178) -> ("wfm"=w2173:i8[][], "wfm info"=w2180:T22)  [unwired: 5 out]
                  n796 = Index Array(array=w2180) -> (element=w2179:T23)  [unwired: 1 in]
                  n797 = Unbundle By Name(w2179) -> ("gain"=w2176:dbl)
                }
              }
              n798 = Bundle("gain"=w2153, "wfm"=w2152, "Reverse?"=w2150, w2145) -> (w2144:T24)  [unwired: 1 in]
              n799 = Enqueue Element(queue=w2154, element=w2144) -> (queue out=w2149:refnum<queue>, error out=w2143:errorcluster)  [unwired: 2 in, 1 out]
            }
            n800 = Wait on Notification(notifier=w2131, timeout in ms (-1)=5) -> (timed out?=w2129:bool)  [unwired: 2 in, 3 out]
            n801 = flat-sequence {
              tunnel: [w2141] -> w2124
              tunnel: w2127 -> [_]
              frame #0 {
                n802 = Tick Count (ms)() -> (millisecond timer value=w2141:u32)
              }
            }
            n803 = Not(x=w2129) -> (.not. x?=w2130:bool)
            n804 = Subtract(x=w2124, y=w2135) -> (x-y=w2122:u32)
            n805 = call <vilib>:"Mean PtByPt.vi"("x"=w2122, "sample length"=20) -> ("mean"=w2123:dbl)  [unwired: 2 in, 1 out]
            n806 = local write "Read Loop"(w2123) -> ()
          }
          n807 = property class="niScope"(reference=w1968, "Active Channel"="1", "Channel Enabled"=TRUE ("Vertical:Channel Enabled")) -> ()  [unwired: 1 in, 2 out]
          n808 = Release Queue(queue=w2005, force destroy? (F)=w1977) -> ()  [unwired: 1 in, 3 out]
          n809 = Delete Data Value Reference(data value reference=w1990) -> ()  [unwired: 1 in, 2 out]
        }
        frame "Drop Ch 5,4,3" {
          w2213 = 5
          # "Reduced data case that drop ring3,4,5 receive"
          # "Restructure file names"
          # "Read queue and send to files. About same as reading channel by channel"
          n810 = Array To Cluster(array=w2194) -> (cluster=w2195:cluster{"[0]":void, "[1]":void, "[2]":void})
          n811 = Reshape Array(w2214, w2213, w2213) -> (w2201:T19)
          n812 = Unbundle(w2195) -> ("[0]"=w2193)  [unwired: 2 out]
          n813 = expression code="x*5"(w2209) -> (w2204:dbl)
          n814 = Array Subset(array=w2201, length (col)=2 ("index")) -> (w2205:T19)  [unwired: 3 in]
          n815 = Obtain Queue(max queue size (-1, unlimited)=1, element data type=cluster{"gain":dbl, "wfm":i8[][], bool} {"gain"=0.0, "wfm"=[], TRUE}) -> (queue out=w2216:refnum<queue>)  [unwired: 3 in, 2 out]
          n816 = call "RTHeader.vi"("Comment"="Drop 3,4,5", "Votage scaling"=w2182) -> ("Header String Out"=w2184:string)  [unwired: 4 in, 1 out]
          n817 = Reshape Array(w2205, 10) -> (w2202:T20)
          n818 = while {
            tunnel: w2216 -> [w2255]
            tunnel: w2200 -> [w2254]
            tunnel: w2209 -> [w2253]
            tunnel: w2196 -> [w2250]
            tunnel: w2198 -> [w2252]
            tunnel: w2202 -> [w2242]
            tunnel: w2189 -> [w2248]
            tunnel: i16[] [1, 1, 1, 1, 2, 2, 2, 2, 2, 2] -> [w2247]
            tunnel: 10 -> [w2243]
            tunnel: [w2235] -> w2199
            tunnel: w2192 -> [w2239]
            tunnel: [w2237] -> w2191
            tunnel: w2185 -> [w2226]
            tunnel: w2184 -> [w2225]
            tunnel: w2183 -> [w2224]
            tunnel: w2181 -> [w2218]
            i -> [w2223]
            stop <- w2240 stop-if-true
            n819 = Dequeue Element(queue=w2255, timeout in ms (-1)=w2248) -> (queue out=w2237:refnum<queue>, element=w2229:cluster{"gain":dbl, "wfm":i8[][], bool}, error out=w2233:errorcluster)  [unwired: 1 in, 1 out]
            n820 = Unbundle(w2228) -> ("gain"=w2251:dbl, "wfm"=w2246:i8[][], w2244:bool)
            n821 = Multiply(x=w2254, y=w2243) -> (x*y=w2245:i32)
            n822 = flat-sequence {
              tunnel: [w2263] -> w2236
              tunnel: w2233 -> [_]
              tunnel: w2229 -> [w2262]
              tunnel: [w2262] -> w2228
              frame #0 {
                n823 = Tick Count (ms)() -> (millisecond timer value=w2263:u32)
              }
            }
            n824 = Reshape Array(w2246, w2253, w2245) -> (w2222:i8[][])
            n825 = for {
              N: w2243 -> [_]
              tunnel: w2242 -> [w2273]
              tunnel: [w2276] -> w2249
              tunnel: w2250 -> [w2275]
              shift-right: [w2271] -> _
              shift-left: w2222 -> [w2277]
              tunnel: w2254 -> [w2270]
              tunnel: w2247 -> [w2269] mode=indexing
              tunnel: [w2265] -> w2220 mode=indexing
              tunnel: w2218 -> [w2264]
              i -> [w2274]
              n826 = Index Array(array=w2273, index=w2274) -> (element=w2266:T17)
              n827 = Delete From Array(array=w2277, length=w2270, index (col)=0 ("disabled index (col)")) -> (deleted portion=w2268:i8[], array with subset deleted=w2271:i8[][])  [unwired: 1 in]
              n828 = call "TimeShiftDataSubMean.vi"("Filter"=w2264, "output cluster"=w2266, "Array In"=w2268) -> ("Array Out"=w2267:i16[][], "Sat Pts"=w2265:i32)  [unwired: 2 in]
              n829 = in-place {
                in-place-border: w2267 -> [w2279]
                in-place-border: w2269 -> [w2280]
                n830 = in-place-dvr #15(w2275) -> (w2281:i16[][])  [unwired: 1 out]
                n831 = case shown="0, Default" w2280 {
                  selector: w2280 -> [_ w2284]
                  tunnel: w2279 -> [w2283 w2286]
                  tunnel: [w2283 w2285] -> w2278
                  frame 0, Default {
                  }
                  frame 2 {
                    n832 = Multiply(x=w2284, y=w2286) -> (x*y=w2285:i16[][])
                  }
                }
                n833 = Add(x=w2278, y=w2281) -> (x+y=w2282:i16[][])
                n834 = in-place-dvr #15(w2282) -> (w2276:refnum<data-value>)  [unwired: 1 out]
              }
            }
            n835 = Get Notifier Status(notifier=w2226) -> (current notification=w2227:bool)  [unwired: 1 in, 4 out]
            n836 = case shown="True" w2227 {
              tunnel: 0 -> [_ w2260]
              tunnel: w2222 -> [_ w2259]
              tunnel: w2224 -> [_ w2258]
              tunnel: w2225 -> [_ w2257]
              tunnel: w2223 -> [_ w2256]
              frame False {
              }
              frame True {
                n837 = call "RawRT_Capture.vi"("Raw data"=w2259, "File Name In"=w2258, "DigCard"=w2260, "header"=w2257, "Iter"=w2256) -> ()  [unwired: 7 in]
              }
            }
            n838 = Add Array Elements(numeric array=w2220) -> (sum=w2219:i32)
            n839 = in-place {
              in-place-border: w2252 -> [w2294]
              in-place-border: w2244 -> [w2293]
              in-place-border: w2251 -> [w2292]
              in-place-border: w2219 -> [w2287]
              n840 = in-place-dvr #16(w2249) -> (w2288:i16[][])  [unwired: 1 out]
              n841 = Bundle("gain"=w2292, w2293, w2288, "Sat Pts"=w2287) -> (w2291:T21)  [unwired: 1 in]
              n842 = Multiply(x=i16 0, y=w2288) -> (x*y=w2290:i16[][])
              n843 = Lossy Enqueue Element(queue=w2294, element=w2291) -> ()  [unwired: 1 in, 4 out]
              n844 = in-place-dvr #16(w2290) -> (w2235:refnum<data-value>)  [unwired: 1 out]
            }
            n845 = Wait on Notification(notifier=w2239, timeout in ms (-1)=5) -> (timed out?=w2238:bool)  [unwired: 2 in, 3 out]
            n846 = Not(x=w2238) -> (.not. x?=w2240:bool)
            n847 = Subtract(x=w2234, y=w2236) -> (x-y=w2231:u32)
            n848 = flat-sequence {
              tunnel: [w2261] -> w2234
              tunnel: w2235 -> [_]
              frame #0 {
                n849 = Tick Count (ms)() -> (millisecond timer value=w2261:u32)
              }
            }
            n850 = call <vilib>:"Mean PtByPt.vi"("x"=w2231, "sample length"=20) -> ("mean"=w2230:dbl)  [unwired: 2 in, 1 out]
            n851 = local write "SF Loop"(w2230) -> ()
          }
          n852 = while {
            tunnel: w2193 -> [w2315]
            tunnel: w2216 -> [w2314]
            tunnel: w2204 -> [_]
            tunnel: w2200 -> [w2313]
            tunnel: w2211 -> [w2302]
            shift-right: [w2299] -> _
            shift-left: _ -> [w2312]
            tunnel: [w2297] -> _
            tunnel: "0,1" -> [w2311]
            tunnel: w2192 -> [w2305]
            tunnel: [w2304] -> w2197
            tunnel: w2190 -> [_]
            tunnel: w2188 -> [w2301]
            tunnel: w2187 -> [w2295]
            stop <- w2304 stop-if-true
            # "Read files and queue it up."
            # "Read data"
            n853 = call "Rapid Read_NI.vi"("NI Card"=w2315, "Channel"=w2311, "Motion Board ID"=w2302, "rf points per line"=w2313, "timeout"=w2295, "Pause?"=w2301) -> ("dig gain"=w2310:dbl, "Array"=w2309:i8[][], "Reverse?"=w2307:bool)  [unwired: 6 in, 1 out]
            n854 = Bundle("dig gain"=w2310, "Array"=w2309, "Reverse?"=w2307) -> (w2308:T26)  [unwired: 1 in]
            n855 = Enqueue Element(queue=w2314, element=w2308) -> (error out=w2300:errorcluster)  [unwired: 2 in, 2 out]
            n856 = stacked-sequence {
              tunnel: w2300 -> [_]
              tunnel: [w2316] -> w2299
              frame #0 {
                n857 = Tick Count (ms)() -> (millisecond timer value=w2316:u32)
              }
            }
            n858 = Wait on Notification(notifier=w2305, timeout in ms (-1)=5) -> (timed out?=w2303:bool)  [unwired: 2 in, 3 out]
            n859 = Not(x=w2303) -> (.not. x?=w2304:bool)
            n860 = Subtract(x=w2299, y=w2312) -> (x-y=w2297:u32)
            n861 = call <vilib>:"Mean PtByPt.vi"("x"=w2297, "sample length"=20) -> ("mean"=w2296:dbl)  [unwired: 2 in, 1 out]
            n862 = local write "Read Loop"(w2296) -> ()
          }
          n863 = Release Queue(queue=w2191, force destroy? (F)=w2197) -> ()  [unwired: 1 in, 3 out]
          n864 = Delete Data Value Reference(data value reference=w2199) -> ()  [unwired: 1 in, 2 out]
        }
        frame "Drop Ch 5,4,3,2" {
          w2354 = 5
          # "Reduced data case that drop ring3,4,5 receive"
          # "Restructure file names"
          # "Read queue and send to files. About same as reading channel by channel"
          n865 = Array To Cluster(array=w2336) -> (cluster=w2337:cluster{"[0]":void, "[1]":void, "[2]":void})
          n866 = Reshape Array(w2355, w2354, w2354) -> (w2343:T19)
          n867 = Unbundle(w2337) -> ("[0]"=w2330)  [unwired: 2 out]
          n868 = call "RTHeader.vi"("Comment"="Drop 2,3,4,5", "Votage scaling"=w2318) -> ("Header String Out"=w2319:string)  [unwired: 4 in, 1 out]
          n869 = property class="niScope"(reference=w2330, "Active Channel"="1", "Channel Enabled"=FALSE ("Vertical:Channel Enabled")) -> (reference out=w2327:refnum<k15>)  [unwired: 1 in, 1 out]
          n870 = Array Subset(array=w2343, length (col)=1 ("index")) -> (w2346:T19)  [unwired: 3 in]
          n871 = Obtain Queue(max queue size (-1, unlimited)=1, element data type=cluster{"gain":dbl, "wfm":i8[][], bool} {"gain"=0.0, "wfm"=[], TRUE}) -> (queue out=w2357:refnum<queue>)  [unwired: 3 in, 2 out]
          n872 = Reshape Array(w2346, 5) -> (w2344:T20)
          n873 = while {
            tunnel: w2357 -> [w2396]
            tunnel: w2342 -> [w2395]
            tunnel: w2350 -> [w2394]
            tunnel: w2338 -> [w2391]
            tunnel: w2340 -> [w2393]
            tunnel: w2344 -> [w2383]
            tunnel: w2331 -> [w2389]
            tunnel: i32[] [1, 2, 2, 2, 2] -> [w2388]
            tunnel: 5 -> [w2384]
            tunnel: [w2376] -> w2341
            tunnel: w2335 -> [w2380]
            tunnel: [w2378] -> w2334
            tunnel: w2322 -> [w2367]
            tunnel: w2321 -> [w2366]
            tunnel: w2319 -> [w2362]
            tunnel: w2317 -> [w2359]
            i -> [w2364]
            stop <- w2381 stop-if-true
            n874 = Dequeue Element(queue=w2396, timeout in ms (-1)=w2389) -> (queue out=w2378:refnum<queue>, element=w2370:cluster{"gain":dbl, "wfm":i8[][], bool}, error out=w2374:errorcluster)  [unwired: 1 in, 1 out]
            n875 = Unbundle(w2369) -> ("gain"=w2392:dbl, "wfm"=w2387:i8[][], w2385:bool)
            n876 = flat-sequence {
              tunnel: [w2404] -> w2377
              tunnel: w2374 -> [_]
              tunnel: w2370 -> [w2403]
              tunnel: [w2403] -> w2369
              frame #0 {
                n877 = Tick Count (ms)() -> (millisecond timer value=w2404:u32)
              }
            }
            n878 = Multiply(x=w2395, y=w2384) -> (x*y=w2386:i32)
            n879 = Reshape Array(w2387, w2394, w2386) -> (w2365:i8[][])
            n880 = for {
              N: w2384 -> [_]
              tunnel: w2383 -> [w2414]
              tunnel: [w2417] -> w2390
              tunnel: w2391 -> [w2416]
              shift-right: [w2412] -> _
              shift-left: w2365 -> [w2418]
              tunnel: w2395 -> [w2411]
              tunnel: w2388 -> [w2410] mode=indexing
              tunnel: [w2406] -> w2361 mode=indexing
              tunnel: w2359 -> [w2405]
              i -> [w2415]
              n881 = Index Array(array=w2414, index=w2415) -> (element=w2407:T17)
              n882 = Delete From Array(array=w2418, length=w2411, index (col)=0 ("disabled index (col)")) -> (deleted portion=w2409:i8[], array with subset deleted=w2412:i8[][])  [unwired: 1 in]
              n883 = call "TimeShiftDataSubMean.vi"("Filter"=w2405, "output cluster"=w2407, "Array In"=w2409) -> ("Array Out"=w2408:i16[][], "Sat Pts"=w2406:i32)  [unwired: 2 in]
              n884 = in-place {
                in-place-border: w2408 -> [w2420]
                in-place-border: w2410 -> [w2421]
                n885 = in-place-dvr #17(w2416) -> (w2422:i16[][])  [unwired: 1 out]
                n886 = case shown="0, Default" w2421 {
                  selector: w2421 -> [_ w2425]
                  tunnel: w2420 -> [w2424 w2427]
                  tunnel: [w2424 w2426] -> w2419
                  frame 0, Default {
                  }
                  frame 2 {
                    n887 = Multiply(x=w2425, y=w2427) -> (x*y=w2426:i32[][])
                  }
                }
                n888 = Add(x=w2419, y=w2422) -> (x+y=w2423:i32[][])
                n889 = in-place-dvr #17(w2423) -> (w2417:refnum<data-value>)  [unwired: 1 out]
              }
            }
            n890 = Get Notifier Status(notifier=w2367) -> (current notification=w2368:bool)  [unwired: 1 in, 4 out]
            n891 = case shown="True" w2368 {
              tunnel: 0 ("max queue size (-1, unlimited)") -> [_ w2401]
              tunnel: w2365 -> [_ w2400]
              tunnel: w2366 -> [_ w2399]
              tunnel: w2362 -> [_ w2398]
              tunnel: w2364 -> [_ w2397]
              frame False {
              }
              frame True {
                n892 = call "RawRT_Capture.vi"("Raw data"=w2400, "File Name In"=w2399, "DigCard"=w2401, "header"=w2398, "Iter"=w2397) -> ()  [unwired: 7 in]
              }
            }
            n893 = Wait on Notification(notifier=w2380, timeout in ms (-1)=5) -> (timed out?=w2379:bool)  [unwired: 2 in, 3 out]
            n894 = Add Array Elements(numeric array=w2361) -> (sum=w2360:i32)
            n895 = in-place {
              in-place-border: w2393 -> [w2435]
              in-place-border: w2385 -> [w2434]
              in-place-border: w2392 -> [w2433]
              in-place-border: w2360 -> [w2428]
              n896 = in-place-dvr #18(w2390) -> (w2429:i16[][])  [unwired: 1 out]
              n897 = Bundle("gain"=w2433, w2434, w2429, "Sat Pts"=w2428) -> (w2432:T21)  [unwired: 1 in]
              n898 = Multiply(x=i16 0, y=w2429) -> (x*y=w2431:i16[][])
              n899 = Lossy Enqueue Element(queue=w2435, element=w2432) -> ()  [unwired: 1 in, 4 out]
              n900 = in-place-dvr #18(w2431) -> (w2376:refnum<data-value>)  [unwired: 1 out]
            }
            n901 = Not(x=w2379) -> (.not. x?=w2381:bool)
            n902 = Subtract(x=w2375, y=w2377) -> (x-y=w2372:u32)
            n903 = flat-sequence {
              tunnel: [w2402] -> w2375
              tunnel: w2376 -> [_]
              frame #0 {
                n904 = Tick Count (ms)() -> (millisecond timer value=w2402:u32)
              }
            }
            n905 = call <vilib>:"Mean PtByPt.vi"("x"=w2372, "sample length"=20) -> ("mean"=w2371:dbl)  [unwired: 2 in, 1 out]
            n906 = local write "SF Loop"(w2371) -> ()
          }
          n907 = while {
            tunnel: w2327 -> [w2440]
            tunnel: w2357 -> [w2456]
            tunnel: w2342 -> [w2455]
            tunnel: w2352 -> [w2444]
            shift-right: [w2441] -> _
            shift-left: _ -> [w2454]
            tunnel: [w2438] -> _
            tunnel: "0" -> [w2453]
            tunnel: w2335 -> [w2447]
            tunnel: [w2446] -> w2339
            tunnel: w2333 -> [w2443]
            tunnel: w2332 -> [_]
            tunnel: [w2440] -> w2324
            tunnel: w2323 -> [w2436]
            stop <- w2446 stop-if-true
            # "Read files and queue it up."
            # "Read data"
            n908 = call "Rapid Read_NI.vi"("NI Card"=w2440, "Channel"=w2453, "Motion Board ID"=w2444, "rf points per line"=w2455, "timeout"=w2436, "Pause?"=w2443) -> ("dig gain"=w2452:dbl, "Array"=w2451:i8[][], "Reverse?"=w2449:bool)  [unwired: 6 in, 1 out]
            n909 = Bundle("dig gain"=w2452, "Array"=w2451, "Reverse?"=w2449) -> (w2450:T26)  [unwired: 1 in]
            n910 = Enqueue Element(queue=w2456, element=w2450) -> (error out=w2442:errorcluster)  [unwired: 2 in, 2 out]
            n911 = stacked-sequence {
              tunnel: w2442 -> [_]
              tunnel: [w2457] -> w2441
              frame #0 {
                n912 = Tick Count (ms)() -> (millisecond timer value=w2457:u32)
              }
            }
            n913 = Wait on Notification(notifier=w2447, timeout in ms (-1)=5) -> (timed out?=w2445:bool)  [unwired: 2 in, 3 out]
            n914 = Not(x=w2445) -> (.not. x?=w2446:bool)
            n915 = Subtract(x=w2441, y=w2454) -> (x-y=w2438:u32)
            n916 = call <vilib>:"Mean PtByPt.vi"("x"=w2438, "sample length"=20) -> ("mean"=w2437:dbl)  [unwired: 2 in, 1 out]
            n917 = local write "Read Loop"(w2437) -> ()
          }
          n918 = property class="niScope"(reference=w2324, "Active Channel"="1", "Channel Enabled"=TRUE ("Vertical:Channel Enabled")) -> ()  [unwired: 1 in, 2 out]
          n919 = Release Queue(queue=w2334, force destroy? (F)=w2339) -> ()  [unwired: 1 in, 3 out]
          n920 = Delete Data Value Reference(data value reference=w2341) -> ()  [unwired: 1 in, 2 out]
        }
        frame "All 25 FIFO CH by CH" {
          w2481 = 5
          w2476 = "1"
          # "Read queue and send to files."
          n921 = Array To Cluster(array=w2466) -> (cluster=w2467:cluster{"[0]":void, "[1]":void, "[2]":void})
          n922 = Unbundle(w2467) -> ("[0]"=w2465, "[1]"=w2464, "[2]"=w2463)
          n923 = expression code="x*5"(w2478) -> (w2483:dbl)
          n924 = Reshape Array(w2482, w2481, w2481) -> (w2480:T19)
          n925 = Obtain Queue(max queue size (-1, unlimited)=3, element data type=T12 {"gain"=0.0, "wfm"=[], TRUE, "max queue size (-1, unlimited)"=25}) -> (queue out=w2487:refnum<queue>)  [unwired: 3 in, 2 out]
          n926 = Build Array(w2465, w2465, w2464, w2464, w2463) -> (w2490:void[])
          n927 = expression code="x*5"(w2475) -> (w2485:dbl)
          n928 = Build Array("0", w2476, "0", w2476, w2476) -> (w2489:string[])
          n929 = while {
            tunnel: w2490 -> [w2580]
            tunnel: w2489 -> [w2579]
            tunnel: w2487 -> [w2578]
            tunnel: w2464 -> [w2577]
            tunnel: w2463 -> [w2576]
            tunnel: w2483 -> [w2575]
            tunnel: w2475 -> [w2574]
            tunnel: w2477 -> [w2567]
            shift-right: [w2572] -> _
            shift-left: _ -> [w2573]
            tunnel: [w2563] -> _
            tunnel: w2471 -> [w2570]
            tunnel: [w2570] -> w2470
            tunnel: [w2569] -> w2469
            tunnel: w2460 -> [w2566]
            tunnel: w2459 -> [w2561]
            stop <- w2569 stop-if-true
            n930 = for {
              tunnel: w2574 -> [w2594]
              tunnel: w2575 -> [w2597]
              tunnel: w2580 -> [w2596] mode=indexing
              tunnel: w2579 -> [w2595] mode=indexing
              tunnel: w2578 -> [w2593]
              tunnel: w2577 -> [w2590]
              tunnel: w2576 -> [w2589]
              tunnel: w2567 -> [w2587]
              tunnel: w2566 -> [w2586]
              tunnel: [w2583] -> w2565
              tunnel: w2561 -> [w2582]
              i -> [w2584]
              # "Read data"
              n931 = case shown="0" w2584 {
                tunnel: w2597 -> [_ w2619]
                tunnel: w2596 -> [w2603 w2618]
                tunnel: w2595 -> [w2601 w2616]
                tunnel: w2594 -> [w2604 w2615]
                tunnel: [w2605 w2614] -> w2592
                tunnel: [w2606 w2613] -> w2591
                tunnel: w2590 -> [w2610 _]
                tunnel: w2589 -> [w2609 _]
                tunnel: [w2602 _] -> w2588
                tunnel: w2587 -> [w2600 _]
                tunnel: w2586 -> [w2599 _]
                tunnel: w2582 -> [w2598 _]
                frame 0 {
                  # "Read files and queue it up."
                  n932 = call <instrlib>:"niScope Initiate Acquisition.vi"("instrument handle"=w2610) -> ("error out"=w2608:errorcluster)  [unwired: 2 in, 12 out]
                  n933 = call <instrlib>:"niScope Initiate Acquisition.vi"("instrument handle"=w2609, "error in"=w2608) -> ("error out"=w2607:errorcluster)  [unwired: 1 in, 12 out]
                  n934 = call "Rapid Read_NI.vi"("NI Card"=w2603, "Channel"=w2601, "Motion Board ID"=w2600, "rf points per line"=w2604, "error in"=w2607, "timeout"=w2598, "Pause?"=w2599) -> ("dig gain"=w2605:dbl, "Array"=w2606:i8[][], "Reverse?"=w2602:bool)  [unwired: 5 in, 1 out]
                }
                frame 1, Default {
                  n935 = property class="niScope"(reference=w2618, "Fetch Record Number"=0, "Fetch Number of Records"=w2619) -> (reference out=w2617:refnum<k15>, error out=w2612:errorcluster)  [unwired: 1 in]
                  n936 = call-poly <instrlib>:"niScope Fetch (poly).vi"("timeout"=0.0, "error in"=w2612, "numSamples"=w2615, "channels"=w2616, "instrument handle"=w2617) -> ("wfm"=w2613:i8[][], "wfm info"=w2622:T22)  [unwired: 5 out]
                  n937 = Index Array(array=w2622) -> (element=w2621:T23)  [unwired: 1 in]
                  n938 = Unbundle By Name(w2621) -> ("gain"=w2614:dbl)
                }
              }
              n939 = Bundle("gain"=w2592, "wfm"=w2591, "Reverse?"=w2588, w2584) -> (w2585:T24)  [unwired: 1 in]
              n940 = Enqueue Element(queue=w2593, element=w2585) -> (error out=w2583:errorcluster)  [unwired: 2 in, 2 out]
            }
            n941 = flat-sequence {
              tunnel: [w2581] -> w2572
              tunnel: w2565 -> [_]
              frame #0 {
                n942 = Tick Count (ms)() -> (millisecond timer value=w2581:u32)
              }
            }
            n943 = Wait on Notification(notifier=w2570, timeout in ms (-1)=5) -> (timed out?=w2568:bool)  [unwired: 2 in, 3 out]
            n944 = Not(x=w2568) -> (.not. x?=w2569:bool)
            n945 = Subtract(x=w2572, y=w2573) -> (x-y=w2563:u32)
            n946 = call <vilib>:"Mean PtByPt.vi"("x"=w2563, "sample length"=20) -> ("mean"=w2562:dbl)  [unwired: 2 in, 1 out]
            n947 = local write "Read Loop"(w2562) -> ()
          }
          n948 = while {
            tunnel: w2487 -> [w2515]
            tunnel: w2485 -> [w2514]
            tunnel: w2480 -> [w2506]
            tunnel: w2478 -> [w2513]
            tunnel: w2468 -> [w2510]
            tunnel: w2472 -> [w2512]
            tunnel: w2475 -> [w2507]
            tunnel: [w2503] -> w2474
            tunnel: w2470 -> [w2501]
            tunnel: [w2498] -> w2462
            tunnel: w2461 -> [w2497]
            tunnel: w2458 -> [w2491]
            stop <- w2500 stop-if-true
            n949 = for {
              tunnel: w2514 -> [w2544]
              tunnel: w2513 -> [w2540]
              tunnel: w2515 -> [w2543]
              tunnel: w2506 -> [_] mode=indexing
              tunnel: [w2539] -> w2504 mode=indexing
              tunnel: [w2538] -> w2511
              tunnel: [w2537] -> w2509
              tunnel: w2510 -> [w2536]
              tunnel: w2507 -> [w2535]
              tunnel: w2506 -> [w2534]
              workers-P: _ -> [_]
              tunnel: [w2530] -> w2498
              tunnel: w2497 -> [w2531]
              tunnel: [w2529] -> w2495 mode=indexing
              tunnel: [w2525] -> w2493 mode=indexing
              tunnel: w2491 -> [w2524]
              n950 = Dequeue Element(queue=w2543, timeout in ms (-1)=w2531) -> (queue out=w2530:refnum<queue>, element=w2527:T12, error out=w2528:errorcluster)  [unwired: 1 in, 1 out]
              n951 = flat-sequence {
                tunnel: [w2546] -> w2529
                tunnel: w2528 -> [_]
                tunnel: w2527 -> [w2545]
                tunnel: [w2545] -> w2526
                frame #0 {
                  n952 = Tick Count (ms)() -> (millisecond timer value=w2546:u32)
                }
              }
              n953 = Unbundle(w2526) -> ("gain"=w2538:dbl, "wfm"=w2542:i8[][], w2539:bool, "max queue size (-1, unlimited)"=w2532:i32)
              n954 = Index Array(array=w2534, index (row)=w2532) -> (element=w2533:T20)  [unwired: 1 in]
              n955 = Reshape Array(w2542, w2540, w2544) -> (w2541:i8[][])
              n956 = for {
                tunnel: w2533 -> [w2549] mode=indexing
                tunnel: [w2556] -> w2537
                tunnel: w2536 -> [w2555]
                tunnel: w2535 -> [w2553]
                shift-right: [w2552] -> _
                shift-left: w2541 -> [w2557]
                tunnel: [w2548] -> w2525 mode=indexing
                tunnel: w2524 -> [w2547]
                n957 = Delete From Array(array=w2557, length=w2553, index (col)=0 ("disabled index (col)")) -> (deleted portion=w2551:i8[], array with subset deleted=w2552:i8[][])  [unwired: 1 in]
                n958 = call "TimeShiftDataSubMean.vi"("Filter"=w2547, "output cluster"=w2549, "Array In"=w2551) -> ("Array Out"=w2550:i16[][], "Sat Pts"=w2548:i32)  [unwired: 2 in]
                n959 = in-place {
                  in-place-border: w2550 -> [w2560]
                  n960 = in-place-dvr #19(w2555) -> (w2558:i16[][])  [unwired: 1 out]
                  n961 = Add(x=w2560, y=w2558) -> (x+y=w2559:i16[][])
                  n962 = in-place-dvr #19(w2559) -> (w2556:refnum<data-value>)  [unwired: 1 out]
                }
              }
            }
            n963 = Wait on Notification(notifier=w2501, timeout in ms (-1)=5) -> (timed out?=w2499:bool)  [unwired: 2 in, 3 out]
            n964 = Or Array Elements(Boolean array=w2504) -> (logical OR=w2505:bool)
            n965 = Index Array(array=w2495) -> (element=w2494:u32)  [unwired: 1 in]
            n966 = Add Array Elements(numeric array=w2493) -> (sum=w2492:i32)
            n967 = in-place {
              in-place-border: w2512 -> [w2523]
              in-place-border: w2505 -> [w2522]
              in-place-border: w2511 -> [w2521]
              in-place-border: w2492 -> [w2516]
              n968 = in-place-dvr #20(w2509) -> (w2517:i16[][])  [unwired: 1 out]
              n969 = Bundle("gain"=w2521, w2522, w2517, "Sat Pts"=w2516) -> (w2520:T21)  [unwired: 1 in]
              n970 = Multiply(x=i16 0, y=w2517) -> (x*y=w2519:i16[][])
              n971 = Lossy Enqueue Element(queue=w2523, element=w2520) -> ()  [unwired: 1 in, 4 out]
              n972 = in-place-dvr #20(w2519) -> (w2503:refnum<data-value>)  [unwired: 1 out]
            }
            n973 = Not(x=w2499) -> (.not. x?=w2500:bool)
            n974 = Tick Count (ms)() -> (millisecond timer value=w2508:u32)
            n975 = Subtract(x=w2508, y=w2494) -> (x-y=w2496:u32)
            n976 = local write "SF Loop"(w2496) -> ()
          }
          n977 = Delete Data Value Reference(data value reference=w2474) -> ()  [unwired: 1 in, 2 out]
          n978 = Release Queue(queue=w2462, force destroy? (F)=w2469) -> ()  [unwired: 1 in, 3 out]
        }
        frame "Line by line 2 Ch" {
          w2641 = 5
          # "Not fast enough for read"
          # "Read queue and send to files for chans 1,2"
          n979 = Array To Cluster(array=w2626) -> (cluster=w2627:cluster{"[0]":void, "[1]":void, "[2]":void})
          n980 = Reshape Array(w2636, w2641, w2641) -> (w2637:T19)
          n981 = Unbundle(w2627) -> ("[0]"=w2625)  [unwired: 2 out]
          n982 = Array Subset(array=w2637, length (col)=2 ("index")) -> (w2638:T19)  [unwired: 3 in]
          n983 = Obtain Queue(max queue size (-1, unlimited)=10, element data type=cluster{"gain":dbl, "wfm":i8[][], bool} {"gain"=0.0, "wfm"=[], TRUE}) -> (queue out=w2642:refnum<queue>)  [unwired: 3 in, 2 out]
          n984 = Reshape Array(w2638, 10) -> (w2635:T20)
          n985 = while {
            tunnel: w2642 -> [w2658]
            tunnel: w2635 -> [w2664]
            tunnel: w2628 -> [w2660]
            tunnel: w2631 -> [w2663]
            tunnel: [w2658] -> w2643
            tunnel: i16[] [1, 1, 1, 1, 2, 2, 2, 2, 2, 2] -> [w2657]
            tunnel: [w2656] -> w2632
            tunnel: w2630 -> [w2654]
            tunnel: w2623 -> [w2649]
            stop <- w2653 stop-if-true
            n986 = for {
              tunnel: w2658 -> [w2685]
              tunnel: w2664 -> [w2676] mode=indexing
              tunnel: [w2682] -> w2662
              tunnel: [w2681] -> w2661
              tunnel: [w2680] -> w2659
              tunnel: w2660 -> [w2679]
              tunnel: w2657 -> [w2678] mode=indexing
              tunnel: [w2674] -> w2651 mode=indexing
              tunnel: w2649 -> [w2673]
              n987 = Dequeue Element(queue=w2685, timeout in ms (-1)=1000) -> (element=w2684:cluster{"gain":dbl, "wfm":i8[][], bool})  [unwired: 1 in, 3 out]
              n988 = Unbundle(w2684) -> ("gain"=w2681:dbl, "wfm"=w2677:i8[][], w2682:bool)
              n989 = call "TimeShiftDataSubMean.vi"("Filter"=w2673, "output cluster"=w2676, "Array In"=w2677) -> ("Array Out"=w2675:i16[][], "Sat Pts"=w2674:i32)  [unwired: 2 in]
              n990 = in-place {
                in-place-border: w2675 -> [w2687]
                in-place-border: w2678 -> [w2688]
                n991 = in-place-dvr #21(w2679) -> (w2689:i16[][])  [unwired: 1 out]
                n992 = case shown="2" w2688 {
                  selector: w2688 -> [_ w2692]
                  tunnel: w2687 -> [w2691 w2694]
                  tunnel: [w2691 w2693] -> w2686
                  frame 0, Default {
                  }
                  frame 2 {
                    n993 = Multiply(x=w2692, y=w2694) -> (x*y=w2693:i16[][])
                  }
                }
                n994 = Add(x=w2686, y=w2689) -> (x+y=w2690:i16[][])
                n995 = in-place-dvr #21(w2690) -> (w2680:refnum<data-value>)  [unwired: 1 out]
              }
            }
            n996 = Wait on Notification(notifier=w2654, timeout in ms (-1)=5) -> (timed out?=w2652:bool)  [unwired: 2 in, 3 out]
            n997 = Add Array Elements(numeric array=w2651) -> (sum=w2650:i32)
            n998 = in-place {
              in-place-border: w2663 -> [w2672]
              in-place-border: w2662 -> [w2671]
              in-place-border: w2661 -> [w2670]
              in-place-border: w2650 -> [w2665]
              n999 = in-place-dvr #22(w2659) -> (w2666:i16[][])  [unwired: 1 out]
              n1000 = Bundle("gain"=w2670, w2671, w2666, "Sat Pts"=w2665) -> (w2669:T21)  [unwired: 1 in]
              n1001 = Multiply(x=i16 0, y=w2666) -> (x*y=w2668:i16[][])
              n1002 = Lossy Enqueue Element(queue=w2672, element=w2669) -> ()  [unwired: 1 in, 4 out]
              n1003 = in-place-dvr #22(w2668) -> (w2656:refnum<data-value>)  [unwired: 1 out]
            }
            n1004 = Not(x=w2652) -> (.not. x?=w2653:bool)
          }
          n1005 = while {
            tunnel: w2645 -> [w2708]
            tunnel: w2633 -> [w2707]
            tunnel: w2644 -> [w2697]
            tunnel: w2642 -> [w2706]
            shift-right: [w2704] -> _
            shift-left: _ -> [w2705]
            tunnel: [w2695] -> _
            tunnel: w2625 -> [w2703]
            tunnel: w2630 -> [w2701]
            tunnel: [w2700] -> w2629
            tunnel: w2624 -> [w2696]
            stop <- w2700 stop-if-true
            # "Read files and queue it up."
            # "Read data"
            n1006 = call "Rapid Read_2Ch.vi"("NI Card 3"=w2703, "Pause?"=w2696, "Motion Board ID"=w2697, "rf points per line"=w2707, "lines per plane"=w2708, "queue out"=w2706) -> ("error out"=w2698:errorcluster)  [unwired: 6 in, 3 out]
            n1007 = Wait on Notification(notifier=w2701, timeout in ms (-1)=5) -> (timed out?=w2699:bool)  [unwired: 2 in, 3 out]
            n1008 = flat-sequence {
              tunnel: w2698 -> [_]
              tunnel: [w2709] -> w2704
              frame #0 {
                n1009 = Tick Count (ms)() -> (millisecond timer value=w2709:u32)
              }
            }
            n1010 = Not(x=w2699) -> (.not. x?=w2700:bool)
            n1011 = Subtract(x=w2704, y=w2705) -> (x-y=w2695:u32)
            n1012 = local write "Read Loop"(w2695) -> ()
          }
          n1013 = Delete Data Value Reference(data value reference=w2632) -> ()  [unwired: 1 in, 2 out]
          n1014 = Release Queue(queue=w2643, force destroy? (F)=w2629) -> ()  [unwired: 1 in, 3 out]
        }
        frame "Line by line All" {
          # "Not fast enough for read"
          # "Read queue and send to files all 25"
          n1015 = Obtain Queue(max queue size (-1, unlimited)=25, element data type=T12 {"gain"=0.0, "wfm"=[], TRUE, "max queue size (-1, unlimited)"=1}) -> (queue out=w2718:refnum<queue>)  [unwired: 3 in, 2 out]
          n1016 = while {
            tunnel: w2718 -> [w2734]
            tunnel: w2722 -> [w2727]
            tunnel: w2712 -> [w2736]
            tunnel: [w2734] -> w2719
            tunnel: [w2733] -> w2717
            tunnel: w2716 -> [w2732]
            tunnel: w2715 -> [w2729]
            stop <- w2730 stop-if-true
            n1017 = for {
              tunnel: w2734 -> [w2758]
              tunnel: w2727 -> [_] mode=indexing
              tunnel: [w2755] -> w2738
              tunnel: [w2754] -> w2737
              tunnel: [w2753] -> w2735
              tunnel: w2736 -> [w2752]
              tunnel: w2727 -> [w2749]
              n1018 = Dequeue Element(queue=w2758, timeout in ms (-1)=500) -> (element=w2757:T12)  [unwired: 1 in, 3 out]
              n1019 = Unbundle(w2757) -> ("gain"=w2754:dbl, "wfm"=w2750:i8[][], w2755:bool, "max queue size (-1, unlimited)"=w2748:i32)
              n1020 = Index Array(array=w2749, index=w2748) -> (element=w2747:T17)
              n1021 = call-poly "TimeShiftDataPoly.vi"("output cluster"=w2747, "Array In"=w2750) -> ("Array Out"=w2751:i8[][])  [unwired: 1 in, 1 out]
              n1022 = in-place {
                in-place-border: w2751 -> [w2761]
                n1023 = in-place-dvr #23(w2752) -> (w2759:i16[][])  [unwired: 1 out]
                n1024 = Add(x=w2761, y=w2759) -> (x+y=w2760:i16[][])
                n1025 = in-place-dvr #23(w2760) -> (w2753:refnum<data-value>)  [unwired: 1 out]
              }
            }
            n1026 = Wait on Notification(notifier=w2729, timeout in ms (-1)=5) -> (timed out?=w2728:bool)  [unwired: 2 in, 3 out]
            n1027 = in-place {
              in-place-border: w2738 -> [w2746]
              in-place-border: w2737 -> [w2745]
              in-place-border: w2732 -> [w2740]
              in-place-border: 0 -> [w2739]
              n1028 = in-place-dvr #24(w2735) -> (w2741:i16[][])  [unwired: 1 out]
              n1029 = Bundle("gain"=w2745, w2746, w2741, w2739) -> (w2744:cluster{"gain":dbl, bool, i16[][], i32})  [unwired: 1 in]
              n1030 = Multiply(x=i16 0, y=w2741) -> (x*y=w2743:i16[][])
              n1031 = Lossy Enqueue Element(queue=w2740, element=w2744) -> ()  [unwired: 1 in, 4 out]
              n1032 = in-place-dvr #24(w2743) -> (w2733:refnum<data-value>)  [unwired: 1 out]
            }
            n1033 = Not(x=w2728) -> (.not. x?=w2730:bool)
          }
          n1034 = while {
            tunnel: w2721 -> [w2775]
            tunnel: w2713 -> [w2774]
            tunnel: w2711 -> [w2773]
            tunnel: w2720 -> [w2764]
            tunnel: w2718 -> [w2772]
            shift-right: [w2770] -> _
            shift-left: _ -> [w2771]
            tunnel: [w2762] -> _
            tunnel: w2715 -> [w2768]
            tunnel: [w2767] -> w2714
            tunnel: w2710 -> [w2763]
            stop <- w2767 stop-if-true
            # "Read files and queue it up."
            # "Read data"
            n1035 = call "Rapid Read_5Ch.vi"("Dig Cards"=w2773, "Pause?"=w2763, "Motion Board ID"=w2764, "rf points per line"=w2774, "lines per plane"=w2775, "queue out"=w2772) -> ("error out"=w2765:errorcluster)  [unwired: 6 in, 3 out]
            n1036 = flat-sequence {
              tunnel: w2765 -> [_]
              tunnel: [w2776] -> w2770
              frame #0 {
                n1037 = Tick Count (ms)() -> (millisecond timer value=w2776:u32)
              }
            }
            n1038 = Wait on Notification(notifier=w2768, timeout in ms (-1)=5) -> (timed out?=w2766:bool)  [unwired: 2 in, 3 out]
            n1039 = Not(x=w2766) -> (.not. x?=w2767:bool)
            n1040 = Subtract(x=w2770, y=w2771) -> (x-y=w2762:u32)
            n1041 = local write "Read Loop"(w2762) -> ()
          }
          n1042 = Release Queue(queue=w2719, force destroy? (F)=w2714) -> ()  [unwired: 1 in, 3 out]
          n1043 = Delete Data Value Reference(data value reference=w2717) -> ()  [unwired: 1 in, 2 out]
        }
        frame "Deep Memory 2 CH" {
          w2804 = 5
          # "Just Ch 1,2. Also cam suffer memory overflow if Byte depth too small"
          # "Arm digitizer"
          n1044 = Array To Cluster(array=w2779) -> (cluster=w2780:cluster{"[0]":void, "[1]":void, "[2]":void})
          n1045 = Unbundle(w2780) -> ("[0]"=w2778)  [unwired: 2 out]
          n1046 = Reshape Array(w2799, w2804, w2804) -> (w2800:T19)
          n1047 = call <instrlib>:"niScope Initiate Acquisition.vi"("instrument handle"=w2778) -> ("error out"=w2790:errorcluster)  [unwired: 2 in, 12 out]
          n1048 = expression code="x*5"(w2793) -> (w2805:dbl)
          n1049 = Array Subset(array=w2800, length (col)=2 ("index")) -> (w2801:T19)  [unwired: 3 in]
          n1050 = Obtain Queue(max queue size (-1, unlimited)=2, element data type=cluster{"Fetch:Records Done":i32, bool} {"Fetch:Records Done"=0, TRUE}) -> (queue out=w2788:refnum<queue>)  [unwired: 2 in, 3 out]
          n1051 = Obtain Queue(max queue size (-1, unlimited)=2, element data type=i8[][] [] ("Array")) -> (queue out=w2798:refnum<queue>)  [unwired: 2 in, 3 out]
          n1052 = node-c288(i64 50 ("Period")) -> (w2807:T13)
          n1053 = Reshape Array(w2801, 10) -> (w2797:T20)
          n1054 = while {
            tunnel: w2788 -> [w2937]
            tunnel: w2778 -> [w2945]
            tunnel: w2798 -> [w2946]
            tunnel: w2795 -> [w2938]
            tunnel: [w2933] -> w2810
            tunnel: w2790 -> [w2944]
            tunnel: w2805 -> [w2934]
            tunnel: [w2931] -> w2791
            shift-right: [w2930] -> _
            shift-left: _ -> [w2929]
            tunnel: [w2921] -> _
            tunnel: w2785 -> [w2926]
            tunnel: [w2925] -> w2783
            tunnel: w2777 -> [w2923]
            stop <- w2925 stop-if-true
            # "This loop reads the data once it is in the queue"
            # "Get and display data"
            n1055 = Dequeue Element(queue=w2937, timeout in ms (-1)=w2923, error in (no error)=w2944) -> (queue out=w2936:refnum<queue>, element=w2947:cluster{"Fetch:Records Done":i32, bool}, error out=w2940:errorcluster)  [unwired: 1 out]
            n1056 = Unbundle(w2947) -> ("Fetch:Records Done"=w2942:i32)  [unwired: 1 out]
            n1057 = property class="niScope"(reference=w2945, error in=w2940, "Fetch Record Number"=w2942, "Fetch Number of Records"=w2934) -> (reference out=w2939:refnum<k15>, error out=w2941:errorcluster)
            n1058 = call-poly <instrlib>:"niScope Fetch (poly).vi"("timeout"=1.0, "error in"=w2941, "numSamples"=w2938, "channels"="0,1", "instrument handle"=w2939) -> ("error out"=w2928:errorcluster, "wfm"=w2943:i8[][], "instrument handle out"=w2931:refnum<k15>)  [unwired: 4 out]
            n1059 = case shown="No Error" w2928 {
              selector: w2928 -> [_ w2956]
              tunnel: w2946 -> [w2955 w2957]
              tunnel: w2943 -> [w2954 _]
              tunnel: w2936 -> [w2953 _]
              tunnel: [w2952 w2957] -> w2933
              tunnel: [w2949 w2956] -> w2922
              frame No Error {
                n1060 = Lossy Enqueue Element(queue=w2955, element=w2954) -> (queue out=w2952:refnum<queue>, error out=w2951:errorcluster)  [unwired: 1 in, 2 out]
                n1061 = Get Queue Status(queue=w2953, error in (no error)=w2951) -> (error out=w2949:errorcluster, # elements in queue=w2950:i32)  [unwired: 1 in, 6 out]
                n1062 = local write "SF queue"(w2950) -> ()
              }
              frame Error {
              }
            }
            n1063 = stacked-sequence {
              tunnel: [w2948] -> w2930
              tunnel: w2922 -> [_]
              frame #0 {
                n1064 = Tick Count (ms)() -> (millisecond timer value=w2948:u32)
              }
            }
            n1065 = Wait on Notification(notifier=w2926, timeout in ms (-1)=5) -> (timed out?=w2924:bool)  [unwired: 2 in, 3 out]
            n1066 = Not(x=w2924) -> (.not. x?=w2925:bool)
            n1067 = Subtract(x=w2930, y=w2929) -> (x-y=w2921:u32)
            n1068 = local write "Read Loop"(w2921) -> ()
          }
          n1069 = timed-loop {
            shift-right: [w2890] -> _
            shift-left: 0 -> [w2896]
            shift-right: [w2902] -> _
            shift-left: TRUE -> [w2897]
            tunnel: w2814 -> [w2900]
            tunnel: [w2886] -> w2811
            tunnel: w2778 -> [w2895]
            tunnel: w2808 -> [w2891]
            tunnel: w2790 -> [w2899]
            timing: w2807 -> [_]
            timing-out: [_] -> w2806
            tunnel: w2788 -> [w2884]
            tunnel: w2785 -> [w2881]
            stop <- w2880 stop-if-true
            # "This loop performs back and forth scan and records record # at end of run"
            n1070 = Bundle(w2896, w2897) -> (w2894:cluster{i32, bool})  [unwired: 1 in]
            n1071 = Select(t=T11 6 ("Program (1)"), s=w2897, f=T11 7 ("Program (1)")) -> (s? t:f=w2885:T11)
            n1072 = call <vilib>:"Run Program.flx"("error in (no error)"=w2899, "Program (1)"=w2885, "Board ID"=w2900) -> ("error out"=w2893:errorcluster, "Bd ID Out"=w2888:T5)  [unwired: 4 out]
            n1073 = stacked-sequence {
              tunnel: w2893 -> [w2914]
              tunnel: [w2914] -> w2892
              tunnel: [w2912] -> w2889
              tunnel: w2888 -> [w2912]
              frame #0 {
                n1074 = Wait (ms)(milliseconds to wait=35) -> ()  [unwired: 1 out]
              }
            }
            n1075 = call-poly <vilib>:"Wait for Move Complete.flx"("Poll Interval (20 ms)"=5, "error in (no error)"=w2892, "Axis or Vector Space"=w2891, "Board ID"=w2889) -> ("error out"=w2898:errorcluster)  [unwired: 4 in, 3 out]
            n1076 = property class="niScope"(reference=w2895, error in=w2898) -> (error out=w2883:errorcluster, "Records Done"=w2890:i32)  [unwired: 1 out]
            n1077 = Wait on Notification(notifier=w2881, timeout in ms (-1)=5) -> (timed out?=w2879:bool)  [unwired: 2 in, 3 out]
            n1078 = case shown="No Error" w2883 {
              selector: w2883 -> [w2904 _]
              tunnel: w2894 -> [w2910 _]
              tunnel: [w2908 w2911] -> w2886
              tunnel: w2884 -> [w2905 w2911]
              frame No Error {
                n1079 = Lossy Enqueue Element(queue=w2905, element=w2910, error in (no error)=w2904) -> (queue out=w2909:refnum<queue>, error out=w2907:errorcluster)  [unwired: 2 out]
                n1080 = Get Queue Status(queue=w2909, error in (no error)=w2907) -> (queue out=w2908:refnum<queue>, # elements in queue=w2906:i32)  [unwired: 1 in, 6 out]
                n1081 = local write "Record queue"(w2906) -> ()
              }
              frame Error {
              }
            }
            n1082 = Not(x=w2879) -> (.not. x?=w2880:bool)
            n1083 = Not(x=w2897) -> (.not. x?=w2902:bool)
          }
          n1084 = while {
            tunnel: w2798 -> [w2843]
            tunnel: w2793 -> [w2842]
            tunnel: w2781 -> [w2840]
            tunnel: w2786 -> [w2841]
            shift-right: [w2838] -> _
            shift-left: _ -> [w2839]
            tunnel: [w2820] -> _
            tunnel: w2797 -> [w2833]
            tunnel: i16[] [1, 1, 1, 1, 2, 2, 2, 2, 2, 2] -> [w2832]
            tunnel: 10 -> [w2831]
            tunnel: w2795 -> [w2830]
            tunnel: [w2829] -> _
            tunnel: w2790 -> [_]
            tunnel: [w2828] -> w2789
            shift-right: [w2823] -> _
            shift-left: TRUE -> [w2827]
            tunnel: w2785 -> [w2825]
            tunnel: [w2823] -> w2784
            tunnel: w2777 -> [w2821]
            stop <- w2824 stop-if-true
            n1085 = Dequeue Element(queue=w2843, timeout in ms (-1)=w2821) -> (element=w2834:i8[][])  [unwired: 1 in, 3 out]
            n1086 = Multiply(x=w2830, y=w2831) -> (x*y=w2835:i32)
            n1087 = Reshape Array(w2834, w2842, w2835) -> (w2836:i8[][])
            n1088 = for {
              N: w2831 -> [_]
              tunnel: w2833 -> [w2851]
              tunnel: [w2854] -> w2837
              tunnel: w2840 -> [w2853]
              shift-right: [w2846] -> _
              shift-left: w2836 -> [w2856]
              tunnel: w2830 -> [w2845]
              tunnel: w2832 -> [w2844] mode=indexing
              i -> [w2852]
              n1089 = Index Array(array=w2851, index=w2852) -> (element=w2850:T17)
              n1090 = Delete From Array(array=w2856, length=w2845, index (col)=0 ("disabled index (col)")) -> (deleted portion=w2849:i8[], array with subset deleted=w2846:i8[][])  [unwired: 1 in]
              n1091 = for {
                tunnel: w2849 -> [w2859] mode=indexing
                tunnel: [w2858] -> w2848 mode=indexing
                n1092 = call-poly <vilib>:"Mean.vi"("X"=w2859) -> ("mean"=w2860:dbl)  [unwired: 1 out]
                n1093 = To Word Integer(number=w2860) -> (16bit integer=w2857:i16)
                n1094 = Subtract(x=w2859, y=w2857) -> (x-y=w2858:i16)
              }
              n1095 = call-poly "TimeShiftDataPoly.vi"("output cluster"=w2850, "Array In"=w2848) -> ("Array Out"=w2855:i16[][])  [unwired: 2 in]
              n1096 = in-place {
                in-place-border: w2855 -> [w2862]
                in-place-border: w2844 -> [w2863]
                n1097 = in-place-dvr #25(w2853) -> (w2864:i16[][])  [unwired: 1 out]
                n1098 = case shown="2" w2863 {
                  selector: w2863 -> [_ w2867]
                  tunnel: w2862 -> [w2866 w2869]
                  tunnel: [w2866 w2868] -> w2861
                  frame 0, Default {
                  }
                  frame 2 {
                    n1099 = Multiply(x=w2867, y=w2869) -> (x*y=w2868:i16[][])
                  }
                }
                n1100 = Add(x=w2861, y=w2864) -> (x+y=w2865:i16[][])
                n1101 = in-place-dvr #25(w2865) -> (w2854:refnum<data-value>)  [unwired: 1 out]
              }
            }
            n1102 = in-place {
              in-place-border: w2841 -> [w2878]
              in-place-border: [w2875] -> w2829
              in-place-border: w2827 -> [w2873]
              in-place-border: 0 -> [w2870]
              n1103 = in-place-dvr #26(w2837) -> (w2874:i16[][])  [unwired: 1 out]
              n1104 = Bundle(0.0, w2873, w2874, w2870) -> (w2871:cluster{dbl, bool, i16[][], i32})  [unwired: 1 in]
              n1105 = Multiply(x=i16 0, y=w2874) -> (x*y=w2877:i16[][])
              n1106 = Lossy Enqueue Element(queue=w2878, element=w2871) -> (queue out=w2875:refnum<queue>)  [unwired: 1 in, 3 out]
              n1107 = in-place-dvr #26(w2877) -> (w2828:refnum<data-value>)  [unwired: 1 out]
            }
            n1108 = Wait on Notification(notifier=w2825, timeout in ms (-1)=5) -> (timed out?=w2822:bool)  [unwired: 2 in, 3 out]
            n1109 = Tick Count (ms)() -> (millisecond timer value=w2838:u32)
            n1110 = Not(x=w2827) -> (.not. x?=w2823:bool)
            n1111 = Not(x=w2822) -> (.not. x?=w2824:bool)
            n1112 = Subtract(x=w2838, y=w2839) -> (x-y=w2820:u32)
            n1113 = local write "SF Loop"(w2820) -> ()
          }
          n1114 = node-c288(w2806) -> ()
          n1115 = Compound Arithmetic op=AND(w2783, w2784) -> (w2782:bool)
          n1116 = Release Queue(queue=w2811, force destroy? (F)=w2782) -> ()  [unwired: 1 in, 3 out]
          n1117 = call <instrlib>:"niScope Abort.vi"("instrument handle"=w2791) -> ()  [unwired: 13 in, 2 out]
          n1118 = Delete Data Value Reference(data value reference=w2789) -> ()  [unwired: 1 in, 2 out]
          n1119 = Release Queue(queue=w2810, force destroy? (F)=w2782) -> ()  [unwired: 1 in, 3 out]
        }
        frame "Drop Ch 5 (3 Trig)" {
          w2980 = 2 ("index")
          w2993 = 5
          # "Reduced data case that drop ring 5 receive using rcv on 3,4,5"
          # "Restructure file names"
          # "Read queue and send to files. About same as reading channel by channel"
          n1120 = Array To Cluster(array=w2965) -> (cluster=w2966:cluster{"[0]":void, "[1]":void, "[2]":void})
          n1121 = Reshape Array(w2994, w2993, w2993) -> (w2978:T19)
          n1122 = Unbundle(w2966) -> ("[0]"=w2964, "[1]"=w2963)  [unwired: 1 out]
          n1123 = Array Subset(array=w2978, index (row)=2 ("index"), index (col)=w2980, length (col)=w2980) -> (w2979:T19)  [unwired: 1 in]
          n1124 = Array Subset(array=w2978, length (col)=2 ("index")) -> (w2982:T19)  [unwired: 3 in]
          n1125 = Obtain Queue(max queue size (-1, unlimited)=2, element data type=w2959) -> (queue out=w2996:refnum<queue>)  [unwired: 3 in, 2 out]
          n1126 = Build Array(w2964, w2963) -> (w2975:void[])
          n1127 = Reshape Array(w2982, 10) -> (w2981:T20)
          n1128 = Reshape Array(w2979, 6) -> (w2989:T20)
          n1129 = expression code="x*5"(w2971) -> (w2974:dbl)
          n1130 = expression code="x*3"(w2971) -> (w2970:dbl)
          n1131 = Build Array(w2981, w2989) -> (w2988:T19)
          n1132 = while {
            tunnel: w2996 -> [w3020]
            tunnel: w2977 -> [w3019]
            tunnel: w2971 -> [w3018]
            tunnel: w2967 -> [w3015]
            tunnel: w2969 -> [w3017]
            tunnel: w2988 -> [w3010]
            tunnel: i32[] [10, 6] -> [w3014]
            shift-right: [w3012] -> _
            shift-left: _ -> [w3013]
            tunnel: [w3011] -> _
            tunnel: w2961 -> [w3006]
            tunnel: i16[] [1, 1, 1, 1, 2, 2, 2, 2, 2, 2] -> [w3005]
            tunnel: [w3004] -> w2976
            tunnel: w2968 -> [w3002]
            tunnel: [w3000] -> w2962
            tunnel: w2958 -> [w2997]
            stop <- w3000 stop-if-true
            n1133 = for {
              tunnel: w3019 -> [w3034]
              tunnel: w3018 -> [w3045]
              tunnel: w3020 -> [w3048]
              tunnel: [w3044] -> w3009 mode=indexing
              tunnel: [w3043] -> w3016
              tunnel: [w3042] -> w3007
              tunnel: w3015 -> [w3041]
              tunnel: w3010 -> [_] mode=indexing
              tunnel: w3014 -> [w3038]
              tunnel: w3010 -> [w3040]
              tunnel: w3006 -> [w3037]
              tunnel: w3005 -> [w3033]
              tunnel: [w3030] -> w2999 mode=indexing
              tunnel: w2997 -> [w3029]
              n1134 = Dequeue Element(queue=w3048, timeout in ms (-1)=w3037) -> (element=w3047:T12)  [unwired: 1 in, 3 out]
              n1135 = Unbundle(w3047) -> ("gain"=w3043:dbl, "wfm"=w3046:i8[][], w3044:bool, "max queue size (-1, unlimited)"=w3035:i32)
              n1136 = Index Array(array=w3038, index=w3035) -> (element=w3036:i32)
              n1137 = Index Array(array=w3040, index (row)=w3035) -> (element=w3039:T20)  [unwired: 1 in]
              n1138 = Multiply(x=w3034, y=w3036) -> (x*y=w3032:i32)
              n1139 = Reshape Array(w3046, w3045, w3032) -> (w3031:i8[][])
              n1140 = for {
                N: w3036 -> [_]
                tunnel: w3039 -> [w3058]
                tunnel: [w3061] -> w3042
                tunnel: w3041 -> [w3060]
                shift-right: [w3054] -> _
                shift-left: w3031 -> [w3062]
                tunnel: w3033 -> [w3056] mode=indexing
                tunnel: w3034 -> [w3055]
                tunnel: [w3050] -> w3030 mode=indexing
                tunnel: w3029 -> [w3049]
                i -> [w3059]
                n1141 = Index Array(array=w3058, index=w3059) -> (element=w3051:T17)
                n1142 = Delete From Array(array=w3062, length=w3055, index (col)=0 ("disabled index (col)")) -> (deleted portion=w3053:i8[], array with subset deleted=w3054:i8[][])  [unwired: 1 in]
                n1143 = call "TimeShiftDataSubMean.vi"("Filter"=w3049, "output cluster"=w3051, "Array In"=w3053) -> ("Array Out"=w3052:i16[][], "Sat Pts"=w3050:i32)  [unwired: 2 in]
                n1144 = in-place {
                  in-place-border: w3052 -> [w3064]
                  in-place-border: w3056 -> [w3065]
                  n1145 = in-place-dvr #27(w3060) -> (w3066:i16[][])  [unwired: 1 out]
                  n1146 = case shown="2" w3065 {
                    selector: w3065 -> [_ w3069]
                    tunnel: w3064 -> [w3068 w3071]
                    tunnel: [w3068 w3070] -> w3063
                    frame 0, Default {
                    }
                    frame 2 {
                      n1147 = Multiply(x=w3069, y=w3071) -> (x*y=w3070:i16[][])
                    }
                  }
                  n1148 = Add(x=w3063, y=w3066) -> (x+y=w3067:i16[][])
                  n1149 = in-place-dvr #27(w3067) -> (w3061:refnum<data-value>)  [unwired: 1 out]
                }
              }
            }
            n1150 = Wait on Notification(notifier=w3002, timeout in ms (-1)=5) -> (timed out?=w3001:bool)  [unwired: 2 in, 3 out]
            n1151 = Or Array Elements(Boolean array=w3009) -> (logical OR=w3008:bool)
            n1152 = Add Array Elements(numeric array=w2999) -> (sum=w2998:i32)
            n1153 = in-place {
              in-place-border: w3017 -> [w3028]
              in-place-border: w3008 -> [w3027]
              in-place-border: w3016 -> [w3026]
              in-place-border: w2998 -> [w3021]
              n1154 = in-place-dvr #28(w3007) -> (w3022:i16[][])  [unwired: 1 out]
              n1155 = Bundle("gain"=w3026, w3027, w3022, "Sat Pts"=w3021) -> (w3025:T21)  [unwired: 1 in]
              n1156 = Multiply(x=i16 0, y=w3022) -> (x*y=w3024:i16[][])
              n1157 = Lossy Enqueue Element(queue=w3028, element=w3025) -> ()  [unwired: 1 in, 4 out]
              n1158 = in-place-dvr #28(w3024) -> (w3004:refnum<data-value>)  [unwired: 1 out]
            }
            n1159 = Not(x=w3001) -> (.not. x?=w3000:bool)
            n1160 = Tick Count (ms)() -> (millisecond timer value=w3012:u32)
            n1161 = Subtract(x=w3012, y=w3013) -> (x-y=w3011:u32)
          }
          n1162 = while {
            tunnel: w2975 -> [w3089]
            tunnel: w2996 -> [w3088]
            tunnel: w2963 -> [w3087]
            tunnel: w2977 -> [w3086]
            tunnel: [w3085] -> w2991
            tunnel: w2990 -> [w3084]
            shift-right: [w3072] -> _
            shift-left: _ -> [w3083]
            tunnel: [w3082] -> _
            tunnel: "0,1" -> [w3081]
            tunnel: w2974 -> [w3080]
            tunnel: w2970 -> [w3079]
            tunnel: w2968 -> [w3077]
            tunnel: w2960 -> [w3074]
            stop <- w3076 stop-if-true
            n1163 = for {
              tunnel: w3086 -> [w3104]
              tunnel: w3089 -> [w3106] mode=indexing
              tunnel: w3081 -> [w3105]
              tunnel: w3088 -> [w3103]
              tunnel: w3087 -> [w3100]
              tunnel: [w3098] -> w3085
              tunnel: w3084 -> [w3095]
              tunnel: w3080 -> [w3097]
              tunnel: w3079 -> [w3096]
              tunnel: w3074 -> [w3094]
              tunnel: [w3091] -> w3073
              i -> [w3093]
              # "Read data"
              n1164 = case shown="0" w3093 {
                tunnel: w3106 -> [w3113 w3122]
                tunnel: w3105 -> [w3111 w3121]
                tunnel: w3104 -> [w3114 w3126]
                tunnel: [w3115 w3125] -> w3102
                tunnel: [w3108 w3120] -> w3101
                tunnel: [w3116 w3124] -> _
                tunnel: w3100 -> [w3117 _]
                tunnel: [w3112 _] -> w3099
                tunnel: w3095 -> [w3110 _]
                tunnel: w3097 -> [_ _]
                tunnel: w3096 -> [_ w3118]
                tunnel: w3094 -> [w3107 _]
                frame 0 {
                  # "Read files and queue it up."
                  n1165 = call <instrlib>:"niScope Initiate Acquisition.vi"("instrument handle"=w3117) -> ("error out"=w3109:errorcluster)  [unwired: 2 in, 12 out]
                  n1166 = call "Rapid Read_NI.vi"("NI Card"=w3113, "Channel"=w3111, "Motion Board ID"=w3110, "rf points per line"=w3114, "error in"=w3109, "Pause?"=w3107) -> ("dig gain"=w3115:dbl, "Array"=w3108:i8[][], "Reverse?"=w3112:bool, "error out"=w3116:errorcluster)  [unwired: 6 in]
                }
                frame 1, Default {
                  n1167 = property class="niScope"(reference=w3122, "Fetch Record Number"=0 ("Fetch:Fetch Record Number"), "Fetch Number of Records"=w3118) -> (reference out=w3127:refnum<k15>, error out=w3123:errorcluster)  [unwired: 1 in]
                  n1168 = call-poly <instrlib>:"niScope Fetch (poly).vi"("error in"=w3123, "numSamples"=w3126, "channels"=w3121, "instrument handle"=w3127) -> ("error out"=w3124:errorcluster, "wfm"=w3120:i8[][], "wfm info"=w3129:T22)  [unwired: 1 in, 4 out]
                  n1169 = Index Array(array=w3129) -> (element=w3128:T23)  [unwired: 1 in]
                  n1170 = Unbundle By Name(w3128) -> ("gain"=w3125:dbl)
                }
              }
              n1171 = Bundle("gain"=w3102, "wfm"=w3101, "Reverse?"=w3099, w3093) -> (w3092:T24)  [unwired: 1 in]
              n1172 = Enqueue Element(queue=w3103, element=w3092) -> (queue out=w3098:refnum<queue>, error out=w3091:errorcluster)  [unwired: 2 in, 1 out]
            }
            n1173 = Wait on Notification(notifier=w3077, timeout in ms (-1)=5) -> (timed out?=w3075:bool)  [unwired: 2 in, 3 out]
            n1174 = flat-sequence {
              tunnel: [w3090] -> w3072
              tunnel: w3073 -> [_]
              frame #0 {
                n1175 = Tick Count (ms)() -> (millisecond timer value=w3090:u32)
              }
            }
            n1176 = Not(x=w3075) -> (.not. x?=w3076:bool)
            n1177 = Subtract(x=w3072, y=w3083) -> (x-y=w3082:u32)
          }
          n1178 = Release Queue(queue=w2991, force destroy? (F)=w2962) -> ()  [unwired: 1 in, 3 out]
          n1179 = Delete Data Value Reference(data value reference=w2976) -> ()  [unwired: 1 in, 2 out]
        }
      }
    }
    frame #5 {
      n1180 = Cancel Notification(0:w3131) -> ()  [unwired: 1 in, 3 out]
      n1181 = case shown="\"Hawaii\", Default" w3132 {
        frame "Hawaii", Default {
          # "turn off real time trig. Back to motion trig"
          n1182 = call-poly <vilib>:"DAQmx Write.vi"("task/channels in"=refnum<k21> "DIO-L2 L3", "data"=bool[] [TRUE, FALSE]) -> ()  [unwired: 11 in, 3 out]
        }
        frame "UHI Allen", "CUMC RT" {
        }
      }
      n1183 = case shown="4" w3130 {
        tunnel: w3133 -> [_ w3134]
        frame 0, Default {
        }
        frame 4 {
          n1184 = for {
            tunnel: w3134 -> [w3137] mode=indexing
            n1185 = call <vilib>:"DAQmx Stop Task.vi"("task/channels in"=w3137) -> ("task out"=w3136:refnum<k21>, "error out"=w3135:errorcluster)  [unwired: 13 in]
            n1186 = call <vilib>:"DAQmx Clear Task.vi"("task in"=w3136, "error in"=w3135) -> ()  [unwired: 13 in, 1 out]
          }
        }
      }
    }
  }
  n1187 = case shown="0, Default" w7 {
    tunnel: w33 -> [w3158 _]
    tunnel: w32 -> [w3157 _]
    tunnel: w31 -> [w3156 _]
    tunnel: w30 -> [w3155 _]
    tunnel: w29 -> [w3154 _]
    tunnel: w28 -> [w3153 _]
    tunnel: w27 -> [w3152 _]
    tunnel: w26 -> [w3151 _]
    tunnel: w15 -> [w3140 _]
    frame 0, Default {
      # "Return to start location and reset to original value"
      n1188 = case shown="\"Full 25 Ch\", Default" w3153 {
        tunnel: w3157 -> [w3160 w3165]
        tunnel: w3156 -> [_ w3168]
        tunnel: w3155 -> [w3159 w3162]
        tunnel: [w3160 w3167] -> w3149
        tunnel: [w3159 w3166] -> w3148
        tunnel: w3140 -> [_ w3161]
        frame "1T/5R Deep Mem", "Deep Memory 2 CH" {
        }
        frame "Full 25 Ch", Default {
          n1189 = call-poly <vilib>:"Wait for Move Complete.flx"("error in (no error)"=w3162, "Axis or Vector Space"=w3161, "Board ID"=w3165) -> ("error out"=w3163:errorcluster, "Bd ID Out"=w3164:T5)  [unwired: 5 in, 2 out]
          n1190 = call <vilib>:"Stop Program.flx"("error in (no error)"=w3163, "Program (1)"=w3168, "Board ID"=w3164) -> ("error out"=w3166:errorcluster, "Bd ID Out"=w3167:T5)  [unwired: 4 out]
        }
      }
      n1191 = call "MoveMotor.vi"("error in (no error)"=w3148, "Target Position (0)"=w3154, "Axis or Vector Space"=w3158, "Motion Bd ID"=w3149) -> ("error out"=w3142:errorcluster, "Resource Output"=w3141:u16, "Bd ID Out"=w3143:u8)  [unwired: 1 in, 4 out]
      n1192 = call "Load Acceleration/Deceleration.flx"("Acceleration (100000)"=w3151, "error in (no error)"=w3142, "Axis or Vector Space"=w3141, "Board ID"=w3143) -> ("error out"=w3146:errorcluster, "Resource Output"=w3144:T27, "Bd ID Out"=w3145:T5)  [unwired: 1 in, 2 out]
      n1193 = call <vilib>:"Load Velocity.flx"("Velocity (10000)"=w3152, "error in (no error)"=w3146, "Axis or Vector Space"=w3144, "Board ID"=w3145) -> ("error out"=→"error out":errorcluster, "Bd ID Out"=→"Bd ID Out":T5)  [unwired: 4 out]
    }
    frame 8 {
    }
  }
